vi "TL_XY_PFS_sCMOS_v8.vi"() -> ()   [LabVIEW 2013]
uses:
  <vilib>/Analysis/Matrix/Datatypes/RealMatrix.ctl
  <vilib>/Platform/TimedLoop/XDataNode/timing_clust.ctl
  <vilib>/Platform/TimedLoop/XDataNode/nitl_modes.ctl
  <vilib>/Platform/TimedLoop/XDataNode/wakeup.ctl
  <vilib>/DAQmx/read.llb/DAQmx Read (Analog DBL 1Chan 1Samp).vi
  <vilib>/DAQmx/write.llb/DAQmx Write (Analog DBL 1Chan 1Samp).vi
  <vilib>/DAQmx/write.llb/DAQmx Write (Digital 1D Bool 1Chan 1Samp).vi
  <vilib>/DAQmx/create/channels.llb/DAQmx Create Channel (AO-Voltage-Basic).vi
  <vilib>/DAQmx/create/channels.llb/DAQmx Create Channel (DO-Digital Output).vi
  <vilib>/Platform/TimedLoop/scheduler/LVUserAPI/_suppVIs/Create_1kHz_TSource.vi
  <vilib>/DAQmx/create/channels.llb/DAQmx Create Channel (AI-Voltage-Basic).vi
  <vilib>/DAQmx/miscellaneous.llb/DAQmx Fill In Error Info.vi
  <vilib>/Analysis/Matrix/Numeric/Conversions/Array To Matrix - RA.vi
  <vilib>/Platform/TimedLoop/XDataNode/XDataNode.xnode
  <vilib>/Platform/TimedLoop/XDataNode/XDNodeRunTimeDep.lvlib
  <vilib>/Analysis/Matrix/NI_Matrix.lvlib
panel:
  out "lastgoodz_list":T1
  in  "Delay after Fluo. cube change":u32=500
  in  "Delay PFS":u32=500
  out "lastgoodz":i32
  out "PFS status":i32
  in  "Delay after Move":u32=500
  out "TL_NPOS":u32 caption="Number of\nPositions"
  out "Laser Power (a.u.)":dbl=50.0 format="%05_2f"
  out "FlowRate (mL/min)":dbl=50.0 format="%05_2f"
  in  "Min. Scan duration":dbl
  out "TL Fluidic SYNC":bool caption="Fluidic SYNC"
  out "softversion":string
  in  "config Name":string="your_config"
  in  "Load Config":bool
  in  "Save Config":bool
  in  "Config Directory":path=path "D:/CONFIG_TIME_LAPSE"
  out "TL Laser shutter":bool caption="L. shutter"
  out "Next Pattern":u8(slide) scale=0.0..100.0
  out "Recorded\nPatterns":u32
  out "Ready":bool
  in  "stop the program":bool
  out "Current Position":u32
  out "Y position (µm)":dbl
  out "X position (µm)":dbl
  in  "storeXY Position":bool
  in  "stage speed (mm/s)":sgl=5.0 min=0.1 max=5 step=0.1
  in  "Stage COM PORT":refnum<visa-resource-name>="COM1"
  out "Next Scan":u8(slide) scale=0.0..100.0
  in  "Frames between Scan":u32
  out "Recorded Scans":u32
  in  "Total Number of Scan":u32=150 step=1
  out "TLON":bool
  in  "pause TL":bool
  in  "startTL":bool
  in  "Lower Filter":u8=1 min=1 max=6 step=1
  out "Buffer Info":T2
  out "Version":string
  out "Camera Serial":string
  out "Camera Model":string
  in  "Binning":u16=1 max=4 step=1
  out "zinit":i32
  in  "file name motif":string="image"
  out "SavedImages":i32
  out "Next Image Name":string
  out "Z position":dbl
  in  "error in (no error)":errorcluster
  out "Read Out Time":dbl=50.0
  in  "RO Mode":u32 max=2 step=1
  out "Imtemp":u16[][](array[numeric])
  in  "savelast":bool
  in  "Current Directory":path=path "D:/DATA_Par_Dates"
  in  "Exposure Time":dbl=0.1 min=0.0 max=10.0 step=9.999999747378752e-06
  in  "Time between Images (Free Run)":u32 caption="delay"
  in  "LASER shutter":bool
  in  "Free Run":bool
  in  "Commande onglets":T3(tab)
  out "Intensity Graph":u16[][](graph)
  in  "RESET ALL\nChanels":bool
  in  "ADD\nChanel":bool
  out "used Filters":u8[](array[numeric])
  out "used LEDs":bool[][](array[boolean])
  in  "LED-0":bool
  in  "LED-1":bool
  in  "LED-2":bool
  in  "LED-3":bool
  in  "LED-4":bool
  in  "LED-5":bool
  in  "Filter selection":u8(ring)=1 items=["1"=1, "2"=2, "3"=3, "4"=4, "5"=5, "6"=6]
  in  "LED-6":bool
  in  "LED-7":bool
  in  "LED-8":bool
  in  "LED-9":bool
  in  "LED-10":bool
  in  "LED-11":bool
  out "TL_NCAN":u8
  in  "Generate\nPositions":bool
  out "Field\nHeigth (µm)":dbl
  out "Field\nWidth (µm)":dbl
  out "stored XY":T1
  in  "re-SET ALL\nPositions":bool
  in  "XY positions path":path
  in  "Loadpositions":bool
  out "Scanning Motif":T4(graph)
  in  "Microscope Objective\nMagnification":dbl=60.0 min=1.0 max=1000.0 step=1.0
  in  "Method":u8(ring) items=["Spiral Scan", "Column Scan", "Line Scan"]
  in  "Spacing X (µm)":dbl=100.0 step=0.001
  in  "Spacing Y (µm)":dbl=100.0 step=0.001
  in  "Number\nof\nPositions":u32=40
  in  "Position to add":u32=30 step=1
  in  "Noff":u32 step=1
  in  "Non":u32=150 step=1
  in  "Nstart":u32=30 step=1
  in  "Frames between Patterns":u32
  in  "Total Number of Patterns":u32=1 step=1
  in  "is_single_shoot":bool caption="SingleShoot/TemporalPattern"
  in  "Shoot duration":dbl=1.0 step=1.0
  out "shooted_ positions":bool[][](array[boolean])
  in  "ADD\nPosition":bool
  in  "ADD ALL\nPositions":bool
  in  "RESET POS":bool
  out "shoot_list":T1
  in  "Shoot at Scan#":i32=1 step=1
  in  "useLASER_TL":bool caption="use LASER"
  in  "Noff FLUIDICS":u32 caption="Noff" step=1
  in  "Non FLUIDICS":u32=150 caption="Non" step=1
  in  "Nstart FLUIDICS":u32=30 caption="Nstart" step=1
  in  "useFLUIDICS_TL":bool caption="use LASER"
  # "XY stage"
  # "(µm)"
  # "Camera Settings"
  # "(s)"
  # "(s)"
  # "Time Lapse"
  # "Timming Settings"
  # "(s)"
  # "(ms)"
  # "(ms)"
  # "(ms)"
  # "Set a Illumination Pattern"
  # "Number of Channels"
  # "Light Sources to use"
  # "340\nnm"
  # "365\nnm"
  # "405\nnm"
  # "455\nnm"
  # "490\nnm"
  # "505\nnm"
  # "565\nnm"
  # "590\nnm"
  # "625\nnm"
  # "680\nnm"
  # "730\nnm"
  # "Bright\nField"
  # "0"
  # "1"
  # "2"
  # "Channel   #"
  # "3"
  # "4"
  # "5"
  # "6"
  # "7"
  # "8"
  # "Stored Positions"
  # "SingleShoot Mode"
  # "TemporalPattern Mode"
  # "Timming"
  # "Timming"
  # "(s)"
  # "FLUIDIC Switch Timming (SCAN Mode)"
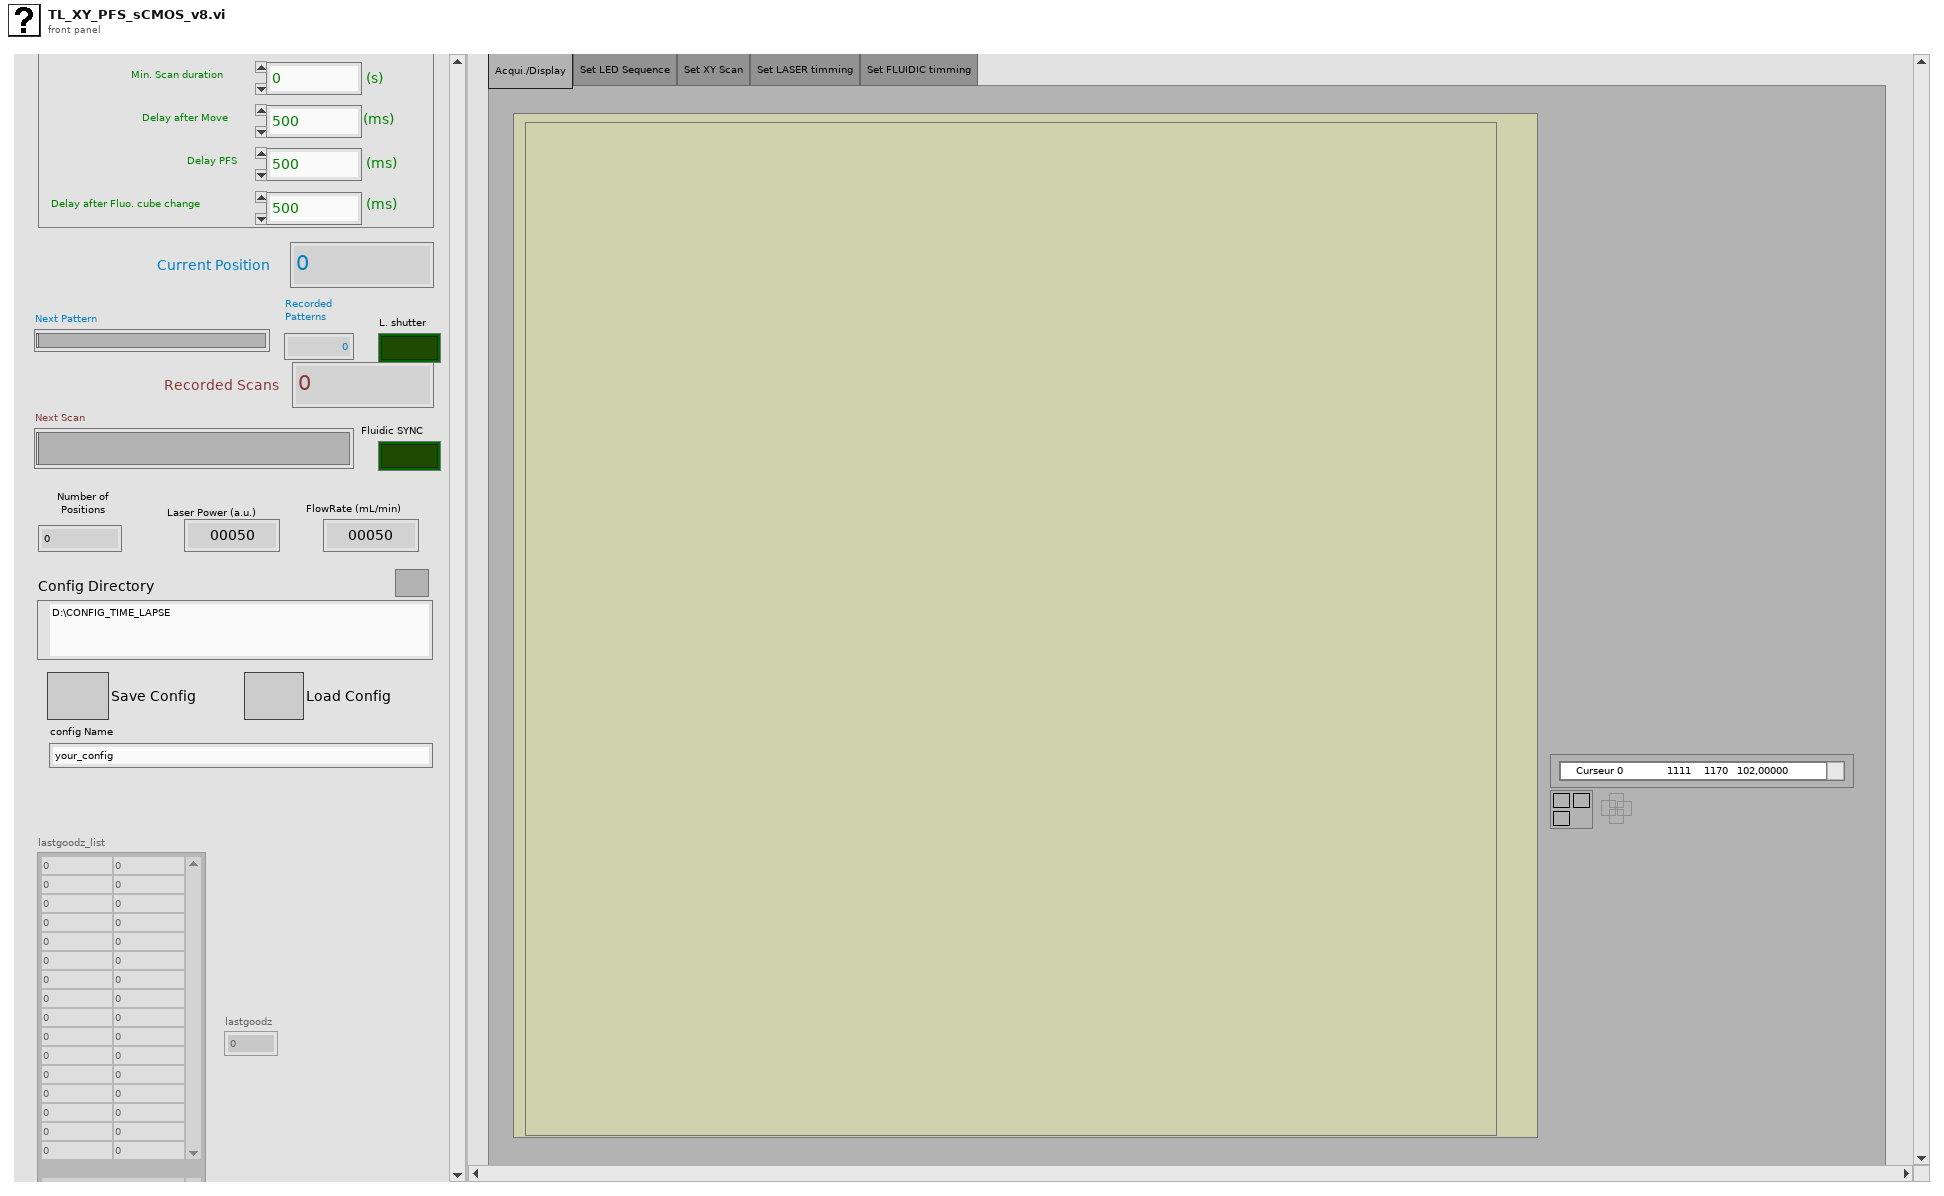
[diagram p1: front panel]
types:
  T1 = typedef "NI_Matrix.lvlib/RealMatrix.ctl" = dbl[][]
  T2 = cluster{"height":u32, "width":u32, "datatype":u32}
  T3 = enum32{"Acqui./Display", "Set LED Sequence", "Set XY Scan", "Set LASER timming", "Set FLUIDIC timming"}
  T4 = cluster{cluster{"Real Matrix Element":dbl, "Real Matrix Element":dbl}[]}[]
  T5 = cluster{"Model":string, "Camera ID":string, "Firmware":string}
  T6 = cluster{"Mode":u32, "Polarity":u32, "Times":u32, "Delay":dbl}
  T7 = typedef "XDNodeRunTimeDep.lvlib/timing_clust.ctl" = cluster{"Expected End [f-1]":u64, "Actual End [f-1]":u64, "Finished Late? [f-1]":bool, "Expected End [i-1]":u64, "Actual End [i-1]":u64, "Finished Late? [i-1]":bool, "Expected Start [i]":u64, "Actual Start [i]":u64, "Expected Start [f]":u64, "Actual Start [f]":u64, "Source Name":string, "Structure Name":string, "Period":i64, "Deadline":i64, "Offset":i64, "Start":i64, "Priority":i32, "Timeout":i32, "Mode":T8, "Wakeup Reason":T9, "Error":errorcluster, "Source Type":string, "Secondary Source Type":string, "Global End Time":u64, "Global Start Time":u64, "Frame Duration":u64, "Iteration Duration":u64, "Assigned CPU":i32, "I/O Scan Engine Mode":u32}
  T8 = typedef "XDNodeRunTimeDep.lvlib/nitl_modes.ctl" = enum32{"No Change", "Process missed periods, maintain original phase", "Discard missed periods, maintain original phase", "Process missed periods, ignore original phase", "Discard missed periods, ignore original phase"}
  T9 = typedef "XDNodeRunTimeDep.lvlib/wakeup.ctl" = enum32{"Normal", "Aborted", "Asynchronous wakeup", "Timing source error", "Timed loop error", "Timeout"}
  T10 = typedef "Image Type" = u32
  T11 = typedef "IMAQ Image.ctl" = refnum<image>
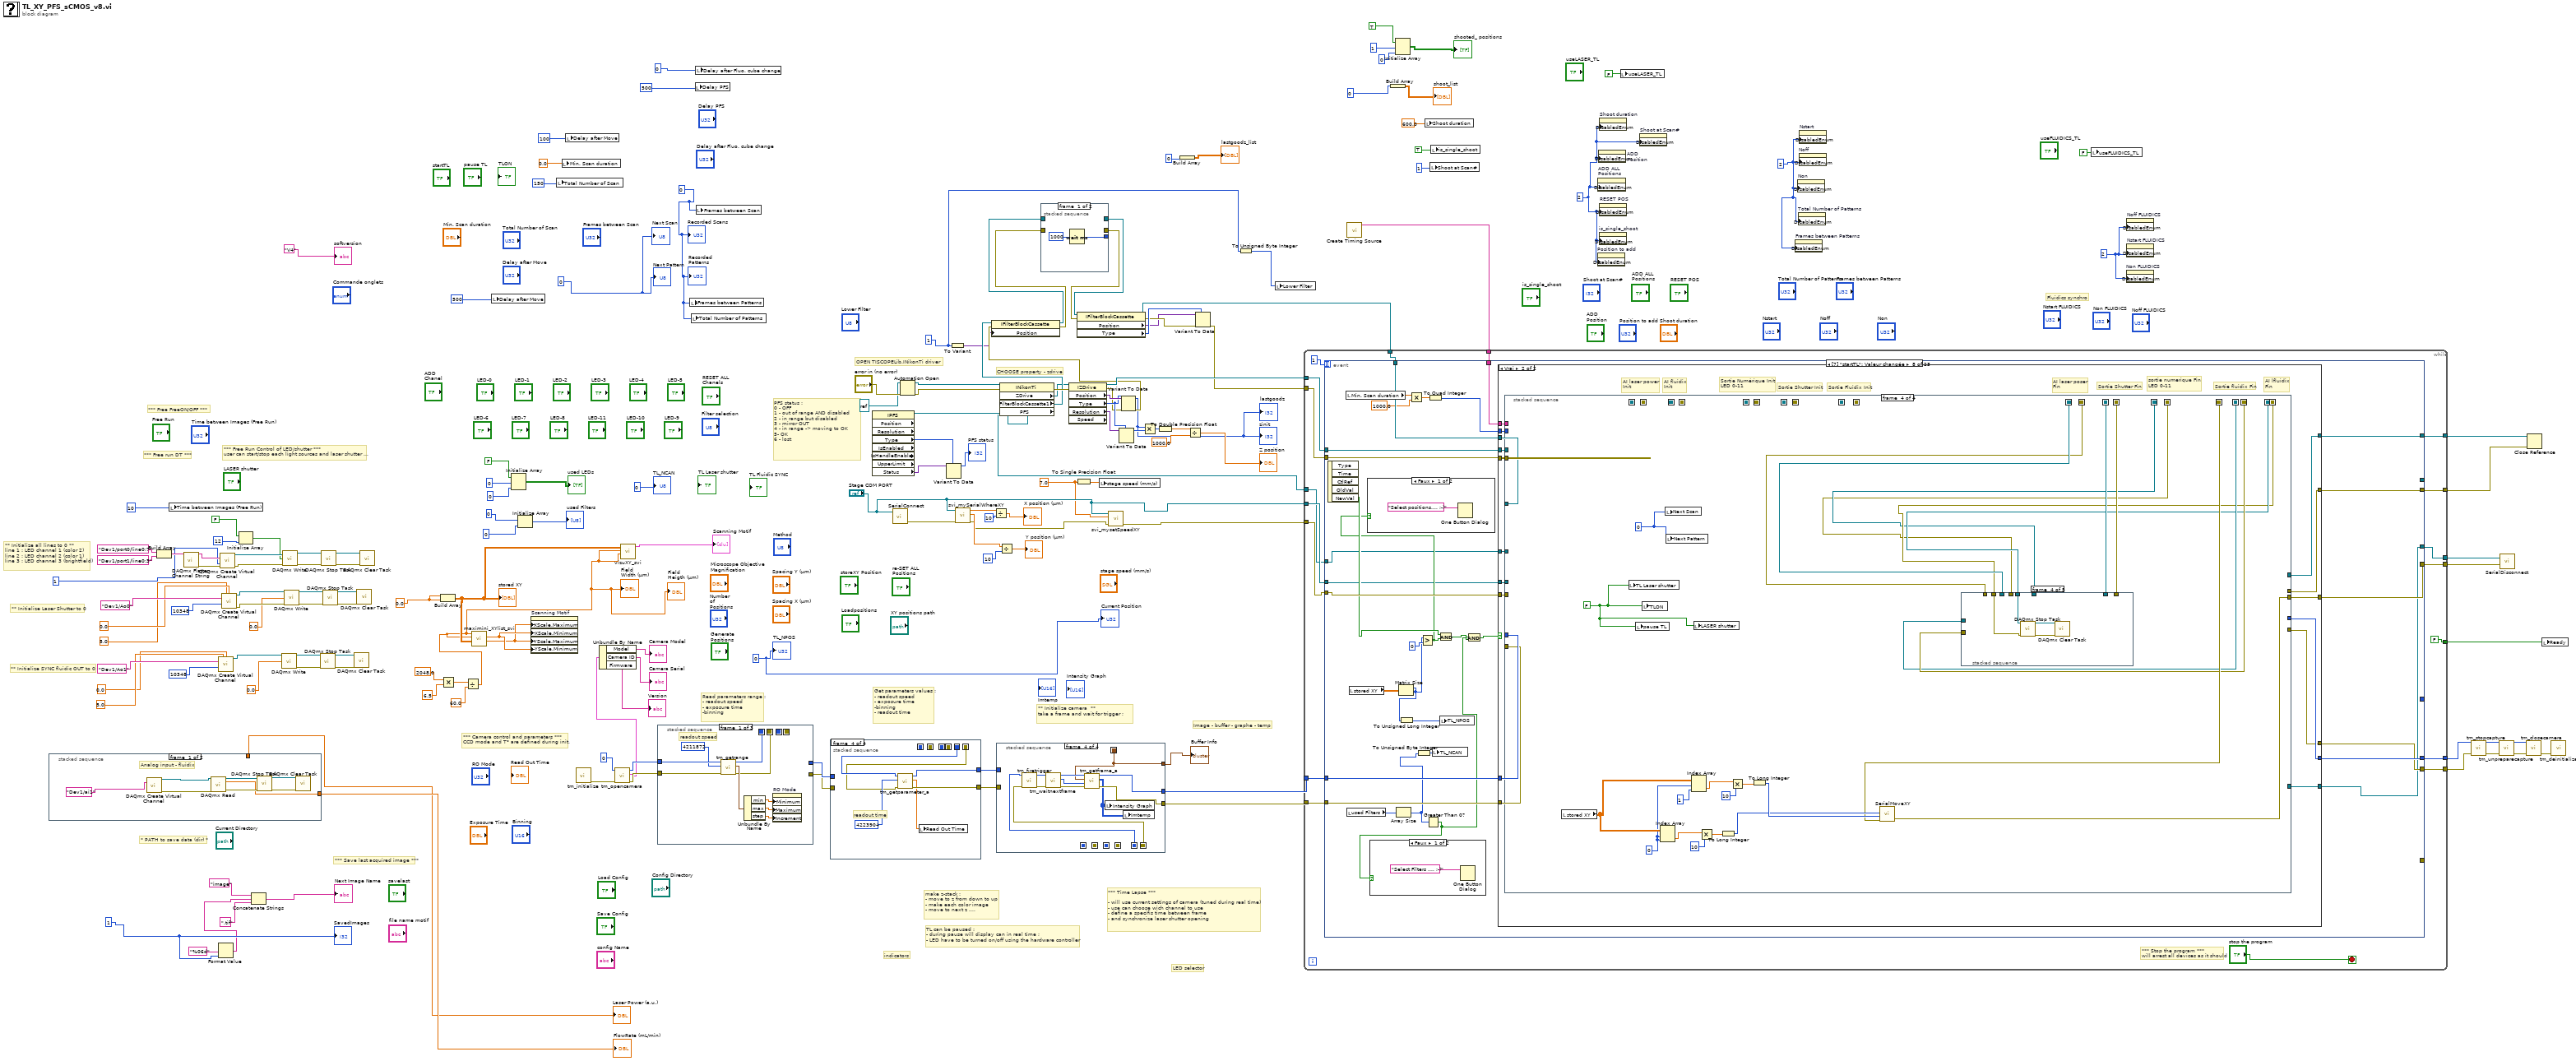
[diagram p0: block diagram]
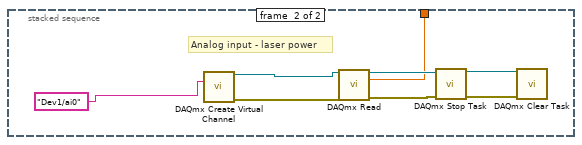
[diagram p2: hidden frame]
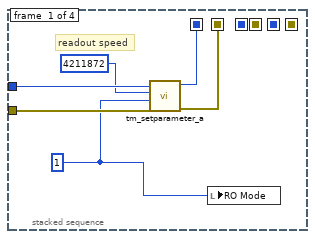
[diagram p4: hidden frame]
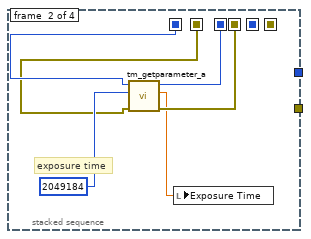
[diagram p5: hidden frame]
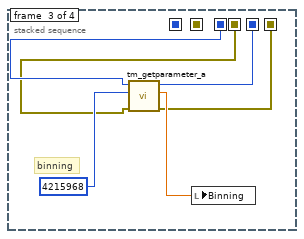
[diagram p6: hidden frame]
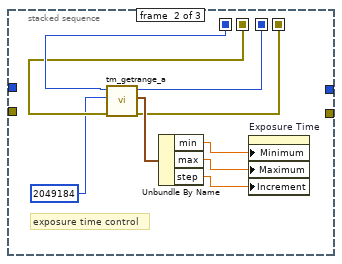
[diagram p7: hidden frame]
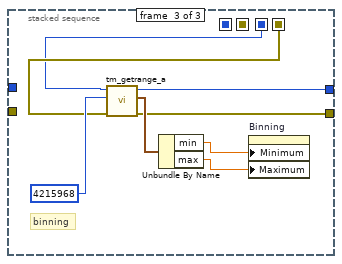
[diagram p8: hidden frame]
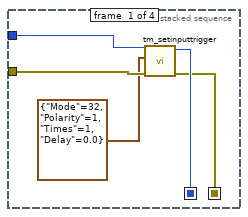
[diagram p9: hidden frame]
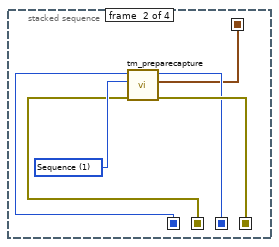
[diagram p10: hidden frame]
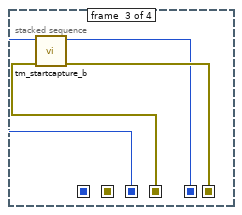
[diagram p11: hidden frame]
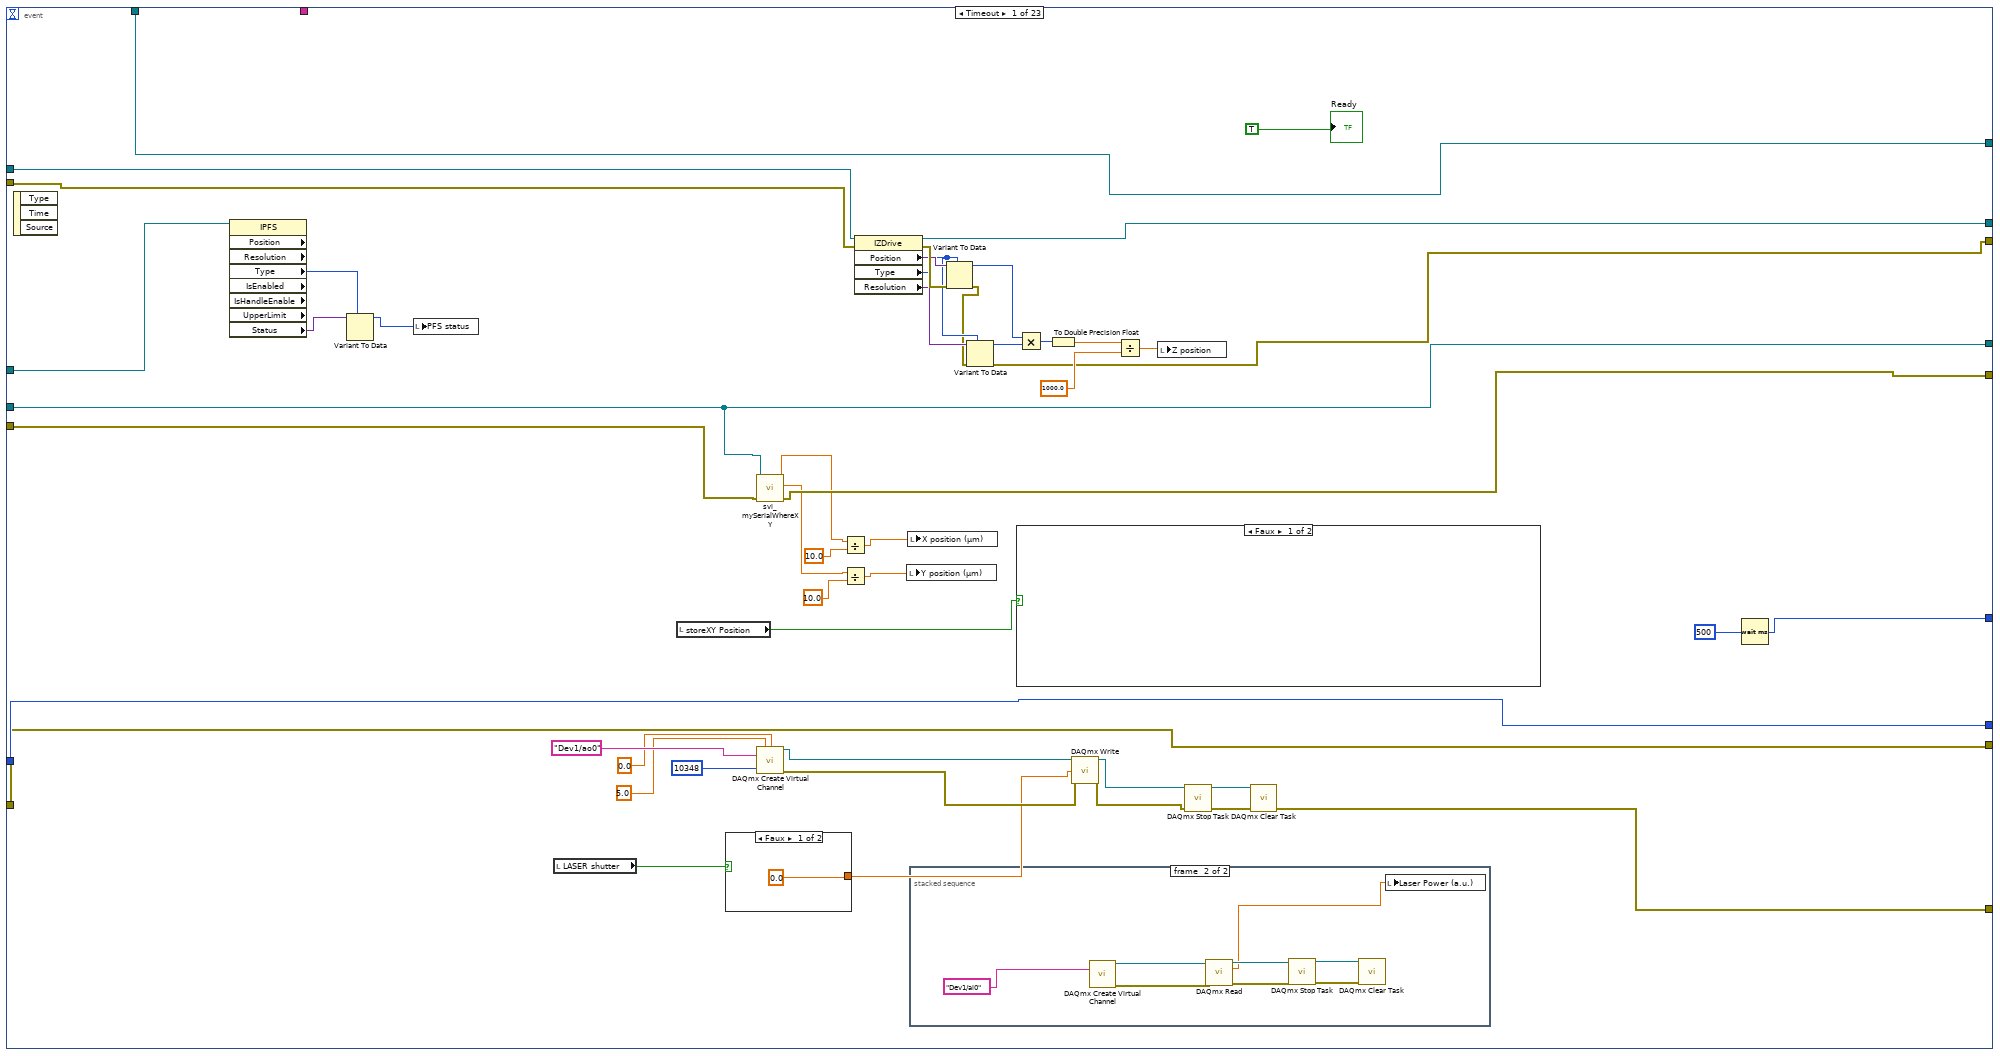
[diagram p12: hidden frame]
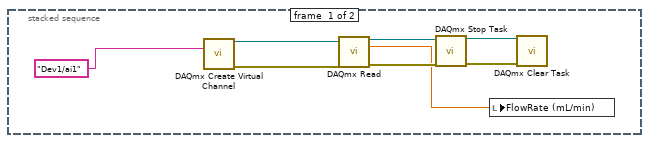
[diagram p13: hidden frame]
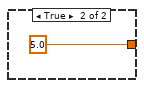
[diagram p14: hidden frame]
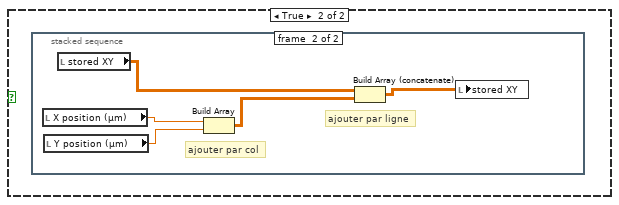
[diagram p15: hidden frame]
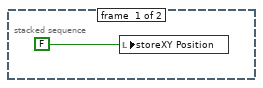
[diagram p16: hidden frame]
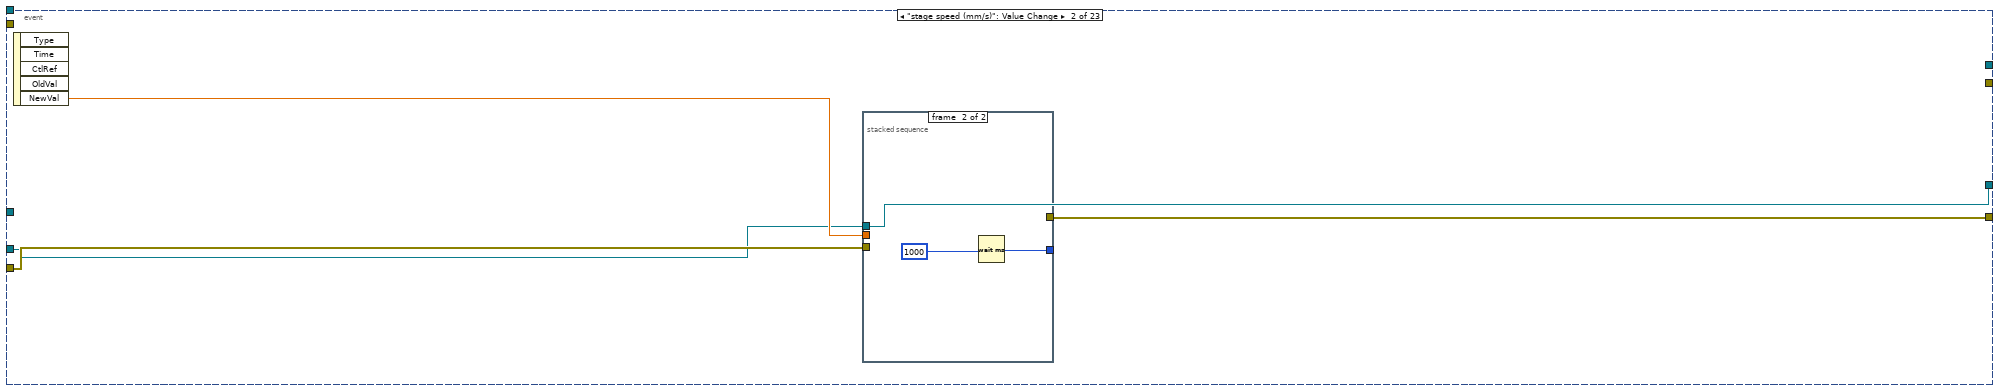
[diagram p17: hidden frame]
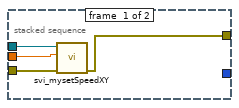
[diagram p18: hidden frame]
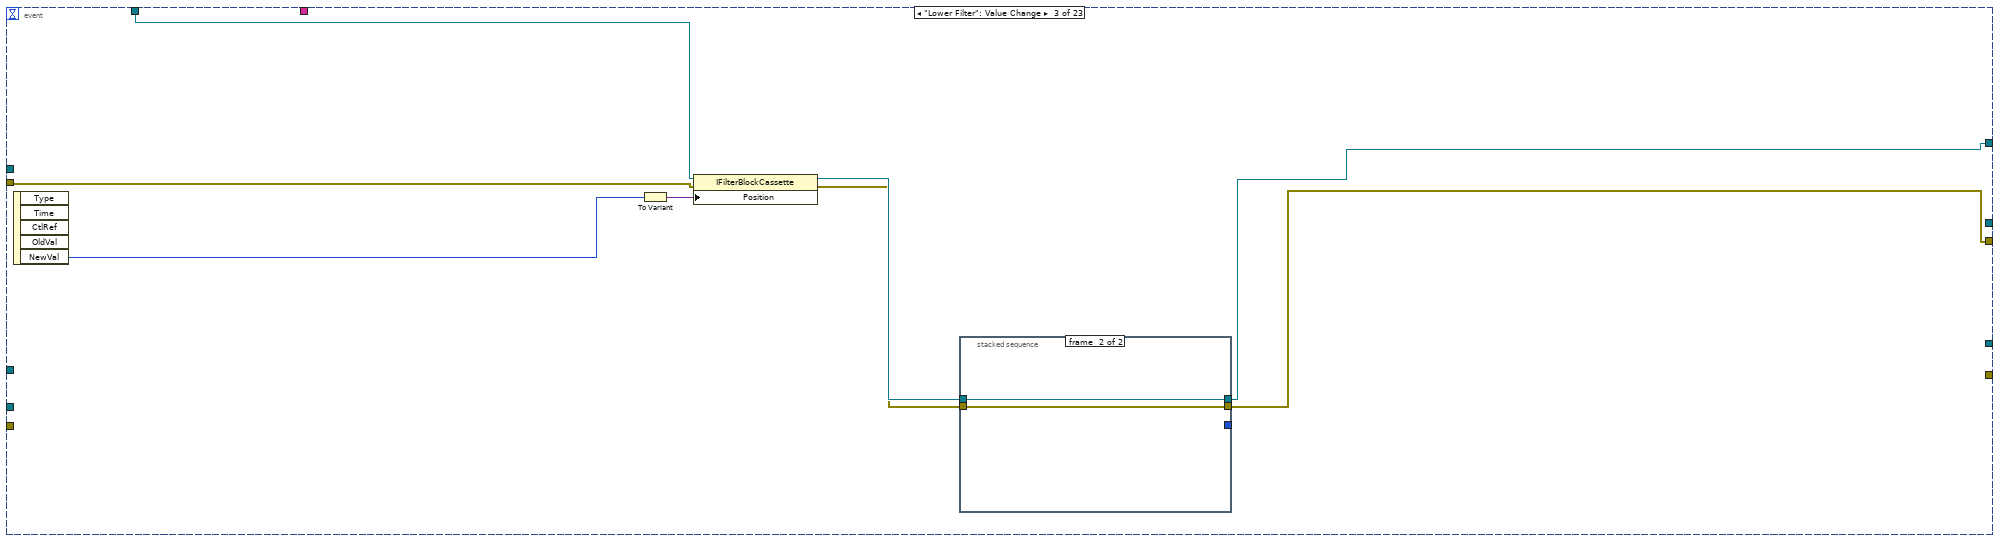
[diagram p19: hidden frame]
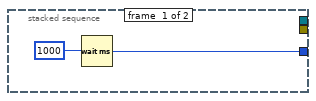
[diagram p20: hidden frame]
diagram:
  w16 = u8 2
  w15 = u8 2
  w24 = u8 2
  w56 = 0
  w58 = u32 0
  w59 = u8 0
  w60 = 0.0
  w92 = 7.0
  w41 = 1
  w132 = 1
  # "PFS status :\n0 - OFF\n1 - out of range AND disabled\n2 - in range but disabled\n3 - mirror OUT\n4 - in range -> moving to OK\n5- OK\n6 - lost"
  # "Fluidics synchro"
  # "** Initialize SYNC fluidic OUT to 0"
  # "** Initialize Laser Shutter to 0"
  # "* PATH to save data (dir) *"
  # "Image - buffer - graphe - temp"
  # "Get parameters values :\n- readout speed\n- exposure time\n-binning\n- readout time"
  # "Read parameters range :\n- readout speed\n- exposure time\n-binning"
  # "CHOOSE property - zdrive"
  # "OPEN TISCOPELib.INikonTi driver"
  # "indicators"
  # "LED selector"
  # "TL can be paused :\n- during pause will display can in real time ;\n- LED have to be turned on/off using the hardware controller"
  # "make z-stack :\n- move to z from down to up\n- make each color image\n- move to next z ...."
  # "*** Time Lapse ***\n\n- will use current settings of camera (tuned during real time)\n- use can choose wich channel to use\n- define a specifis time between frame\n- and synchronize laser shutter opening"
  # "*** Camera control and parameters ***\nCCD mode and T° are defined during init."
  # "*** Save last acquired image ***"
  # "** Initialize camera  **\ntake a frame and wait for trigger ;"
  # "** Initialize all lines to 0 **\nline 1 : LED channel 1 (color 2)\nline 2 : LED channel 2 (color 1)\nline 3 : LED channel 3 (brightfield)"
  # "*** Free FreeON/OFF ***"
  # "*** Free run DT ***"
  # "*** Free Run Control of LED/shutter ***\nuser can start/stop each light sources and laser shutter ..."
  n1 = stacked-sequence {
    tunnel: [w166 _] -> w20
    tunnel: [_ w174] -> w13
    frame #0 {
      # "Analog input - fluidix"
      n2 = call-poly <vilib>:"DAQmx Create Virtual Channel.vi"("physical channels"="Dev1/ai1") -> ("task out"=w173:refnum<k21>, "error out"=w172:errorcluster)  [unwired: 13 in]
      n3 = call-poly <vilib>:"DAQmx Read.vi"("task/channels in"=w173, "error in"=w172) -> ("task out"=w170:refnum<k21>, "data"=w166:dbl, "error out"=w171:errorcluster)  [unwired: 11 in]
      n4 = call <vilib>:"DAQmx Stop Task.vi"("task/channels in"=w170, "error in"=w171) -> ("task out"=w168:refnum<k21>, "error out"=w169:errorcluster)  [unwired: 12 in]
      n5 = call <vilib>:"DAQmx Clear Task.vi"("task in"=w168, "error in"=w169) -> ()  [unwired: 13 in, 1 out]
    }
    frame #1 {
      # "Analog input - laser power"
      n6 = call-poly <vilib>:"DAQmx Create Virtual Channel.vi"("physical channels"="Dev1/ai0") -> ("task out"=w175:refnum<k21>, "error out"=w176:errorcluster)  [unwired: 13 in]
      n7 = call-poly <vilib>:"DAQmx Read.vi"("task/channels in"=w175, "error in"=w176) -> ("task out"=w178:refnum<k21>, "data"=w174:dbl, "error out"=w177:errorcluster)  [unwired: 11 in]
      n8 = call <vilib>:"DAQmx Stop Task.vi"("task/channels in"=w178, "error in"=w177) -> ("task out"=w180:refnum<k21>, "error out"=w179:errorcluster)  [unwired: 12 in]
      n9 = call <vilib>:"DAQmx Clear Task.vi"("task in"=w180, "error in"=w179) -> ()  [unwired: 13 in, 1 out]
    }
  }
  "Laser Power (a.u.)" <- w13
  "FlowRate (mL/min)" <- w20
  n10 = Build Array("Dev1/port0/line0:7", "Dev1/port1/line0:3") -> (w83:string[])
  n11 = local write "Time between Images (Free Run)"(10) -> ()
  n12 = call <vilib>:"DAQmx Flatten Channel String.vi"("names in"=w83) -> ("names out"=w82:string, "error out"=w84:errorcluster)  [unwired: 13 in]
  n13 = Format Value(format string="%06d", value (0)=w132) -> (output string=w131:string)  [unwired: 1 in]
  n14 = call-poly <vilib>:"DAQmx Create Virtual Channel.vi"("maximum value"=5.0, "minimum value"=0.0, "physical channels"="Dev1/Ao1", "units"=10348) -> ("task out"=w38:refnum<k21>)  [unwired: 10 in, 1 out]
  n15 = call-poly <vilib>:"DAQmx Create Virtual Channel.vi"("lines"=w82, "line grouping"=1, "error in"=w84) -> ("task out"=w164:refnum<k21>, "error out"=w163:errorcluster)  [unwired: 11 in]
  n16 = call-poly <vilib>:"DAQmx Create Virtual Channel.vi"("maximum value"=5.0, "minimum value"=0.0, "physical channels"="Dev1/Ao0", "units"=10348) -> ("task out"=w80:refnum<k21>, "error out"=w79:errorcluster)  [unwired: 10 in]
  n17 = Initialize Array(FALSE, 12) -> (w109:bool[])
  n18 = Concatenate Strings("image", w131, ".tif") -> (→"Next Image Name":string)
  n19 = call-poly <vilib>:"DAQmx Write.vi"("task/channels in"=w38, "data"=0.0) -> ("task out"=w37:refnum<k21>, "error out"=w36:errorcluster)  [unwired: 11 in, 1 out]
  n20 = call-poly <vilib>:"DAQmx Write.vi"("task/channels in"=w164, "data"=w109, "error in"=w163) -> ("task out"=w162:refnum<k21>, "error out"=w160:errorcluster)  [unwired: 10 in, 1 out]
  n21 = call-poly <vilib>:"DAQmx Write.vi"("task/channels in"=w80, "data"=0.0, "error in"=w79) -> ("task out"=w76:refnum<k21>, "error out"=w77:errorcluster)  [unwired: 10 in, 1 out]
  n22 = call <vilib>:"DAQmx Stop Task.vi"("task/channels in"=w37, "error in"=w36) -> ("task out"=w34:refnum<k21>, "error out"=w35:errorcluster)  [unwired: 12 in]
  n23 = call <vilib>:"DAQmx Stop Task.vi"("task/channels in"=w162, "error in"=w160) -> ("task out"=w161:refnum<k21>, "error out"=w159:errorcluster)  [unwired: 12 in]
  n24 = call <vilib>:"DAQmx Stop Task.vi"("task/channels in"=w76, "error in"=w77) -> ("task out"=w75:refnum<k21>, "error out"=w74:errorcluster)  [unwired: 12 in]
  n25 = call <vilib>:"DAQmx Clear Task.vi"("task in"=w34, "error in"=w35) -> ()  [unwired: 13 in, 1 out]
  n26 = call <vilib>:"DAQmx Clear Task.vi"("task in"=w75, "error in"=w74) -> ()  [unwired: 13 in, 1 out]
  n27 = call <vilib>:"DAQmx Clear Task.vi"("task in"=w161, "error in"=w159) -> ()  [unwired: 13 in, 1 out]
  n28 = Build Array(w60, w60) -> (w52:T1)
  "stored XY" <- w52
  n29 = Multiply(x=2048.0, y=6.5) -> (x*y=w48:dbl)
  n30 = Divide(x=w48, y=60.0) -> (x/y=w47:dbl)
  "Field\nWidth (µm)" <- w47
  "Field\nHeigth (µm)" <- w47
  n31 = call "maximini_XYlist_svi.vi"("stored XY"=w52, "LY"=w47, "LX"=w47) -> ("mini (µm)"=w54:dbl, "maxi (µm)"=w53:dbl)  [unwired: 7 in]
  n32 = local write "Delay after Move"(u32 500) -> ()
  n33 = Initialize Array(FALSE, 0, 0) -> (→"used LEDs":bool[][])
  n34 = Initialize Array(u8 0, 0) -> (→"used Filters":u8[])
  n35 = property on="Scanning Motif" class="GraphXY (strict)"("XScale.Maximum"=w53, "XScale.Minimum"=w54, "YScale.Maximum"=w53, "YScale.Minimum"=w54) -> ()  [unwired: 2 in, 2 out]
  n36 = local write "Total Number of Scan"(u32 150) -> ()
  n37 = local write "Min. Scan duration"(0.0) -> ()
  n38 = local write "Delay after Move"(u32 100) -> ()
  n39 = call <userlib>:"tm_initialize.vi"() -> ("error out"=w158:errorcluster)  [unwired: 1 in, 10 out]
  n40 = call <userlib>:"tm_opencamera.vi"("error in (no error)"=w158, "Camera Index"=u32 0) -> ("error out"=w129:errorcluster, "Camera Details"=w119:T5, "Handle out"=w130:u32)  [unwired: 1 in, 6 out]
  n41 = Unbundle By Name(w119) -> ("Model"=→"Camera Model":string, "Camera ID"=→"Camera Serial":string, "Firmware"=→"Version":string)
  n42 = call "vizuXY_svi.vi"("LY (mm)"=w47, "LX (mm)"=w47, "stored XY (µm)"=w52) -> ("Tableau"=→"Scanning Motif":T4)  [unwired: 8 in]
  n43 = stacked-sequence {
    seq-local: [w183 _ _] -> [_ w199 _]
    seq-local: [w182 _ _] -> [_ w198 _]
    seq-local: [_ w192 _] -> [_ _ w203]
    seq-local: [_ w191 _] -> [_ _ w204]
    tunnel: w130 -> [w190 _ _]
    tunnel: w129 -> [w189 _ _]
    tunnel: [_ _ w202] -> w128
    tunnel: [_ _ w201] -> w127
    frame #0 {
      # "readout speed"
      n44 = call <userlib>:"tm_getrange.vi"("error in (no error)"=w189, "Parameter"=4211872, "Handle in"=w190) -> ("error out"=w182:errorcluster, "Range"=w187:cluster{"min":dbl, "max":dbl, "step":dbl}, "Handle out"=w183:u32)  [unwired: 6 out]
      n45 = Unbundle By Name(w187) -> ("min"=w186:dbl, "max"=w185:dbl, "step"=w184:dbl)
      n46 = property on="RO Mode" class="NumNb (strict)"("Minimum"=w186, "Maximum"=w185, "Increment"=w184) -> ()  [unwired: 2 in, 2 out]
    }
    frame #1 {
      # "exposure time control"
      n47 = call <userlib>:"tm_getrange_a.vi"("error in (no error)"=w198, "Parameter"=2049184, "Handle in"=w199) -> ("error out"=w191:errorcluster, "Range"=w197:cluster{"min":dbl, "max":dbl, "step":dbl}, "Handle out"=w192:u32)  [unwired: 2 in, 4 out]
      n48 = Unbundle By Name(w197) -> ("min"=w196:dbl, "max"=w195:dbl, "step"=w194:dbl)
      n49 = property on="Exposure Time" class="NumNb (strict)"("Minimum"=w196, "Maximum"=w195, "Increment"=w194) -> ()  [unwired: 2 in, 2 out]
    }
    frame #2 {
      # "binning"
      n50 = call <userlib>:"tm_getrange_a.vi"("error in (no error)"=w204, "Parameter"=4215968, "Handle in"=w203) -> ("error out"=w201:errorcluster, "Range"=w207:cluster{"min":dbl, "max":dbl, "step":dbl}, "Handle out"=w202:u32)  [unwired: 2 in, 4 out]
      n51 = Unbundle By Name(w207) -> ("min"=w200:dbl, "max"=w206:dbl)
      n52 = property on="Binning" class="NumNb (strict)"("Minimum"=w200, "Maximum"=w206) -> ()  [unwired: 2 in, 2 out]
    }
  }
  n53 = local write "Frames between Patterns"(w58) -> ()
  n54 = local write "Total Number of Patterns"(w58) -> ()
  n55 = local write "Delay PFS"(u32 500) -> ()
  n56 = local write "Delay after Fluo. cube change"(u32 0) -> ()
  n57 = local write "Frames between Scan"(w58) -> ()
  n58 = stacked-sequence {
    seq-local: [w210 _ _ _] -> [_ w218 _ _]
    seq-local: [w209 _ _ _] -> [_ w217 _ _]
    seq-local: [_ w216 _ _] -> [_ _ w223 _]
    seq-local: [_ w215 _ _] -> [_ _ w222 _]
    seq-local: [_ _ w221 _] -> [_ _ _ w230]
    seq-local: [_ _ w220 _] -> [_ _ _ w229]
    tunnel: w128 -> [w213 _ _ _]
    tunnel: w127 -> [w212 _ _ _]
    tunnel: [_ _ _ w228] -> w126
    tunnel: [_ _ _ w227] -> w125
    frame #0 {
      w208 = 1
      # "readout speed"
      n59 = call <userlib>:"tm_setparameter_a.vi"("error in (no error)"=w212, "Value in"=w208, "Parameter"=4211872, "Handle in"=w213) -> ("error out"=w209:errorcluster, "Handle out"=w210:u32)  [unwired: 6 in]
      n60 = local write "RO Mode"(w208) -> ()
    }
    frame #1 {
      # "exposure time"
      n61 = call <userlib>:"tm_getparameter_a.vi"("error in (no error)"=w217, "Parameter"=2049184, "Handle in"=w218) -> ("error out"=w215:errorcluster, "Value out"=w214:dbl, "Handle out"=w216:u32)  [unwired: 6 in]
      n62 = local write "Exposure Time"(w214) -> ()
    }
    frame #2 {
      # "binning"
      n63 = call <userlib>:"tm_getparameter_a.vi"("error in (no error)"=w222, "Parameter"=4215968, "Handle in"=w223) -> ("error out"=w220:errorcluster, "Value out"=w224:dbl, "Handle out"=w221:u32)  [unwired: 6 in]
      n64 = local write "Binning"(w224) -> ()
    }
    frame #3 {
      # "readout time"
      n65 = call <userlib>:"tm_getparameter_a.vi"("error in (no error)"=w229, "Parameter"=4223904, "Handle in"=w230) -> ("error out"=w227:errorcluster, "Value out"=w226:dbl, "Handle out"=w228:u32)  [unwired: 6 in]
      n66 = local write "Read Out Time"(w226) -> ()
    }
  }
  n67 = call "SerialConnect.vi"("VISA resource name"="Stage COM PORT") -> ("error out"=w108:errorcluster)  [unwired: 4 in]
  n68 = Automation Open(error in (no error)="error in (no error)", Automation Refnum=refnum<k7> refnum ("TISCOPELib.INikonTi")) -> (Automation Refnum=w145:refnum<k7>, error out=w144:errorcluster)  [unwired: 2 out]
  n69 = To Variant(anything=w41) -> (Variant=w110:variant)
  n70 = call "svi_mySerialWhereXY.vi"("entrée d'erreur (pas d'erreur)"=w108, "Refnum VISA en entrée"="Stage COM PORT") -> ("sortie d'erreur"=w101:errorcluster, "Y"=w104:dbl, "X"=w107:dbl)  [unwired: 7 in]
  n71 = Divide(x=w107, y=10) -> (x/y=→"X position (µm)":dbl)
  n72 = stacked-sequence {
    seq-local: [w233 _ _ _] -> [_ w241 _ _]
    seq-local: [w232 _ _ _] -> [_ w240 _ _]
    seq-local: [_ w238 _ _] -> [_ _ w246 _]
    seq-local: [_ w239 _ _] -> [_ _ w245 _]
    seq-local: [_ _ w243 _] -> [_ _ _ w255]
    seq-local: [_ _ w244 _] -> [_ _ _ w254]
    seq-local: [_ w237 _ _] -> [_ _ _ w248]
    tunnel: w126 -> [w236 _ _ _]
    tunnel: w125 -> [w235 _ _ _]
    tunnel: [_ _ _ w250] -> w124
    tunnel: [_ _ _ w249] -> w123
    tunnel: [_ _ _ w248] -> w152
    frame #0 {
      n73 = call <userlib>:"tm_setinputtrigger.vi"("error in (no error)"=w235, "Parameters"=T6 {"Mode"=32, "Polarity"=1, "Times"=1, "Delay"=0.0}, "Handle in"=w236) -> ("error out"=w232:errorcluster, "Handle out"=w233:u32)  [unwired: 7 in]
    }
    frame #1 {
      w242 = 1 items=["Snap", "Sequence"] ("Capture mode")
      n74 = call <userlib>:"tm_preparecapture.vi"("error in (no error)"=w240, "Capture mode"=w242, "Handle in"=w241) -> ("error out"=w239:errorcluster, "Buffer Info"=w237:T2, "Handle out"=w238:u32)  [unwired: 5 in, 1 out]
    }
    frame #2 {
      n75 = call <userlib>:"tm_startcapture_b.vi"("error in (no error)"=w245, "Handle in"=w246) -> ("error out"=w244:errorcluster, "Handle out"=w243:u32)  [unwired: 8 in]
    }
    frame #3 {
      n76 = call <userlib>:"tm_firetrigger.vi"("error in (no error)"=w254, "Handle in"=w255) -> ("error out"=w257:errorcluster, "Handle out"=w256:u32)  [unwired: 8 in]
      n77 = call <userlib>:"tm_waitnextframe.vi"("error in (no error)"=w257, "Handle in"=w256) -> ("error out"=w252:errorcluster, "Frame Index"=w251:i32, "Handle out"=w253:u32)  [unwired: 6 in, 1 out]
      n78 = call <userlib>:"tm_getframe_a.vi"("error in (no error)"=w252, "Frame Index"=w251, "Buffer Info"=w248, "Handle in"=w253) -> ("error out"=w249:errorcluster, "Data 16"=w247:u16[][], "Handle out"=w250:u32)  [unwired: 3 in, 2 out]
      n79 = local write "Intensity Graph"(w247) -> ()
      n80 = local write "Imtemp"(w247) -> ()
    }
  }
  "Buffer Info" <- w152
  n81 = Divide(x=w104, y=10) -> (x/y=→"Y position (µm)":dbl)
  n82 = property class="INikonTi"(reference=w145, error in=w144) -> (error out=w116:errorcluster, "ZDrive"=w89:refnum<k7>, "FilterBlockCassette1"=w112:refnum<k7>, "PFS"=w10:refnum<k7>)  [unwired: 1 out]
  n83 = property class="IPFS" props=["Position", "Resolution", "Type", "IsEnabled", "IsHandleEnable", "UpperLimit", "Status"](reference=w10) -> (reference out=w6:refnum<k7>, "Type"=w9:i32, "Status"=w7:variant)  [unwired: 1 in, 6 out]
  n84 = Variant To Data(type=w9, Variant=w7) -> (data=→"PFS status":i32)  [unwired: 1 in, 1 out]
  n85 = property class="IZDrive" props=["Position", "Type", "Resolution", "Speed"](reference=w89, error in=w116) -> (reference out=w143:refnum<k7>, error out=w139:errorcluster, "Position"=w142:variant, "Type"=w140:i32, "Resolution"=w141:variant)  [unwired: 1 out]
  n86 = To Single Precision Float(number=w92) -> (single precision float=w93:sgl)
  n87 = local write "stage speed (mm/s)"(w93) -> ()
  n88 = call "svi_mysetSpeedXY.vi"("entrée d'erreur (pas d'erreur)"=w101, "speed (mm/s)"=w92, "Refnum VISA en entrée"="Stage COM PORT") -> ("sortie d'erreur"=w99:errorcluster)  [unwired: 8 in]
  n89 = Variant To Data(type=w140, Variant=w141) -> (data=w138:i32)  [unwired: 1 in, 1 out]
  n90 = Variant To Data(error in=w139, type=w140, Variant=w142) -> (data=w5:i32, error out=w111:errorcluster)
  "zinit" <- w5
  "lastgoodz" <- w5
  n91 = property class="IFilterBlockCassette"(reference=w112, error in=w111, "Position"=w110) -> (reference out=w46:refnum<k7>, error out=w45:errorcluster)
  n92 = stacked-sequence {
    tunnel: [w258 _] -> _
    tunnel: w46 -> [_ w261]
    tunnel: w45 -> [_ w260]
    tunnel: [_ w261] -> w44
    tunnel: [_ w260] -> w43
    frame #0 {
      n93 = Wait (ms)(milliseconds to wait=1000) -> (millisecond timer value=w258:u32)
    }
    frame #1 {
    }
  }
  n94 = property class="IFilterBlockCassette"(reference=w44, error in=w43) -> (reference out=w115:refnum<k7>, error out=w117:errorcluster, "Position"=w113:variant, "Type"=w118:i32)
  n95 = Multiply(x=w5, y=w138) -> (x*y=w95:i32)
  n96 = To Double Precision Float(number=w95) -> (double precision float=w94:dbl)
  n97 = Build Array(0) -> (→"lastgoodz_list":T1)
  n98 = Divide(x=w94, y=1000.0) -> (x/y=→"Z position":dbl)
  n99 = Variant To Data(error in=w117, type=w118, Variant=w113) -> (error out=w64:errorcluster)  [unwired: 1 out]
  n100 = To Unsigned Byte Integer(number=w41) -> (unsigned 8bit integer=w90:u8)
  n101 = local write "Lower Filter"(w90) -> ()
  n102 = call-poly <vilib>:"Create Timing Source.vi"() -> ("name (out)"=w18:string)  [unwired: 10 in, 1 out]
  n103 = while {
    tunnel: [w277] -> w154
    tunnel: w124 -> [w276]
    tunnel: w123 -> [w275]
    tunnel: [w274] -> w153
    tunnel: w143 -> [w272]
    tunnel: w64 -> [w273]
    tunnel: [w271] -> w87
    tunnel: [FALSE] -> w134
    tunnel: w115 -> [w269]
    tunnel: [w268] -> w114
    tunnel: w99 -> [w267]
    tunnel: "Stage COM PORT" -> [w266]
    tunnel: [w265] -> w98
    tunnel: [w264] -> w97
    tunnel: w18 -> [w263]
    tunnel: w6 -> [w262]
    stop <- "stop the program" stop-if-true
    # "*** Stop the program ***\nwill arrest all devices as it should ..."
    n104 = event shown="[7] \"startTL\": Valeur changée" {
      selector: _ -> [_ _ _ _ _ _ _ _ _ _ _ _ _ _ _ _ _ _ _ _ _ _ _]
      dyn-events: _ -> [_ _ _ _ _ _ _ _ _ _ _ _ _ _ _ _ _ _ _ _ _ _ _]
      timeout: 1 -> [_ _ _ _ _ _ _ _ _ _ _ _ _ _ _ _ _ _ _ _ _ _ _]
      tunnel: [w326 _ _ w378 _ _ _ w540 _ _ _ w1701 w1741 w1779 _ _ _ _ _ _ _ w1907 _] -> w277
      tunnel: w276 -> [w326 _ _ w379 _ _ _ w539 _ _ _ w1737 w1776 w1815 _ _ _ _ _ _ _ w1912 _]
      tunnel: w275 -> [w325 _ _ w380 _ _ _ w538 _ _ _ w1736 w1775 w1814 _ _ _ _ _ _ _ w1911 _]
      tunnel: [w325 _ _ w377 _ _ _ w534 _ _ _ w1702 w1740 w1778 _ _ _ _ _ _ _ w1906 _] -> w274
      tunnel: w273 -> [w324 _ w368 _ _ _ _ w537 _ _ _ _ _ _ _ _ _ _ _ _ _ _ _]
      tunnel: w272 -> [w284 _ _ _ _ _ _ w536 _ _ _ _ _ _ _ _ _ _ _ _ _ _ _]
      tunnel: [w323 _ _ _ _ _ _ _ _ _ _ _ _ _ _ _ _ _ _ _ _ _ _] -> _
      tunnel: [w285 _ w362 _ _ _ _ w525 _ _ _ _ _ _ _ _ _ _ _ _ _ _ _] -> w271
      tunnel: w269 -> [w286 _ w367 _ _ _ _ w527 _ _ _ _ _ _ _ _ _ _ _ _ _ _ _]
      tunnel: [w286 _ w363 _ _ _ _ w526 _ _ _ _ _ _ _ _ _ _ _ _ _ _ _] -> w268
      tunnel: [w314 _ _ _ _ _ _ _ _ _ _ _ _ _ _ _ _ _ _ _ _ _ _] -> _
      tunnel: [w306 _ _ _ _ _ _ _ _ _ _ _ _ _ _ _ _ _ _ _ _ _ _] -> _
      tunnel: w267 -> [w305 w354 _ w376 _ _ _ w535 _ _ _ _ _ _ _ _ _ _ _ _ _ w1910 _]
      tunnel: w266 -> [w303 w353 _ w375 _ _ _ w517 _ _ _ _ _ _ _ _ _ _ _ _ _ w1904 _]
      tunnel: [w304 w352 _ w374 _ _ _ w533 _ _ _ _ _ _ _ _ _ _ _ _ _ w1908 _] -> w264
      tunnel: [w303 w353 _ _ _ _ _ w516 _ _ _ _ _ _ _ _ _ _ _ _ _ w1909 _] -> w265
      tunnel: w263 -> [_ _ _ _ _ _ _ w515 _ _ _ _ _ _ _ _ _ _ _ _ _ _ _]
      tunnel: w262 -> [w283 _ _ _ _ _ _ w510 _ _ _ _ _ _ _ _ _ _ _ _ _ _ _]
      event Timeout {
        n105 = event-data() -> ()  [unwired: 1 in, 3 out]
        n106 = property class="IPFS" props=["Position", "Resolution", "Type", "IsEnabled", "IsHandleEnable", "UpperLimit", "Status"](reference=w283) -> ("Type"=w281:i32, "Status"=w282:variant)  [unwired: 1 in, 7 out]
        n107 = Variant To Data(type=w281, Variant=w282) -> (data=w280:i32)  [unwired: 1 in, 1 out]
        n108 = local write "PFS status"(w280) -> ()
        n109 = local read "LASER shutter"() -> (w290:bool)
        n110 = local read "storeXY Position"() -> (w292:bool)
        n111 = case shown="Faux" w290 {
          tunnel: [0.0 5.0] -> w291
          frame False {
          }
          frame True {
          }
        }
        n112 = call "svi_mySerialWhereXY.vi"("entrée d'erreur (pas d'erreur)"=w305, "Refnum VISA en entrée"=w303) -> ("sortie d'erreur"=w304:errorcluster, "Y"=w300:dbl, "X"=w298:dbl)  [unwired: 7 in]
        n113 = call-poly <vilib>:"DAQmx Create Virtual Channel.vi"("maximum value"=5.0, "minimum value"=0.0, "physical channels"="Dev1/ao0", "units"=10348) -> ("task out"=w312:refnum<k21>, "error out"=w311:errorcluster)  [unwired: 10 in]
        n114 = Divide(x=w298, y=10.0) -> (x/y=w297:dbl)
        n115 = Divide(x=w300, y=10.0) -> (x/y=w299:dbl)
        n116 = property class="IZDrive"(reference=w284, error in=w324) -> (reference out=w323:refnum<k7>, error out=w322:errorcluster, "Position"=w321:variant, "Type"=w319:i32, "Resolution"=w320:variant)
        n117 = local write "Y position (µm)"(w299) -> ()
        n118 = local write "X position (µm)"(w297) -> ()
        n119 = stacked-sequence {
          frame #0 {
            n120 = call-poly <vilib>:"DAQmx Create Virtual Channel.vi"("physical channels"="Dev1/ai1") -> ("task out"=w328:refnum<k21>, "error out"=w335:errorcluster)  [unwired: 13 in]
            n121 = call-poly <vilib>:"DAQmx Read.vi"("task/channels in"=w328, "error in"=w335) -> ("task out"=w329:refnum<k21>, "data"=w331:dbl, "error out"=w334:errorcluster)  [unwired: 11 in]
            n122 = call <vilib>:"DAQmx Stop Task.vi"("task/channels in"=w329, "error in"=w334) -> ("task out"=w330:refnum<k21>, "error out"=w333:errorcluster)  [unwired: 12 in]
            n123 = local write "FlowRate (mL/min)"(w331) -> ()
            n124 = call <vilib>:"DAQmx Clear Task.vi"("task in"=w330, "error in"=w333) -> ()  [unwired: 13 in, 1 out]
          }
          frame #1 {
            n125 = call-poly <vilib>:"DAQmx Create Virtual Channel.vi"("physical channels"="Dev1/ai0") -> ("task out"=w337:refnum<k21>, "error out"=w338:errorcluster)  [unwired: 13 in]
            n126 = call-poly <vilib>:"DAQmx Read.vi"("task/channels in"=w337, "error in"=w338) -> ("task out"=w340:refnum<k21>, "data"=w336:dbl, "error out"=w339:errorcluster)  [unwired: 11 in]
            n127 = call <vilib>:"DAQmx Stop Task.vi"("task/channels in"=w340, "error in"=w339) -> ("task out"=w342:refnum<k21>, "error out"=w341:errorcluster)  [unwired: 12 in]
            n128 = call <vilib>:"DAQmx Clear Task.vi"("task in"=w342, "error in"=w341) -> ()  [unwired: 13 in, 1 out]
            n129 = local write "Laser Power (a.u.)"(w336) -> ()
          }
        }
        n130 = Variant To Data(error in=w322, type=w319, Variant=w321) -> (data=w317:i32, error out=w316:errorcluster)
        n131 = Variant To Data(error in=w316, type=w319, Variant=w320) -> (data=w318:i32, error out=w285:errorcluster)
        n132 = case shown="Faux" w292 {
          frame False {
          }
          frame True {
            n133 = stacked-sequence {
              frame #0 {
                n134 = local write "storeXY Position"(FALSE) -> ()
              }
              frame #1 {
                # "ajouter par ligne"
                # "ajouter par col"
                n135 = local read "X position (µm)"() -> (w351:dbl)
                n136 = local read "Y position (µm)"() -> (w350:dbl)
                n137 = local read "stored XY"() -> (w349:T1)
                n138 = Build Array(w351, w350) -> (w348:T1)
                n139 = Build Array (concatenate)(w349, w348) -> (w347:T1)
                n140 = local write "stored XY"(w347) -> ()
              }
            }
          }
        }
        n141 = Multiply(x=w317, y=w318) -> (x*y=w295:i32)
        n142 = To Double Precision Float(number=w295) -> (double precision float=w294:dbl)
        n143 = call-poly <vilib>:"DAQmx Write.vi"("task/channels in"=w312, "data"=w291, "error in"=w311) -> ("task out"=w309:refnum<k21>, "error out"=w310:errorcluster)  [unwired: 10 in, 1 out]
        n144 = Divide(x=w294, y=1000.0) -> (x/y=w296:dbl)
        n145 = local write "Z position"(w296) -> ()
        n146 = call <vilib>:"DAQmx Stop Task.vi"("task/channels in"=w309, "error in"=w310) -> ("task out"=w307:refnum<k21>, "error out"=w308:errorcluster)  [unwired: 12 in]
        n147 = call <vilib>:"DAQmx Clear Task.vi"("task in"=w307, "error in"=w308) -> ("error out"=w306:errorcluster)  [unwired: 13 in]
        n148 = Wait (ms)(milliseconds to wait=u32 500) -> (millisecond timer value=w314:u32)
        "Ready" <- TRUE
      }
      event "stage speed (mm/s)": Value Change {
        n149 = event-data() -> ("NewVal"=w355:sgl)  [unwired: 1 in, 4 out]
        n150 = stacked-sequence {
          tunnel: w355 -> [w359 _]
          tunnel: w354 -> [w358 _]
          tunnel: w353 -> [w357 _]
          tunnel: [w356 _] -> w352
          tunnel: [_ w360] -> _
          frame #0 {
            n151 = call "svi_mysetSpeedXY.vi"("entrée d'erreur (pas d'erreur)"=w358, "speed (mm/s)"=w359, "Refnum VISA en entrée"=w357) -> ("sortie d'erreur"=w356:errorcluster)  [unwired: 8 in]
          }
          frame #1 {
            n152 = Wait (ms)(milliseconds to wait=1000) -> (millisecond timer value=w360:u32)
          }
        }
      }
      event "Lower Filter": Value Change {
        n153 = event-data() -> ("NewVal"=w369:u8)  [unwired: 1 in, 4 out]
        n154 = To Variant(anything=w369) -> (Variant=w366:variant)
        n155 = property class="IFilterBlockCassette"(reference=w367, error in=w368, "Position"=w366) -> (reference out=w365:refnum<k7>, error out=w364:errorcluster)
        n156 = stacked-sequence {
          tunnel: w365 -> [_ w373]
          tunnel: w364 -> [_ w372]
          tunnel: [w370 _] -> _
          tunnel: [_ w373] -> w363
          tunnel: [_ w372] -> w362
          frame #0 {
            n157 = Wait (ms)(milliseconds to wait=u32 1000) -> (millisecond timer value=w370:u32)
          }
          frame #1 {
          }
        }
      }
      event "Free Run": Value Change {
        n158 = event-data() -> ("NewVal"=w381:bool)  [unwired: 1 in, 4 out]
        n159 = case shown="Vrai" w381 {
          tunnel: w380 -> [w384 w401]
          tunnel: [w384 w405] -> w377
          tunnel: w379 -> [w383 w402]
          tunnel: [w383 w400] -> w378
          tunnel: w376 -> [w382 w395]
          tunnel: w375 -> [_ w394]
          tunnel: [w382 w393] -> w374
          frame False {
          }
          frame True {
            # "*** Stop E/S device ***"
            # "*** Start E/S device ***"
            n160 = stacked-sequence {
              tunnel: w401 -> [w410]
              tunnel: [w413] -> w404
              tunnel: [w412] -> w403
              tunnel: w402 -> [w411]
              frame #0 {
                w415 = 7 items=["BINNING"=1, "BITS PER CHANNEL"=2, "ACTIVE VIEW INDEX"=3, "CCD MODE"=4, "SENSOR MODE"=5, "READOUT MODE"=6, "EXPOSURE TIME"=7, "CONTRAST GAIN"=8, "CONTRAST OFFSET"=9, "LIGHT MODE"=10, "SENSITIVITY"=11, "WHITE BALANCE"=12, "PHOTON IMAGING MODE"=13, "HIGH DYNAMIC RANGE MODE"=14, "TRIGGER SOURCE"=15, "TRIGGER ACTIVE"=16, "TRIGGER MODE"=17, "TRIGGER POLARITY"=18, "TRIGGER GLOBAL EXPOSURE"=19, "FIRST TRIGGER BEHAVIOR"=20, "TRIGGER TIMES"=21, "OUTPUT TRIGGER POLARITY"=22, "OUTPUT TRIGGER DELAY"=23, "OUTPUT TRIGGER PERIOD"=24, "TEMPERATURE"=25, "TEMPERATURE TARGET"=26, "SENSOR COOLER FAN"=27, "MECHANICAL SHUTTER"=28, "BACK FOCUS POSITION"=29, "FRAMEBUNDLE MODE"=30, "FRAMEBUNDLE NUMBER"=31] ("Parameter")
                n161 = local read "Exposure Time"() -> (w414:dbl)
                n162 = call <userlib>:"tm_setparameter.vi"("error in (no error)"=w410, "Value in"=w414, "Parameter"=w415, "Handle in"=w411) -> ("error out"=w412:errorcluster, "Handle out"=w413:u32)  [unwired: 6 in]
              }
            }
            n163 = call-poly <vilib>:"DAQmx Create Virtual Channel.vi"("maximum value"=5.0, "minimum value"=0.0, "physical channels"="Dev1/Ao0", "units"=10348) -> ("task out"=w391:refnum<k21>, "error out"=w390:errorcluster)  [unwired: 10 in]
            n164 = while {
              shift-right: [w424] -> w400
              shift-left: w404 -> [w426]
              shift-right: [w423] -> w405
              shift-left: w403 -> [w425]
              shift-right: [w427] -> w397
              shift-left: w390 -> [w416]
              shift-right: [w428] -> w396
              shift-left: w391 -> [w417]
              tunnel: w395 -> [w421]
              tunnel: w394 -> [w419]
              tunnel: [w418] -> w393
              stop <- w422 continue-if-true
              n165 = local read "storeXY Position"() -> (w420:bool)
              n166 = stacked-sequence {
                tunnel: w417 -> [w434 _ _ _]
                tunnel: w416 -> [w433 _ _ _]
                tunnel: [w430 _ _ _] -> w428
                tunnel: [w429 _ _ _] -> w427
                tunnel: w426 -> [_ w440 _ _]
                tunnel: w425 -> [_ w439 _ _]
                tunnel: [_ w442 _ _] -> w424
                tunnel: [_ w441 _ _] -> w423
                tunnel: [_ _ _ w466] -> _
                tunnel: w421 -> [_ _ w449 _]
                tunnel: w420 -> [_ _ w450 _]
                tunnel: w419 -> [_ _ w448 _]
                tunnel: [_ _ w447 _] -> w418
                frame #0 {
                  n167 = local read "LASER shutter"() -> (w432:bool)
                  n168 = case shown="Faux" w432 {
                    tunnel: [0.0 5.0] -> w431
                    frame False {
                    }
                    frame True {
                    }
                  }
                  n169 = call-poly <vilib>:"DAQmx Write.vi"("task/channels in"=w434, "data"=w431, "error in"=w433) -> ("task out"=w430:refnum<k21>, "error out"=w429:errorcluster)  [unwired: 10 in, 1 out]
                }
                frame #1 {
                  n170 = call <userlib>:"tm_firetrigger.vi"("error in (no error)"=w439, "Handle in"=w440) -> ("error out"=w446:errorcluster, "Handle out"=w445:u32)  [unwired: 8 in]
                  n171 = local read "Buffer Info"() -> (w438:T2)
                  n172 = call <userlib>:"tm_waitnextframe.vi"("error in (no error)"=w446, "Handle in"=w445) -> ("error out"=w443:errorcluster, "Handle out"=w444:u32)  [unwired: 6 in, 2 out]
                  n173 = call <userlib>:"tm_getframe_a.vi"("error in (no error)"=w443, "Buffer Info"=w438, "Handle in"=w444) -> ("error out"=w441:errorcluster, "Data 16"=w437:u16[][], "Handle out"=w442:u32)  [unwired: 4 in, 2 out]
                  n174 = local write "Imtemp"(w437) -> ()
                  n175 = local write "Intensity Graph"(w437) -> ()
                }
                frame #2 {
                  n176 = stacked-sequence {
                    tunnel: w450 -> [_ w459]
                    tunnel: w449 -> [w458 _]
                    tunnel: w448 -> [w457 _]
                    tunnel: [w451 _] -> w447
                    frame #0 {
                      w456 = 10.0
                      n177 = call "svi_mySerialWhereXY.vi"("entrée d'erreur (pas d'erreur)"=w458, "Refnum VISA en entrée"=w457) -> ("sortie d'erreur"=w451:errorcluster, "Y"=w455:dbl, "X"=w454:dbl)  [unwired: 7 in]
                      n178 = Divide(x=w454, y=w456) -> (x/y=w453:dbl)
                      n179 = Divide(x=w455, y=w456) -> (x/y=w452:dbl)
                      n180 = local write "X position (µm)"(w453) -> ()
                      n181 = local write "Y position (µm)"(w452) -> ()
                    }
                    frame #1 {
                      n182 = case shown="Vrai" w459 {
                        frame False {
                        }
                        frame True {
                          n183 = stacked-sequence {
                            frame #0 {
                              n184 = local write "storeXY Position"(FALSE) -> ()
                            }
                            frame #1 {
                              # "ajouter par ligne"
                              # "ajouter par col"
                              n185 = local read "X position (µm)"() -> (w465:dbl)
                              n186 = local read "Y position (µm)"() -> (w464:dbl)
                              n187 = local read "stored XY"() -> (w463:T1)
                              n188 = Build Array(w465, w464) -> (w462:T1)
                              n189 = Build Array (concatenate)(w463, w462) -> (w461:T1)
                              n190 = local write "stored XY"(w461) -> ()
                            }
                          }
                        }
                      }
                    }
                  }
                }
                frame #3 {
                  n191 = local read "Time between Images (Free Run)"() -> (w467:u32)
                  n192 = Wait (ms)(milliseconds to wait=w467) -> (millisecond timer value=w466:u32)
                }
              }
              n193 = local read "Free Run"() -> (w422:bool)
            }
            n194 = local read "LASER shutter"() -> (w386:bool)
            n195 = case shown="Faux" w386 {
              tunnel: [0.0 5.0] -> w385
              frame False {
              }
              frame True {
              }
            }
            n196 = call-poly <vilib>:"DAQmx Write.vi"("task/channels in"=w396, "data"=w385, "error in"=w397) -> ("task out"=w399:refnum<k21>, "error out"=w398:errorcluster)  [unwired: 10 in, 1 out]
            n197 = call <vilib>:"DAQmx Stop Task.vi"("task/channels in"=w399, "error in"=w398) -> ("task out"=w406:refnum<k21>, "error out"=w407:errorcluster)  [unwired: 12 in]
            n198 = call <vilib>:"DAQmx Clear Task.vi"("task in"=w406, "error in"=w407) -> ()  [unwired: 13 in, 1 out]
          }
        }
      }
      event "re-SET ALL\nPositions": Value Change {
        n199 = event-data() -> ("NewVal"=w468:bool)  [unwired: 1 in, 4 out]
        n200 = case shown="Vrai" w468 {
          frame False {
          }
          frame True {
            n201 = stacked-sequence {
              frame #0 {
                n202 = local read "Microscope Objective\nMagnification"() -> (w473:dbl)
                n203 = Build Array(0.0, 0.0) -> (w477:T1)
                n204 = Multiply(x=2048.0, y=6.5) -> (x*y=w470:dbl)
                n205 = Divide(x=w470, y=w473) -> (x/y=w469:dbl)
                n206 = call "vizuXY_svi.vi"("LY (mm)"=w469, "LX (mm)"=w469, "stored XY (µm)"=w477) -> ("Tableau"=w476:T4)  [unwired: 8 in]
                n207 = call "maximini_XYlist_svi.vi"("stored XY"=w477, "LY"=w469, "LX"=w469) -> ("mini (µm)"=w475:dbl, "maxi (µm)"=w474:dbl)  [unwired: 7 in]
                n208 = local write "stored XY"(w477) -> ()
                n209 = local write "Scanning Motif"(w476) -> ()
                n210 = property on="Scanning Motif" class="GraphXY (strict)"("XScale.Maximum"=w474, "XScale.Minimum"=w475, "YScale.Maximum"=w474, "YScale.Minimum"=w475) -> ()  [unwired: 2 in, 2 out]
              }
              frame #1 {
                n211 = local write "re-SET ALL\nPositions"(FALSE) -> ()
              }
            }
          }
        }
      }
      event "savelast": Value Change {
        n212 = event-data() -> ("NewVal"=w481:bool)  [unwired: 1 in, 4 out]
        n213 = case shown="Vrai" w481 {
          frame False {
          }
          frame True {
            n214 = stacked-sequence {
              frame #0 {
                w491 = T10 7 items=["Grayscale (U8)", "Grayscale (I16)", "Grayscale (SGL)", "Complex (CSG)", "RGB (U32)", "HSL (U32)", "RGB (U64)", "Grayscale (U16)"] ("Image Type")
                n215 = local read "Next Image Name"() -> (w485:string)
                n216 = local read "Current Directory"() -> (w488:path)
                n217 = local read "Imtemp"() -> (w489:u16[][])
                n218 = call "IMAQ Create"("Image Name"="nextimage", "Image Type"=w491) -> ("New Image"=w496:T11, "error out"=w492:errorcluster)  [unwired: 2 in, 1 out]
                n219 = Path To String(path=w488) -> (string=w487:string)
                n220 = call "IMAQ ArrayToImage"("Image Pixels (U16)"=w489, "error in (no error)"=w492, "Image"=w496) -> ("error out"=w493:errorcluster, "Image Out"=w494:T11)  [unwired: 7 in]
                n221 = Concatenate Strings(w487, "/", w485) -> (w484:string)
                n222 = String To Path(string=w484) -> (path=w483:path)
                n223 = call-poly "IMAQ Write File 2"("error in (no error)"=w493, "File Path"=w483, "Image"=w494) -> ("error out"=w490:errorcluster, "Image Out (duplicate)"=w495:T11)  [unwired: 2 in, 5 out]
                n224 = call "IMAQ Dispose"("Image"=w495, "error in (no error)"=w490) -> ()  [unwired: 1 in, 4 out]
              }
              frame #1 {
                n225 = local read "SavedImages"() -> (w501:i32)
                n226 = local read "file name motif"() -> (w497:string)
                n227 = Increment(x=w501) -> (x+1=w500:i32)
                n228 = Format Value(format string="%06d", value (0)=w500) -> (output string=w498:string)  [unwired: 1 in]
                n229 = local write "SavedImages"(w500) -> ()
                n230 = Concatenate Strings(w497, w498, ".tif") -> (w503:string)
                n231 = local write "Next Image Name"(w503) -> ()
              }
            }
          }
        }
      }
      event "file name motif": Value Change {
        w506 = 1
        n232 = event-data() -> ("NewVal"=w504:string)  [unwired: 1 in, 4 out]
        n233 = local write "SavedImages"(w506) -> ()
        n234 = Format Value(format string="%06d", value (0)=w506) -> (output string=w507:string)  [unwired: 1 in]
        n235 = Concatenate Strings(w504, w507, ".tif") -> (w505:string)
        n236 = local write "Next Image Name"(w505) -> ()
      }
      event "startTL": Value Change {
        n237 = event-data() -> ("NewVal"=w528:bool)  [unwired: 1 in, 4 out]
        n238 = local read "Min. Scan duration"() -> (w514:dbl)
        n239 = local read "used Filters"() -> (w520:u8[])
        n240 = local read "stored XY"() -> (w532:T1)
        n241 = Array Size(array=w520) -> (size(s)=w518:i32)
        n242 = Matrix Size(0:w532) -> (1:w529:i32)  [unwired: 1 out]
        n243 = To Unsigned Long Integer(number=w529) -> (unsigned 32bit integer=w531:u32)
        n244 = Multiply(x=w514, y=1000.0) -> (x*y=w512:dbl)
        n245 = To Unsigned Byte Integer(number=w518) -> (unsigned 8bit integer=w519:u8)
        n246 = Greater?(x=w529, y=0) -> (0:w524:bool)
        n247 = case shown="Faux" w524 {
          frame False {
            n248 = One Button Dialog(message="Select positions.... ;-)") -> ()  [unwired: 1 in, 1 out]
          }
          frame True {
          }
        }
        n249 = Greater Than 0?(x=w518) -> (x > 0?=w522:bool)
        n250 = case shown="Faux" w522 {
          frame False {
            n251 = One Button Dialog(message="Select Filters .... ;-)") -> ()  [unwired: 1 in, 1 out]
          }
          frame True {
          }
        }
        n252 = To Quad Integer(1:w512) -> (0:w511:i64)
        n253 = local write "TL_NCAN"(w519) -> ()
        n254 = And(x=w528, y=w524) -> (x .and. y?=w521:bool)
        n255 = local write "TL_NPOS"(w531) -> ()
        n256 = And(x=w521, y=w522) -> (x .and. y?=w523:bool)
        n257 = case shown="Vrai" w523 {
          tunnel: [w548 w556] -> w540
          tunnel: [w547 w555] -> w534
          tunnel: w539 -> [w548 w558]
          tunnel: w538 -> [w547 w557]
          tunnel: w537 -> [w545 w562]
          tunnel: w536 -> [_ w561]
          tunnel: [w545 w554] -> w525
          tunnel: w535 -> [w546 w564]
          tunnel: [w546 w563] -> w533
          tunnel: w527 -> [w544 w560]
          tunnel: [w544 w559] -> w526
          tunnel: w517 -> [w543 w553]
          tunnel: [w543 w552] -> w516
          tunnel: w515 -> [_ w551]
          tunnel: w511 -> [_ w550]
          tunnel: w510 -> [_ w549]
          frame False {
          }
          frame True {
            # "AI lfluidix\nFin"
            # "Sortie fluidix Fin"
            # "Sortie Fluidix Init"
            # "AI fluidix\nInit"
            # "Sortie Shutter Fin"
            # "Sortie Shutter Init"
            # "sortie numerique Fin\nLED 0-11"
            # "AI laser poser\nFin"
            # "Sortie Numérique Init\nLED 0-11"
            # "AI laser power\nInit"
            n258 = stacked-sequence {
              seq-local: [w595 _ _ _] -> [_ _ w804 _]
              seq-local: [w594 _ _ _] -> [_ _ w805 _]
              seq-local: [w581 _ _ _] -> [_ _ w811 _]
              seq-local: [w580 _ _ _] -> [_ _ w810 _]
              seq-local: [_ _ w803 _] -> [_ _ _ w1611]
              seq-local: [_ _ w802 _] -> [_ _ _ w1610]
              seq-local: [_ _ w799 _] -> [_ _ _ w1607]
              seq-local: [_ _ w798 _] -> [_ _ _ w1606]
              seq-local: [_ _ w797 _] -> [_ _ _ w1619]
              seq-local: [w579 _ _ _] -> [_ _ w794 _]
              seq-local: [w578 _ _ _] -> [_ _ w793 _]
              seq-local: [_ _ w792 _] -> [_ _ _ w1616]
              seq-local: [_ _ w791 _] -> [_ _ _ w1615]
              seq-local: [w569 _ _ _] -> [_ _ w789 _]
              seq-local: [w570 _ _ _] -> [_ _ w788 _]
              seq-local: [w571 _ _ _] -> [_ _ _ _]
              seq-local: [w572 _ _ _] -> [_ _ _ _]
              seq-local: [_ _ w787 _] -> [_ _ _ w1612]
              seq-local: [_ _ w786 _] -> [_ _ _ w1613]
              seq-local: [_ _ w785 _] -> [_ _ _ w1609]
              seq-local: [_ _ w784 _] -> [_ _ _ w1608]
              tunnel: w564 -> [w575 _ w812 _]
              tunnel: [_ _ _ w1618] -> w563
              tunnel: w562 -> [_ _ w795 _]
              tunnel: w561 -> [w568 _ w796 _]
              tunnel: w560 -> [_ _ w809 _]
              tunnel: [_ _ w808 _] -> w559
              tunnel: w558 -> [_ _ w807 _]
              tunnel: w557 -> [_ _ w806 _]
              tunnel: [_ _ w801 _] -> w556
              tunnel: [_ _ w800 _] -> w555
              tunnel: [_ _ w790 _] -> w554
              tunnel: w553 -> [w576 _ _ _]
              tunnel: [w573 _ _ _] -> w552
              tunnel: w551 -> [_ _ w781 _]
              tunnel: w550 -> [_ _ w780 _]
              tunnel: w549 -> [_ _ w779 _]
              frame #0 {
                n259 = stacked-sequence {
                  tunnel: [w611 _] -> w595
                  tunnel: [w610 _] -> w594
                  tunnel: [_ w614] -> w570
                  tunnel: [_ w613] -> w569
                  frame #0 {
                    n260 = call-poly <vilib>:"DAQmx Create Virtual Channel.vi"("physical channels"="Dev1/ai0") -> ("task out"=w611:refnum<k21>, "error out"=w610:errorcluster)  [unwired: 13 in]
                  }
                  frame #1 {
                    n261 = call-poly <vilib>:"DAQmx Create Virtual Channel.vi"("physical channels"="Dev1/ai1") -> ("task out"=w613:refnum<k21>, "error out"=w614:errorcluster)  [unwired: 13 in]
                  }
                }
                n262 = stacked-sequence {
                  tunnel: [w620 _] -> w579
                  tunnel: [w619 _] -> w578
                  tunnel: [_ w626] -> w572
                  tunnel: [_ w625] -> w571
                  frame #0 {
                    n263 = call-poly <vilib>:"DAQmx Create Virtual Channel.vi"("maximum value"=5.0, "minimum value"=0.0, "physical channels"="Dev1/Ao0", "units"=10348) -> ("task out"=w623:refnum<k21>, "error out"=w622:errorcluster)  [unwired: 10 in]
                    n264 = call-poly <vilib>:"DAQmx Write.vi"("task/channels in"=w623, "data"=0.0, "error in"=w622) -> ("task out"=w620:refnum<k21>, "error out"=w619:errorcluster)  [unwired: 10 in, 1 out]
                  }
                  frame #1 {
                    n265 = call-poly <vilib>:"DAQmx Create Virtual Channel.vi"("maximum value"=5.0, "minimum value"=0.0, "physical channels"="Dev1/Ao1", "units"=10348) -> ("task out"=w628:refnum<k21>, "error out"=w629:errorcluster)  [unwired: 10 in]
                    n266 = call-poly <vilib>:"DAQmx Write.vi"("task/channels in"=w628, "data"=0.0, "error in"=w629) -> ("task out"=w625:refnum<k21>, "error out"=w626:errorcluster)  [unwired: 10 in, 1 out]
                  }
                }
                n267 = local write "TLON"(TRUE) -> ()
                n268 = local write "Recorded Scans"(0) -> ()
                n269 = Build Array("Dev1/port0/line0:7", "Dev1/port1/line0:3") -> (w589:string[])
                n270 = property class="IZDrive"(reference=w568) -> ("Type"=w566:i32, "Position"=w567:variant)  [unwired: 1 in, 2 out]
                n271 = call <vilib>:"DAQmx Flatten Channel String.vi"("names in"=w589) -> ("names out"=w588:string, "error out"=w587:errorcluster)  [unwired: 13 in]
                n272 = call-poly <vilib>:"DAQmx Create Virtual Channel.vi"("lines"=w588, "line grouping"=1, "error in"=w587) -> ("task out"=w586:refnum<k21>, "error out"=w585:errorcluster)  [unwired: 11 in]
                n273 = Variant To Data(type=w566, Variant=w567) -> (data=w565:i32)  [unwired: 1 in, 1 out]
                n274 = Initialize Array(FALSE, 12) -> (w582:bool[])
                n275 = local write "lastgoodz"(w565) -> ()
                n276 = call-poly <vilib>:"DAQmx Write.vi"("task/channels in"=w586, "data"=w582, "error in"=w585) -> ("task out"=w581:refnum<k21>, "error out"=w580:errorcluster)  [unwired: 10 in, 1 out]
                n277 = stacked-sequence {
                  seq-local: [w596 _] -> [_ w609]
                  tunnel: w565 -> [_ w607]
                  frame #0 {
                    n278 = Initialize Array(nan, 0) -> (w601:dbl[])
                    n279 = local read "TL_NPOS"() -> (w599:u32)
                    n280 = call-poly <vilib>:"Array To Matrix.vi"("Real 1D Array"=w601) -> ("Real Matrix (Column Vector)"=w597:T1)
                    n281 = for {
                      N: w599 -> [_]
                      border: w597 -> [_]
                      tunnel: [w602] -> w596
                      n282 = Build Array(nan) -> (w604:T1)
                      n283 = feedback #1() -> (w603:T1)
                      n284 = Build Array (concatenate)(w603, w604) -> (w602:T1)
                      n285 = feedback-in #1(w602) -> ()
                    }
                  }
                  frame #1 {
                    w606 = 0
                    n286 = Replace Array Subset(array=w609, new element=w607, index (row)=w606, index (col)=w606) -> (w608:T1)
                    n287 = local write "lastgoodz_list"(w608) -> ()
                  }
                }
                n288 = local read "stage speed (mm/s)"() -> (w574:sgl)
                n289 = stacked-sequence {
                  tunnel: w576 -> [w634 _]
                  tunnel: w575 -> [w636 _]
                  tunnel: w574 -> [w635 _]
                  tunnel: [_ w638] -> _
                  tunnel: [w634 _] -> w573
                  frame #0 {
                    n290 = call "svi_mysetSpeedXY.vi"("entrée d'erreur (pas d'erreur)"=w636, "speed (mm/s)"=w635, "Refnum VISA en entrée"=w634) -> ()  [unwired: 8 in, 1 out]
                  }
                  frame #1 {
                    n291 = Wait (ms)(milliseconds to wait=1000) -> (millisecond timer value=w638:u32)
                  }
                }
              }
              frame #1 {
                n292 = local read "Camera Model"() -> (w647:string)
                n293 = local read "Camera Serial"() -> (w641:string)
                n294 = local read "Version"() -> (w644:string)
                n295 = local read "useLASER_TL"() -> (w652:bool)
                n296 = local read "useFLUIDICS_TL"() -> (w651:bool)
                n297 = local read "softversion"() -> (w674:string)
                n298 = local read "Current Directory"() -> (w675:path)
                n299 = local read "TL_NPOS"() -> (w650:u32)
                n300 = local read "TL_NCAN"() -> (w649:u8)
                n301 = local read "Total Number of Patterns"() -> (w662:u32)
                n302 = local read "Frames between Patterns"() -> (w663:u32)
                n303 = local read "Total Number of Scan"() -> (w660:u32)
                n304 = local read "Frames between Scan"() -> (w661:u32)
                n305 = local read "stage speed (mm/s)"() -> (w670:sgl)
                n306 = local read "Min. Scan duration"() -> (w656:dbl)
                n307 = local read "Stage COM PORT"() -> (w669:refnum<visa-resource-name>)
                n308 = local read "is_single_shoot"() -> (w655:bool)
                n309 = local read "Shoot at Scan#"() -> (w654:i32)
                n310 = local read "Shoot duration"() -> (w653:dbl)
                n311 = local read "used Filters"() -> (w667:u8[])
                n312 = local read "used LEDs"() -> (w668:bool[][])
                n313 = local read "Nstart FLUIDICS"() -> (w659:u32)
                n314 = local read "Exposure Time"() -> (w673:dbl)
                n315 = local read "Noff FLUIDICS"() -> (w657:u32)
                n316 = local read "Non FLUIDICS"() -> (w658:u32)
                n317 = local read "Nstart"() -> (w664:u32)
                n318 = local read "RO Mode"() -> (w671:u32)
                n319 = local read "Noff"() -> (w666:u32)
                n320 = local read "Non"() -> (w665:u32)
                n321 = Concatenate Strings("camera model :", w647, "\r", "camera version :", w644, "\r", "camera serial :", w641, "\r") -> (w639:string)
                n322 = local read "Binning"() -> (w672:u16)
                n323 = stacked-sequence {
                  tunnel: w650 -> [w678 w724 w735 w758]
                  tunnel: w649 -> [w677 w725 _ w757]
                  tunnel: w675 -> [w676 w721 w728 w756]
                  tunnel: w674 -> [_ w720 _ _]
                  tunnel: w673 -> [_ w718 _ _]
                  tunnel: w672 -> [_ w717 _ _]
                  tunnel: w671 -> [_ w716 _ _]
                  tunnel: w670 -> [_ w722 _ _]
                  tunnel: w669 -> [_ w723 _ _]
                  tunnel: w668 -> [_ w727 _ _]
                  tunnel: w667 -> [_ w726 _ _]
                  tunnel: w666 -> [_ w704 _ _]
                  tunnel: w665 -> [_ w705 _ _]
                  tunnel: w664 -> [_ w706 _ _]
                  tunnel: w663 -> [_ w707 _ _]
                  tunnel: w662 -> [_ w708 _ _]
                  tunnel: w661 -> [_ w714 _ _]
                  tunnel: w660 -> [_ w715 _ _]
                  tunnel: w659 -> [_ w702 _ _]
                  tunnel: w658 -> [_ w701 _ _]
                  tunnel: w657 -> [_ w700 _ _]
                  tunnel: w656 -> [_ w713 _ _]
                  tunnel: w655 -> [_ w711 _ _]
                  tunnel: w654 -> [_ w710 _ _]
                  tunnel: w653 -> [_ w709 _ _]
                  tunnel: w652 -> [_ w712 _ _]
                  tunnel: w651 -> [_ w703 _ _]
                  tunnel: w639 -> [_ w719 _ _]
                  frame #0 {
                    n324 = for {
                      N: w678 -> [_]
                      tunnel: w677 -> [w680]
                      tunnel: w676 -> [w679]
                      i -> [w685]
                      n325 = Path To String(path=w679) -> (string=w687:string)
                      n326 = Format Value(string ("")="\\Pos_", format string="%05d" ("chaîne"), value (0)=w685) -> (output string=w683:string)
                      n327 = Concatenate Strings(w687, w683, "\\") -> (w681:string)
                      n328 = stacked-sequence {
                        tunnel: w681 -> [w689 w691]
                        tunnel: w680 -> [_ w690]
                        frame #0 {
                          n329 = String To Path(string=w689) -> (path=w688:path)
                          n330 = Create Folder ("Créer un dossier")(path (use dialog)=w688) -> ()  [unwired: 2 in, 3 out]
                        }
                        frame #1 {
                          n331 = for {
                            N: w690 -> [_]
                            tunnel: w691 -> [w693]
                            i -> [w692]
                            n332 = Format Value(string ("")="\\chanel", format string="%d" ("chaîne"), value (0)=w692) -> (output string=w697:string)
                            n333 = Concatenate Strings(w693, w697, "\\") -> (w695:string)
                            n334 = String To Path(string=w695) -> (path=w694:path)
                            n335 = Create Folder ("Créer un dossier")(path (use dialog)=w694) -> ()  [unwired: 2 in, 3 out]
                          }
                        }
                      }
                    }
                  }
                  frame #1 {
                    n336 = call "save_infos_v4_svi.vi"("Refnum VISA en entrée"=w723, "STAGE_SPEED"=w722, "info Directory"=w721, "USED_FILTERS"=w726, "NUM_POS"=w724, "NB_CHANELS"=w725, "NSCAN"=w715, "Noff_fluidix"=w700, "Camera infos"=w719, "BETWEEN_SCAN"=w714, "ROMODE"=w716, "Non_fluidix"=w701, "BIN"=w717, "useLASER"=w712, "SOFT_VERSION"=w720, "Nstart_fluidics"=w702, "EXPT"=w718, "MIN SCAN DURATION"=w713, "USED_LEDS"=w727, "useFLUIDCS"=w703, "Noff_laser"=w704, "Non_laser"=w705, "Nstart_laser"=w706, "BETWEEN_PATTERN"=w707, "NPATTERN"=w708, "SHOOT_AT_SCAN"=w710, "SHOOT_DUR"=w709, "is_singleshoot"=w711) -> ()
                  }
                  frame #2 {
                    n337 = Path To String(path=w728) -> (string=w737:string)
                    n338 = Concatenate Strings(w737, "\\XY_positions.txt") -> (w736:string)
                    n339 = String To Path(string=w736) -> (path=w729:path)
                    n340 = Open/Create/Replace File(file path (use dialog)=w729, operation (0:open)=4) -> (refnum out=w733:refnum<file>, error out=w732:errorcluster)  [unwired: 4 in, 1 out]
                    n341 = for {
                      N: w735 -> [_]
                      tunnel: w733 -> [w743]
                      tunnel: w732 -> [w742]
                      tunnel: [w741] -> w731
                      tunnel: [w740] -> w730
                      i -> [w752]
                      n342 = local read "stored XY"() -> (w750:T1)
                      n343 = Index Array(array=w750, index (row)=w752, index (col)=0) -> (element=w754:dbl)
                      n344 = Format Value(format string="%f" ("chaîne"), value (0)=w754) -> (output string=w746:string)  [unwired: 1 in]
                      n345 = Index Array(array=w750, index (row)=w752, index (col)=1) -> (element=w748:dbl)
                      n346 = Format Value(string ("")=" ; ", format string="%f" ("chaîne"), value (0)=w748) -> (output string=w745:string)
                      n347 = Concatenate Strings(w746, w745, "\r") -> (w744:string)
                      n348 = Write to Text File(file (use dialog)=w743, text=w744, error in=w742) -> (refnum out=w741:refnum<file>, error out=w740:errorcluster)  [unwired: 1 in, 1 out]
                    }
                    n349 = Close File(refnum=w731, error in=w730) -> ()  [unwired: 2 out]
                  }
                  frame #3 {
                    n350 = for {
                      N: w758 -> [_]
                      tunnel: w757 -> [w760]
                      tunnel: w756 -> [w759]
                      i -> [w764]
                      n351 = Path To String(path=w759) -> (string=w763:string)
                      n352 = Format Value(string ("")="\\Pos_", format string="%05d" ("chaîne"), value (0)=w764) -> (output string=w762:string)
                      n353 = Concatenate Strings(w763, w762) -> (w761:string)
                      n354 = for {
                        N: w760 -> [_]
                        tunnel: w761 -> [w776]
                        i -> [w767]
                        n355 = Format Value(string ("")="\\ext_in_chanel", format string="%d" ("chaîne"), value (0)=w767) -> (output string=w775:string)
                        n356 = Concatenate Strings(w776, w775, ".txt") -> (w773:string)
                        n357 = String To Path(string=w773) -> (path=w772:path)
                        n358 = Open/Create/Replace File(file path (use dialog)=w772, prompt="", operation (0:open)=4) -> (refnum out=w768:refnum<file>, error out=w769:errorcluster)  [unwired: 3 in, 1 out]
                        n359 = Close File(refnum=w768, error in=w769) -> ()  [unwired: 2 out]
                      }
                    }
                  }
                }
              }
              frame #2 {
                n360 = node-c288(w781, w780) -> (w783:T7)  [unwired: 2 in]
                n361 = timed-loop {
                  tunnel: w812 -> [w845]
                  tunnel: w811 -> [w844]
                  tunnel: w810 -> [w843]
                  tunnel: w809 -> [w842]
                  tunnel: [w841] -> w808
                  tunnel: w807 -> [w840]
                  tunnel: w806 -> [w839]
                  tunnel: w805 -> [w838]
                  tunnel: w804 -> [w837]
                  tunnel: [w836] -> w803
                  tunnel: [w835] -> w802
                  tunnel: [w834] -> w801
                  tunnel: [w833] -> w800
                  tunnel: [w832] -> w799
                  tunnel: [w831] -> w798
                  tunnel: [w830] -> w797
                  tunnel: w796 -> [w827]
                  tunnel: w795 -> [w826]
                  tunnel: w794 -> [w825]
                  tunnel: w793 -> [w824]
                  tunnel: [w823] -> w792
                  tunnel: [w822] -> w791
                  tunnel: [w821] -> w790
                  tunnel: w789 -> [w820]
                  tunnel: w788 -> [w819]
                  tunnel: [w818] -> w787
                  tunnel: [w817] -> w786
                  tunnel: [w815] -> w785
                  tunnel: [w814] -> w784
                  timing: w783 -> [_]
                  timing-out: [_] -> w782
                  tunnel: w779 -> [w813]
                  i -> [w816]
                  stop <- w848 stop-if-true
                  n362 = node-c288() -> ()  [unwired: 1 in, 1 out]
                  n363 = stacked-sequence {
                    seq-local: [_ w901 _ _ _] -> [_ _ _ w1568 _]
                    seq-local: [_ w900 _ _ _] -> [_ _ _ w1567 _]
                    seq-local: [_ w899 _ _ _] -> [_ _ w1562 _ _]
                    tunnel: w845 -> [_ w912 _ _ _]
                    tunnel: w844 -> [_ w911 _ _ _]
                    tunnel: w843 -> [_ w910 _ _ _]
                    tunnel: w842 -> [_ w909 _ _ _]
                    tunnel: [_ w908 _ _ _] -> w841
                    tunnel: w840 -> [_ w907 _ _ _]
                    tunnel: w839 -> [_ w906 _ _ _]
                    tunnel: w838 -> [_ w905 _ _ _]
                    tunnel: w837 -> [_ w904 _ _ _]
                    tunnel: [_ w903 _ _ _] -> w836
                    tunnel: [_ w902 _ _ _] -> w835
                    tunnel: [_ _ _ w1566 _] -> w834
                    tunnel: [_ _ _ w1565 _] -> w833
                    tunnel: [_ w898 _ _ _] -> w832
                    tunnel: [_ w897 _ _ _] -> w831
                    tunnel: [_ _ w1550 _ _] -> w830
                    tunnel: w816 -> [_ _ _ _ w1599]
                    tunnel: w827 -> [_ w890 _ _ _]
                    tunnel: w826 -> [_ w889 _ _ _]
                    tunnel: w825 -> [_ w894 _ _ _]
                    tunnel: w824 -> [_ w893 _ _ _]
                    tunnel: [_ w892 _ _ _] -> w823
                    tunnel: [_ w891 _ _ _] -> w822
                    tunnel: [_ w888 _ _ _] -> w821
                    tunnel: w820 -> [w857 w887 _ _ _]
                    tunnel: w819 -> [w856 w886 _ _ _]
                    tunnel: [w855 _ _ _ _] -> w818
                    tunnel: [w854 _ _ _ _] -> w817
                    tunnel: w816 -> [w853 w883 _ _ _]
                    tunnel: [_ w885 _ _ _] -> w815
                    tunnel: [_ w884 _ _ _] -> w814
                    tunnel: w813 -> [_ w882 _ _ _]
                    frame #0 {
                      w858 = 0
                      n364 = local read "useFLUIDICS_TL"() -> (w852:bool)
                      n365 = local write "Recorded\nPatterns"(w858) -> ()
                      n366 = local write "Next Scan"(w858) -> ()
                      n367 = case shown="Vrai" w852 {
                        tunnel: w857 -> [w859 w865]
                        tunnel: w856 -> [w860 w864]
                        tunnel: [w859 w863] -> w855
                        tunnel: [w860 w862] -> w854
                        tunnel: w853 -> [_ w861]
                        frame False {
                        }
                        frame True {
                          # "motif index"
                          # "number of motif done"
                          n368 = local read "Noff FLUIDICS"() -> (w879:u32)
                          n369 = local read "Non FLUIDICS"() -> (w878:u32)
                          n370 = local read "Nstart FLUIDICS"() -> (w877:u32)
                          n371 = Add(x=w878, y=w879) -> (x+y=w876:u32)
                          n372 = Subtract(x=w861, y=w877) -> (x-y=w872:u32)
                          n373 = Greater Or Equal To 0?(x=w872) -> (x >= 0?=w870:bool)
                          n374 = Divide(x=w872, y=w876) -> (x/y=w875:dbl)
                          n375 = Round Toward -Infinity(1:w875) -> (0:w874:dbl)
                          n376 = Multiply(x=w874, y=w876) -> (x*y=w873:dbl)
                          n377 = Subtract(x=w872, y=w873) -> (x-y=w871:dbl)
                          n378 = Greater Or Equal?(x=w871, y=w878) -> (x >= y?=w869:bool)
                          n379 = Or(x=w869, y=w870) -> (x .or. y?=w868:bool)
                          n380 = Not(x=w868) -> (.not. x?=w867:bool)
                          n381 = case shown="Faux" w867 {
                            tunnel: [0.0 5.0] -> w866
                            frame False {
                            }
                            frame True {
                            }
                          }
                          n382 = local write "TL Fluidic SYNC"(w867) -> ()
                          n383 = call-poly <vilib>:"DAQmx Write.vi"("task/channels in"=w865, "data"=w866, "error in"=w864) -> ("task out"=w863:refnum<k21>, "error out"=w862:errorcluster)  [unwired: 10 in, 1 out]
                        }
                      }
                    }
                    frame #1 {
                      n384 = local read "TL_NPOS"() -> (w896:u32)
                      n385 = To Long Integer(number=w896) -> (32bit integer=w895:i32)
                      n386 = for {
                        N: w895 -> [_]
                        tunnel: w912 -> [w942]
                        tunnel: w911 -> [w940]
                        tunnel: w910 -> [w939]
                        tunnel: w909 -> [w938]
                        tunnel: [w937] -> w908
                        tunnel: w907 -> [w936]
                        tunnel: w906 -> [w935]
                        tunnel: w905 -> [w934]
                        tunnel: w904 -> [w933]
                        tunnel: [w932] -> w903
                        tunnel: [w931] -> w902
                        tunnel: [w930] -> w901
                        tunnel: [w929] -> w900
                        tunnel: [w928] -> w899
                        tunnel: [w927] -> w898
                        tunnel: [w926] -> w897
                        tunnel: w894 -> [w925]
                        tunnel: w893 -> [w924]
                        tunnel: [w923] -> w892
                        tunnel: [w922] -> w891
                        tunnel: w890 -> [w921]
                        tunnel: w889 -> [w920]
                        tunnel: [w919] -> w888
                        tunnel: w887 -> [w918]
                        tunnel: w886 -> [w917]
                        tunnel: [w916] -> w885
                        tunnel: [w915] -> w884
                        tunnel: w883 -> [w914]
                        tunnel: w882 -> [w913]
                        i -> [w941]
                        n387 = stacked-sequence {
                          seq-local: [_ _ _ w1238 _ _] -> [_ _ _ _ w1260 _]
                          seq-local: [_ _ _ w1237 _ _] -> [_ _ _ _ w1259 _]
                          seq-local: [_ _ _ _ w1257 _] -> [_ _ _ _ _ w1548]
                          seq-local: [_ _ _ _ w1258 _] -> [_ _ _ _ _ w1549]
                          seq-local: [_ _ _ w1233 _ _] -> [_ _ _ _ w1256 _]
                          seq-local: [_ _ _ w1232 _ _] -> [_ _ _ _ w1255 _]
                          seq-local: [_ _ _ _ w1253 _] -> [_ _ _ _ _ w1540]
                          seq-local: [_ _ _ _ w1254 _] -> [_ _ _ _ _ w1541]
                          tunnel: w942 -> [w958 _ _ _ _ _]
                          tunnel: w941 -> [w945 _ w962 _ w1244 _]
                          tunnel: [_ w960 _ _ _ _] -> _
                          tunnel: w940 -> [_ _ _ w1240 w1272 _]
                          tunnel: w939 -> [_ _ _ w1239 w1271 _]
                          tunnel: w938 -> [_ _ _ _ w1270 _]
                          tunnel: [_ _ _ _ w1269 _] -> w937
                          tunnel: w936 -> [_ _ _ _ w1268 _]
                          tunnel: w935 -> [_ _ _ _ w1267 _]
                          tunnel: w934 -> [_ _ _ _ w1266 _]
                          tunnel: w933 -> [_ _ _ _ w1265 _]
                          tunnel: [_ _ _ _ w1264 _] -> w932
                          tunnel: [_ _ _ _ w1263 _] -> w931
                          tunnel: [_ _ _ _ w1262 _] -> w930
                          tunnel: [_ _ _ _ w1261 _] -> w929
                          tunnel: [w946 _ _ _ _ _] -> w928
                          tunnel: [_ _ _ _ _ w1544] -> w927
                          tunnel: [_ _ _ _ _ w1543] -> w926
                          tunnel: w925 -> [_ _ _ w1235 _ _]
                          tunnel: w924 -> [_ _ _ w1234 _ _]
                          tunnel: [_ _ _ _ _ w1539] -> w923
                          tunnel: [_ _ _ _ _ w1538] -> w922
                          tunnel: w921 -> [_ _ w972 _ w1252 _]
                          tunnel: w920 -> [_ _ _ _ w1251 _]
                          tunnel: [_ _ _ _ w1250 _] -> w919
                          tunnel: w918 -> [_ _ _ _ w1249 _]
                          tunnel: w917 -> [_ _ _ _ w1248 _]
                          tunnel: [_ _ _ _ w1247 _] -> w916
                          tunnel: [_ _ _ _ w1246 _] -> w915
                          tunnel: w914 -> [_ _ _ _ w1245 _]
                          tunnel: w913 -> [_ _ w975 _ _ _]
                          frame #0 {
                            n388 = local read "stored XY"() -> (w952:T1)
                            n389 = Index Array(array=w952, index (row)=w945, index (col)=0) -> (element=w948:dbl)
                            n390 = Index Array(array=w952, index (row)=w945, index (col)=1) -> (element=w947:dbl)
                            n391 = Multiply(x=w948, y=10) -> (x*y=w955:dbl)
                            n392 = To Long Integer(number=w955) -> (32bit integer=w954:i32)
                            n393 = Multiply(x=w947, y=10) -> (x*y=w950:dbl)
                            n394 = To Long Integer(number=w950) -> (32bit integer=w949:i32)
                            n395 = local write "Next Pattern"(0) -> ()
                            n396 = call "SerialMoveXY.vi"("error in (no error)"=w958, "Y"=w949, "X"=w954) -> ("error out"=w946:errorcluster)  [unwired: 2 in]
                            n397 = To Unsigned Long Integer(number=w945) -> (unsigned 32bit integer=w944:u32)
                            n398 = local write "X position (µm)"(w948) -> ()
                            n399 = local write "Y position (µm)"(w947) -> ()
                            n400 = local write "Current Position"(w944) -> ()
                          }
                          frame #1 {
                            n401 = local read "Delay after Move"() -> (w959:u32)
                            n402 = Wait (ms)(milliseconds to wait=w959) -> (millisecond timer value=w960:u32)
                          }
                          frame #2 {
                            n403 = local read "lastgoodz_list"() -> (w963:T1)
                            n404 = local read "lastgoodz"() -> (w966:i32)
                            n405 = property class="IPFS"(reference=w975) -> (reference out=w971:refnum<k7>, "Type"=w974:i32, "Status"=w973:variant)  [unwired: 1 in, 1 out]
                            n406 = Index Array(array=w963, index (row)=w962, index (col)=0) -> (element=w967:dbl)
                            n407 = Variant To Data(type=w974, Variant=w973) -> (data=w970:i32, error out=w969:errorcluster)  [unwired: 1 in]
                            n408 = local write "PFS status"(w970) -> ()
                            n409 = case shown="5" w970 {
                              tunnel: w972 -> [w979 w1014 w1065 w1117 w1171 w1229]
                              tunnel: w971 -> [w981 w1016 w1067 w1119 w1170 _]
                              tunnel: [w980 w1015 w1066 w1118 w1173 w1227] -> _
                              tunnel: w969 -> [_ _ _ _ w1172 _]
                              tunnel: w967 -> [w978 w1013 w1063 w1116 w1169 _]
                              tunnel: w962 -> [_ _ _ w1115 _ _]
                              tunnel: w966 -> [w977 w1012 w1064 w1114 w1168 _]
                              tunnel: [w976 w1011 w1062 w1113 w1167 w1226] -> w961
                              frame 2 {
                                n410 = stacked-sequence {
                                tunnel: w981 -> [w985 _ w995]
                                tunnel: [w984 _ _] -> w980
                                tunnel: w979 -> [_ _ w994]
                                tunnel: [_ w986 _] -> _
                                tunnel: w978 -> [_ _ w990]
                                tunnel: w977 -> [_ _ w989]
                                tunnel: [_ _ w988] -> w976
                                frame #0 {
                                n411 = To Variant(anything=1) -> (Variant=w982:variant)
                                n412 = property class="IPFS"(reference=w985, "IsEnabled"=w982) -> (error out=w984:errorcluster)  [unwired: 1 in, 1 out]
                                }
                                frame #1 {
                                n413 = local read "Delay PFS"() -> (w987:u32)
                                n414 = Wait (ms)(milliseconds to wait=w987) -> (millisecond timer value=w986:u32)
                                }
                                frame #2 {
                                n415 = property class="IPFS"(reference=w995) -> ("Type"=w996:i32, "Status"=w997:variant)  [unwired: 1 in, 2 out]
                                n416 = Variant To Data(type=w996, Variant=w997) -> (data=w992:i32)  [unwired: 1 in, 1 out]
                                n417 = local write "PFS status"(w992) -> ()
                                n418 = Equal?(x=w992, y=5) -> (x = y?=w991:bool)
                                n419 = case shown="Vrai" w991 {
                                tunnel: w994 -> [w1004 w1010]
                                tunnel: w990 -> [w999 _]
                                tunnel: w989 -> [w1001 _]
                                tunnel: [nan w1007] -> w988
                                frame False {
                                n420 = Not A Number/Path/Refnum?(number/path/refnum=w999) -> (NaN/Path/Refnum?=w1002:bool)
                                n421 = case shown="Faux" w1002 {
                                tunnel: [w1005 w1006] -> w1000
                                tunnel: w1001 -> [_ w1006]
                                tunnel: w999 -> [w1005 _]
                                frame False {
                                }
                                frame True {
                                }
                                }
                                n422 = To Variant(anything=w1000) -> (Variant=w1003:variant)
                                n423 = property class="IZDrive"(reference=w1004, "Position"=w1003) -> ()  [unwired: 1 in, 2 out]
                                }
                                frame True {
                                n424 = property class="IZDrive"(reference=w1010) -> ("Type"=w1009:i32, "Position"=w1008:variant)  [unwired: 1 in, 2 out]
                                n425 = Variant To Data(type=w1009, Variant=w1008) -> (data=w1007:i32)  [unwired: 1 in, 1 out]
                                n426 = local write "lastgoodz"(w1007) -> ()
                                }
                                }
                                }
                                }
                              }
                              frame 6 {
                                n427 = stacked-sequence {
                                tunnel: w1016 -> [_ w1028 _ w1037]
                                tunnel: [_ w1027 _ _] -> w1015
                                tunnel: w1014 -> [w1022 _ _ w1036]
                                tunnel: [_ _ w1029 _] -> _
                                tunnel: w1013 -> [w1017 _ _ w1032]
                                tunnel: w1012 -> [w1018 _ _ w1031]
                                tunnel: [_ _ _ w1033] -> w1011
                                frame #0 {
                                n428 = Not A Number/Path/Refnum?(number/path/refnum=w1017) -> (NaN/Path/Refnum?=w1020:bool)
                                n429 = case shown="Faux" w1020 {
                                tunnel: [w1023 w1024] -> w1019
                                tunnel: w1018 -> [_ w1024]
                                tunnel: w1017 -> [w1023 _]
                                frame False {
                                }
                                frame True {
                                }
                                }
                                n430 = To Variant(anything=w1019) -> (Variant=w1021:variant)
                                n431 = property class="IZDrive"(reference=w1022, "Position"=w1021) -> ()  [unwired: 1 in, 2 out]
                                }
                                frame #1 {
                                n432 = To Variant(anything=1) -> (Variant=w1025:variant)
                                n433 = property class="IPFS"(reference=w1028, "IsEnabled"=w1025) -> (error out=w1027:errorcluster)  [unwired: 1 in, 1 out]
                                }
                                frame #2 {
                                n434 = local read "Delay PFS"() -> (w1030:u32)
                                n435 = Wait (ms)(milliseconds to wait=w1030) -> (millisecond timer value=w1029:u32)
                                }
                                frame #3 {
                                n436 = property class="IPFS"(reference=w1037) -> (reference out=w1035:refnum<k7>, "Type"=w1038:i32, "Status"=w1039:variant)  [unwired: 1 in, 1 out]
                                n437 = Variant To Data(type=w1038, Variant=w1039) -> (data=w1034:i32)  [unwired: 1 in, 1 out]
                                n438 = local write "PFS status"(w1034) -> ()
                                n439 = case shown="4" w1034 {
                                tunnel: w1036 -> [w1044 _ w1061]
                                tunnel: w1035 -> [w1043 _ _]
                                tunnel: [w1040 nan w1058] -> w1033
                                tunnel: w1032 -> [w1042 _ _]
                                tunnel: w1031 -> [w1041 _ _]
                                frame 0, 1, 6, Default {
                                n440 = stacked-sequence {
                                tunnel: w1044 -> [_ w1053]
                                tunnel: w1043 -> [w1047 _]
                                tunnel: w1042 -> [_ w1049]
                                tunnel: w1041 -> [_ w1051]
                                tunnel: [_ nan] -> w1040
                                frame #0 {
                                n441 = To Variant(anything=0) -> (Variant=w1046:variant)
                                n442 = property class="IPFS"(reference=w1047, "IsEnabled"=w1046) -> ()  [unwired: 1 in, 2 out]
                                }
                                frame #1 {
                                n443 = Not A Number/Path/Refnum?(number/path/refnum=w1049) -> (NaN/Path/Refnum?=w1052:bool)
                                n444 = case shown="Faux" w1052 {
                                tunnel: [w1055 w1056] -> w1050
                                tunnel: w1051 -> [_ w1056]
                                tunnel: w1049 -> [w1055 _]
                                frame False {
                                }
                                frame True {
                                }
                                }
                                n445 = To Variant(anything=w1050) -> (Variant=w1054:variant)
                                n446 = property class="IZDrive"(reference=w1053, "Position"=w1054) -> ()  [unwired: 1 in, 2 out]
                                }
                                }
                                }
                                frame 4 {
                                }
                                frame 5 {
                                n447 = property class="IZDrive"(reference=w1061) -> ("Type"=w1060:i32, "Position"=w1059:variant)  [unwired: 1 in, 2 out]
                                n448 = Variant To Data(type=w1060, Variant=w1059) -> (data=w1058:i32)  [unwired: 1 in, 1 out]
                                n449 = local write "lastgoodz"(w1058) -> ()
                                }
                                }
                                }
                                }
                              }
                              frame 1 {
                                n450 = stacked-sequence {
                                tunnel: w1067 -> [_ w1079 _ w1088]
                                tunnel: [_ w1078 _ _] -> w1066
                                tunnel: w1065 -> [w1073 _ _ w1087]
                                tunnel: [_ _ w1080 _] -> _
                                tunnel: w1064 -> [w1070 _ _ w1082]
                                tunnel: w1063 -> [w1068 _ _ w1083]
                                tunnel: [_ _ _ w1084] -> w1062
                                frame #0 {
                                n451 = Not A Number/Path/Refnum?(number/path/refnum=w1068) -> (NaN/Path/Refnum?=w1071:bool)
                                n452 = case shown="Faux" w1071 {
                                tunnel: w1070 -> [_ w1075]
                                tunnel: [w1074 w1075] -> w1069
                                tunnel: w1068 -> [w1074 _]
                                frame False {
                                }
                                frame True {
                                }
                                }
                                n453 = To Variant(anything=w1069) -> (Variant=w1072:variant)
                                n454 = property class="IZDrive"(reference=w1073, "Position"=w1072) -> ()  [unwired: 1 in, 2 out]
                                }
                                frame #1 {
                                n455 = To Variant(anything=1) -> (Variant=w1076:variant)
                                n456 = property class="IPFS"(reference=w1079, "IsEnabled"=w1076) -> (error out=w1078:errorcluster)  [unwired: 1 in, 1 out]
                                }
                                frame #2 {
                                n457 = local read "Delay PFS"() -> (w1081:u32)
                                n458 = Wait (ms)(milliseconds to wait=w1081) -> (millisecond timer value=w1080:u32)
                                }
                                frame #3 {
                                n459 = property class="IPFS"(reference=w1088) -> (reference out=w1086:refnum<k7>, "Type"=w1089:i32, "Status"=w1090:variant)  [unwired: 1 in, 1 out]
                                n460 = Variant To Data(type=w1089, Variant=w1090) -> (data=w1085:i32)  [unwired: 1 in, 1 out]
                                n461 = local write "PFS status"(w1085) -> ()
                                n462 = case shown="5" w1085 {
                                tunnel: w1087 -> [w1095 _ w1112]
                                tunnel: w1086 -> [w1094 _ _]
                                tunnel: [w1091 nan w1109] -> w1084
                                tunnel: w1083 -> [w1093 _ _]
                                tunnel: w1082 -> [w1092 _ _]
                                frame 0, 1, 6, Default {
                                n463 = stacked-sequence {
                                tunnel: w1095 -> [_ w1104]
                                tunnel: w1094 -> [w1098 _]
                                tunnel: w1093 -> [_ w1100]
                                tunnel: w1092 -> [_ w1101]
                                tunnel: [_ nan] -> w1091
                                frame #0 {
                                n464 = To Variant(anything=0) -> (Variant=w1097:variant)
                                n465 = property class="IPFS"(reference=w1098, "IsEnabled"=w1097) -> ()  [unwired: 1 in, 2 out]
                                }
                                frame #1 {
                                n466 = Not A Number/Path/Refnum?(number/path/refnum=w1100) -> (NaN/Path/Refnum?=w1103:bool)
                                n467 = case shown="Faux" w1103 {
                                tunnel: [w1106 w1107] -> w1102
                                tunnel: w1101 -> [_ w1107]
                                tunnel: w1100 -> [w1106 _]
                                frame False {
                                }
                                frame True {
                                }
                                }
                                n468 = To Variant(anything=w1102) -> (Variant=w1105:variant)
                                n469 = property class="IZDrive"(reference=w1104, "Position"=w1105) -> ()  [unwired: 1 in, 2 out]
                                }
                                }
                                }
                                frame 4 {
                                }
                                frame 5 {
                                n470 = property class="IZDrive"(reference=w1112) -> ("Type"=w1111:i32, "Position"=w1110:variant)  [unwired: 1 in, 2 out]
                                n471 = Variant To Data(type=w1111, Variant=w1110) -> (data=w1109:i32)  [unwired: 1 in, 1 out]
                                n472 = local write "lastgoodz"(w1109) -> ()
                                }
                                }
                                }
                                }
                              }
                              frame 0, Default {
                                n473 = stacked-sequence {
                                tunnel: w1119 -> [_ w1133 _ w1142]
                                tunnel: [_ w1132 _ _] -> w1118
                                tunnel: w1117 -> [w1122 _ _ w1141]
                                tunnel: [_ _ w1134 _] -> _
                                tunnel: w1116 -> [w1121 _ _ w1138]
                                tunnel: w1115 -> [_ _ _ _]
                                tunnel: w1114 -> [w1120 _ _ w1137]
                                tunnel: [_ _ _ w1136] -> w1113
                                frame #0 {
                                n474 = Not A Number/Path/Refnum?(number/path/refnum=w1121) -> (NaN/Path/Refnum?=w1123:bool)
                                n475 = case shown="Vrai" w1123 {
                                tunnel: w1122 -> [w1124 w1128]
                                tunnel: w1121 -> [w1125 _]
                                tunnel: w1120 -> [_ w1127]
                                frame False {
                                n476 = To Variant(anything=w1125) -> (Variant=w1126:variant)
                                n477 = property class="IZDrive"(reference=w1124, "Position"=w1126) -> ()  [unwired: 1 in, 2 out]
                                }
                                frame True {
                                n478 = To Variant(anything=w1127) -> (Variant=w1129:variant)
                                n479 = property class="IZDrive"(reference=w1128, "Position"=w1129) -> ()  [unwired: 1 in, 2 out]
                                }
                                }
                                }
                                frame #1 {
                                n480 = To Variant(anything=1) -> (Variant=w1130:variant)
                                n481 = property class="IPFS"(reference=w1133, "IsEnabled"=w1130) -> (error out=w1132:errorcluster)  [unwired: 1 in, 1 out]
                                }
                                frame #2 {
                                n482 = local read "Delay PFS"() -> (w1135:u32)
                                n483 = Wait (ms)(milliseconds to wait=w1135) -> (millisecond timer value=w1134:u32)
                                }
                                frame #3 {
                                n484 = property class="IPFS"(reference=w1142) -> (reference out=w1140:refnum<k7>, "Type"=w1143:i32, "Status"=w1144:variant)  [unwired: 1 in, 1 out]
                                n485 = Variant To Data(type=w1143, Variant=w1144) -> (data=w1139:i32)  [unwired: 1 in, 1 out]
                                n486 = local write "PFS status"(w1139) -> ()
                                n487 = case shown="0, 1, 6, Par défaut" w1139 {
                                tunnel: w1141 -> [w1149 _ w1166]
                                tunnel: w1140 -> [w1148 _ _]
                                tunnel: w1138 -> [w1147 _ _]
                                tunnel: w1137 -> [w1146 _ _]
                                tunnel: [w1145 nan w1163] -> w1136
                                frame 0, 1, 6, Default {
                                n488 = stacked-sequence {
                                tunnel: w1149 -> [_ w1158]
                                tunnel: w1148 -> [w1152 _]
                                tunnel: w1147 -> [_ w1154]
                                tunnel: w1146 -> [_ w1156]
                                tunnel: [_ nan] -> w1145
                                frame #0 {
                                n489 = To Variant(anything=0) -> (Variant=w1151:variant)
                                n490 = property class="IPFS"(reference=w1152, "IsEnabled"=w1151) -> ()  [unwired: 1 in, 2 out]
                                }
                                frame #1 {
                                n491 = Not A Number/Path/Refnum?(number/path/refnum=w1154) -> (NaN/Path/Refnum?=w1157:bool)
                                n492 = case shown="Vrai" w1157 {
                                tunnel: w1156 -> [_ w1161]
                                tunnel: [w1160 w1161] -> w1155
                                tunnel: w1154 -> [w1160 _]
                                frame False {
                                }
                                frame True {
                                }
                                }
                                n493 = To Variant(anything=w1155) -> (Variant=w1159:variant)
                                n494 = property class="IZDrive"(reference=w1158, "Position"=w1159) -> ()  [unwired: 1 in, 2 out]
                                }
                                }
                                }
                                frame 4 {
                                }
                                frame 5 {
                                n495 = property class="IZDrive"(reference=w1166) -> ("Type"=w1165:i32, "Position"=w1164:variant)  [unwired: 1 in, 2 out]
                                n496 = Variant To Data(type=w1165, Variant=w1164) -> (data=w1163:i32)  [unwired: 1 in, 1 out]
                                n497 = local write "lastgoodz"(w1163) -> ()
                                }
                                }
                                }
                                }
                              }
                              frame 4 {
                                n498 = stacked-sequence {
                                tunnel: [w1175 _] -> _
                                tunnel: [w1174 _] -> w1173
                                tunnel: w1172 -> [w1174 _]
                                tunnel: w1171 -> [_ w1182]
                                tunnel: w1170 -> [_ w1181]
                                tunnel: w1169 -> [_ w1179]
                                tunnel: w1168 -> [_ w1178]
                                tunnel: [_ w1177] -> w1167
                                frame #0 {
                                n499 = local read "Delay PFS"() -> (w1176:u32)
                                n500 = Wait (ms)(milliseconds to wait=w1176) -> (millisecond timer value=w1175:u32)
                                }
                                frame #1 {
                                n501 = property class="IPFS"(reference=w1181) -> (reference out=w1180:refnum<k7>, "Type"=w1185:i32, "Status"=w1184:variant)  [unwired: 1 in, 1 out]
                                n502 = Variant To Data(type=w1185, Variant=w1184) -> (data=w1183:i32)  [unwired: 1 in, 1 out]
                                n503 = local write "PFS status"(w1183) -> ()
                                n504 = case shown="5" w1183 {
                                tunnel: w1182 -> [w1192 w1201 w1210 _ _ w1225]
                                tunnel: w1180 -> [_ _ _ w1214 _ _]
                                tunnel: w1179 -> [w1187 w1196 w1205 w1213 w1217 _]
                                tunnel: w1178 -> [w1188 w1197 w1206 _ _ _]
                                tunnel: [nan nan nan w1213 w1218 w1222] -> w1177
                                frame 0, Default {
                                n505 = Not A Number/Path/Refnum?(number/path/refnum=w1187) -> (NaN/Path/Refnum?=w1190:bool)
                                n506 = case shown="Faux" w1190 {
                                tunnel: [w1193 w1194] -> w1189
                                tunnel: w1188 -> [_ w1194]
                                tunnel: w1187 -> [w1193 _]
                                frame False {
                                }
                                frame True {
                                }
                                }
                                n507 = To Variant(anything=w1189) -> (Variant=w1191:variant)
                                n508 = property class="IZDrive"(reference=w1192, "Position"=w1191) -> ()  [unwired: 1 in, 2 out]
                                }
                                frame 1 {
                                n509 = Not A Number/Path/Refnum?(number/path/refnum=w1196) -> (NaN/Path/Refnum?=w1199:bool)
                                n510 = case shown="Faux" w1199 {
                                tunnel: [w1202 w1203] -> w1198
                                tunnel: w1197 -> [_ w1203]
                                tunnel: w1196 -> [w1202 _]
                                frame False {
                                }
                                frame True {
                                }
                                }
                                n511 = To Variant(anything=w1198) -> (Variant=w1200:variant)
                                n512 = property class="IZDrive"(reference=w1201, "Position"=w1200) -> ()  [unwired: 1 in, 2 out]
                                }
                                frame 6 {
                                n513 = Not A Number/Path/Refnum?(number/path/refnum=w1205) -> (NaN/Path/Refnum?=w1208:bool)
                                n514 = case shown="Faux" w1208 {
                                tunnel: [w1211 w1212] -> w1207
                                tunnel: w1206 -> [_ w1212]
                                tunnel: w1205 -> [w1211 _]
                                frame False {
                                }
                                frame True {
                                }
                                }
                                n515 = To Variant(anything=w1207) -> (Variant=w1209:variant)
                                n516 = property class="IZDrive"(reference=w1210, "Position"=w1209) -> ()  [unwired: 1 in, 2 out]
                                }
                                frame 2 {
                                n517 = To Variant(anything=1) -> (Variant=w1216:variant)
                                n518 = property class="IPFS"(reference=w1214, "IsEnabled"=w1216) -> ()  [unwired: 1 in, 2 out]
                                }
                                frame 4 {
                                n519 = stacked-sequence {
                                tunnel: [w1220] -> _
                                tunnel: [w1219] -> w1218
                                tunnel: w1217 -> [w1219]
                                frame #0 {
                                n520 = local read "Delay PFS"() -> (w1221:u32)
                                n521 = Wait (ms)(milliseconds to wait=w1221) -> (millisecond timer value=w1220:u32)
                                }
                                }
                                }
                                frame 5 {
                                n522 = property class="IZDrive"(reference=w1225) -> ("Type"=w1224:i32, "Position"=w1223:variant)  [unwired: 1 in, 2 out]
                                n523 = Variant To Data(type=w1224, Variant=w1223) -> (data=w1222:i32)  [unwired: 1 in, 1 out]
                                n524 = local write "lastgoodz"(w1222) -> ()
                                }
                                }
                                }
                                }
                              }
                              frame 5 {
                                n525 = property class="IZDrive"(reference=w1229) -> (error out=w1228:errorcluster, "Type"=w1231:i32, "Position"=w1230:variant)  [unwired: 1 in, 1 out]
                                n526 = Variant To Data(error in=w1228, type=w1231, Variant=w1230) -> (data=w1226:i32, error out=w1227:errorcluster)
                                n527 = local write "lastgoodz"(w1226) -> ()
                              }
                            }
                            n528 = Replace Array Subset(array=w963, new element=w961, index (row)=w962, index (col)=0) -> (w964:T1)
                            n529 = local write "lastgoodz_list"(w964) -> ()
                          }
                          frame #3 {
                            n530 = Initialize Array(FALSE, 12) -> (w1241:bool[])
                            n531 = call-poly <vilib>:"DAQmx Write.vi"("task/channels in"=w1235, "data"=0.0, "error in"=w1234) -> ("task out"=w1233:refnum<k21>, "error out"=w1232:errorcluster)  [unwired: 10 in, 1 out]
                            n532 = call-poly <vilib>:"DAQmx Write.vi"("task/channels in"=w1240, "data"=w1241, "error in"=w1239) -> ("task out"=w1238:refnum<k21>, "error out"=w1237:errorcluster)  [unwired: 10 in, 1 out]
                          }
                          frame #4 {
                            n533 = while {
                              tunnel: w1272 -> [w1305]
                              tunnel: w1271 -> [w1304]
                              tunnel: w1270 -> [w1303]
                              tunnel: [w1302] -> w1269
                              tunnel: w1268 -> [w1301]
                              tunnel: w1267 -> [w1300]
                              tunnel: w1244 -> [w1299]
                              tunnel: w1266 -> [w1298]
                              tunnel: w1265 -> [w1297]
                              tunnel: [w1296] -> w1264
                              tunnel: [w1295] -> w1263
                              tunnel: [w1294] -> w1262
                              tunnel: [w1293] -> w1261
                              tunnel: w1260 -> [w1289]
                              tunnel: w1259 -> [w1288]
                              tunnel: [w1287] -> w1258
                              tunnel: [w1286] -> w1257
                              tunnel: w1256 -> [w1285]
                              tunnel: w1255 -> [w1284]
                              tunnel: [w1283] -> w1254
                              tunnel: [w1282] -> w1253
                              tunnel: w1252 -> [w1281]
                              tunnel: w1251 -> [w1280]
                              tunnel: [w1279] -> w1250
                              tunnel: w1249 -> [w1278]
                              tunnel: w1248 -> [w1277]
                              tunnel: [w1276] -> w1247
                              tunnel: [w1275] -> w1246
                              tunnel: w1245 -> [w1274]
                              tunnel: w1244 -> [w1273]
                              i -> [w1290]
                              stop <- w1307 stop-if-true
                              n534 = local read "Total Number of Patterns"() -> (w1291:u32)
                              n535 = stacked-sequence {
                                seq-local: [_ w1388 _ _ _] -> [_ _ _ w1505 _]
                                seq-local: [_ w1387 _ _ _] -> [_ _ _ w1504 _]
                                seq-local: [_ w1383 _ _ _] -> [_ _ w1496 _ _]
                                seq-local: [_ w1382 _ _ _] -> [_ _ w1495 _ _]
                                tunnel: w1290 -> [w1317 _ _ _ w1535]
                                tunnel: w1305 -> [_ _ _ _ _]
                                tunnel: w1304 -> [_ _ _ _ _]
                                tunnel: w1303 -> [_ w1397 _ _ _]
                                tunnel: [_ w1396 _ _ _] -> w1302
                                tunnel: w1301 -> [_ w1395 _ _ _]
                                tunnel: w1300 -> [_ w1394 _ _ _]
                                tunnel: w1299 -> [_ w1393 _ _ _]
                                tunnel: w1298 -> [_ w1392 _ _ _]
                                tunnel: w1297 -> [_ w1391 _ _ _]
                                tunnel: [_ w1390 _ _ _] -> w1296
                                tunnel: [_ w1389 _ _ _] -> w1295
                                tunnel: [_ _ _ w1503 _] -> w1294
                                tunnel: [_ _ _ w1502 _] -> w1293
                                tunnel: w1289 -> [_ w1385 _ _ _]
                                tunnel: w1288 -> [_ w1384 _ _ _]
                                tunnel: [_ _ w1493 _ _] -> w1287
                                tunnel: [_ _ w1494 _ _] -> w1286
                                tunnel: w1285 -> [w1316 _ _ _ _]
                                tunnel: w1284 -> [w1315 _ _ _ _]
                                tunnel: [w1314 _ _ _ _] -> w1283
                                tunnel: [w1313 _ _ _ _] -> w1282
                                tunnel: w1281 -> [_ w1381 _ _ _]
                                tunnel: w1280 -> [_ w1380 _ _ _]
                                tunnel: [_ w1379 _ _ _] -> w1279
                                tunnel: w1278 -> [_ w1378 _ _ _]
                                tunnel: w1277 -> [_ w1377 _ _ _]
                                tunnel: [_ w1376 _ _ _] -> w1276
                                tunnel: [_ w1375 _ _ _] -> w1275
                                tunnel: w1274 -> [w1312 _ _ _ _]
                                tunnel: w1273 -> [w1311 _ _ _ _]
                                frame #0 {
                                n536 = local read "useLASER_TL"() -> (w1310:bool)
                                n537 = case shown="Vrai" w1310 {
                                tunnel: w1317 -> [_ w1327]
                                tunnel: w1316 -> [w1319 w1326]
                                tunnel: w1315 -> [w1318 w1325]
                                tunnel: [w1319 w1324] -> w1314
                                tunnel: [w1318 w1323] -> w1313
                                tunnel: w1312 -> [_ w1321]
                                tunnel: w1311 -> [_ w1320]
                                frame False {
                                }
                                frame True {
                                n538 = local read "is_single_shoot"() -> (w1322:bool)
                                n539 = case shown="Vrai" w1322 {
                                tunnel: w1327 -> [w1345 _]
                                tunnel: w1326 -> [w1331 w1354]
                                tunnel: w1325 -> [w1330 w1353]
                                tunnel: [w1329 w1350] -> w1324
                                tunnel: [w1328 w1349] -> w1323
                                tunnel: w1321 -> [_ w1352]
                                tunnel: w1320 -> [_ w1351]
                                frame False {
                                # "motif index"
                                # "number of motif done"
                                n540 = local read "Non"() -> (w1338:u32)
                                n541 = local read "Noff"() -> (w1344:u32)
                                n542 = local read "Nstart"() -> (w1346:u32)
                                n543 = Add(x=w1338, y=w1344) -> (x+y=w1341:u32)
                                n544 = Subtract(x=w1345, y=w1346) -> (x-y=w1337:u32)
                                n545 = Divide(x=w1337, y=w1341) -> (x/y=w1343:dbl)
                                n546 = Greater Or Equal To 0?(x=w1337) -> (x >= 0?=w1335:bool)
                                n547 = Round Toward -Infinity(1:w1343) -> (0:w1342:dbl)
                                n548 = Multiply(x=w1342, y=w1341) -> (x*y=w1340:dbl)
                                n549 = Subtract(x=w1337, y=w1340) -> (x-y=w1339:dbl)
                                n550 = Greater Or Equal?(x=w1339, y=w1338) -> (x >= y?=w1336:bool)
                                n551 = Or(x=w1336, y=w1335) -> (x .or. y?=w1334:bool)
                                n552 = Not(x=w1334) -> (.not. x?=w1333:bool)
                                n553 = case shown="Faux" w1333 {
                                tunnel: [0.0 5.0] -> w1332
                                frame False {
                                }
                                frame True {
                                }
                                }
                                n554 = local write "TL Laser shutter"(w1333) -> ()
                                n555 = call-poly <vilib>:"DAQmx Write.vi"("task/channels in"=w1331, "data"=w1332, "error in"=w1330) -> ("task out"=w1329:refnum<k21>, "error out"=w1328:errorcluster)  [unwired: 10 in, 1 out]
                                }
                                frame True {
                                n556 = stacked-sequence {
                                tunnel: w1354 -> [w1367 _]
                                tunnel: w1353 -> [w1366 _]
                                tunnel: w1352 -> [w1364 _]
                                tunnel: w1351 -> [w1362 _]
                                tunnel: [w1356 _] -> w1350
                                tunnel: [w1355 _] -> w1349
                                tunnel: [_ w1370] -> _
                                frame #0 {
                                n557 = local read "Shoot at Scan#"() -> (w1365:i32)
                                n558 = local read "shooted_ positions"() -> (w1363:bool[][])
                                n559 = Equal?(x=w1365, y=w1364) -> (x = y?=w1360:bool)
                                n560 = Index Array(array=w1363, index (row)=w1362, index (col)=0) -> (element=w1361:bool)
                                n561 = And(x=w1361, y=w1360) -> (x .and. y?=w1357:bool)
                                n562 = case shown="Vrai" w1357 {
                                tunnel: [0.0 5.0] -> w1358
                                frame False {
                                }
                                frame True {
                                }
                                }
                                n563 = local write "TL Laser shutter"(w1357) -> ()
                                n564 = call-poly <vilib>:"DAQmx Write.vi"("task/channels in"=w1367, "data"=w1358, "error in"=w1366) -> ("task out"=w1356:refnum<k21>, "error out"=w1355:errorcluster)  [unwired: 10 in, 1 out]
                                }
                                frame #1 {
                                n565 = local read "Shoot duration"() -> (w1374:dbl)
                                n566 = Multiply(x=w1374, y=1000.0) -> (x*y=w1372:dbl)
                                n567 = To Unsigned Long Integer(number=w1372) -> (unsigned 32bit integer=w1371:u32)
                                n568 = Wait Until Next ms Multiple(millisecond multiple=w1371) -> (millisecond timer value=w1370:u32)
                                }
                                }
                                }
                                }
                                }
                                }
                                }
                                frame #1 {
                                n569 = local read "TL_NCAN"() -> (w1386:u8)
                                n570 = for {
                                N: w1386 -> [_]
                                tunnel: w1397 -> [w1419]
                                tunnel: [w1418] -> w1396
                                tunnel: w1395 -> [w1417]
                                tunnel: w1394 -> [w1416]
                                tunnel: w1393 -> [w1415]
                                tunnel: w1392 -> [w1414]
                                tunnel: w1391 -> [w1413]
                                tunnel: [w1412] -> w1390
                                tunnel: [w1411] -> w1389
                                tunnel: [w1410] -> w1388
                                tunnel: [w1409] -> w1387
                                tunnel: w1385 -> [w1408]
                                tunnel: w1384 -> [w1407]
                                tunnel: [w1406] -> w1383
                                tunnel: [w1405] -> w1382
                                tunnel: w1381 -> [w1404]
                                tunnel: w1380 -> [w1403]
                                tunnel: [w1402] -> w1379
                                tunnel: w1378 -> [w1401]
                                tunnel: w1377 -> [w1400]
                                tunnel: [w1399] -> w1376
                                tunnel: [w1398] -> w1375
                                i -> [w1420]
                                n571 = stacked-sequence {
                                seq-local: [_ _ w1452 _ _] -> [_ _ _ _ w1489]
                                seq-local: [_ _ w1451 _ _] -> [_ _ _ _ w1488]
                                tunnel: w1420 -> [w1426 _ w1450 w1465 _]
                                tunnel: w1419 -> [w1425 _ _ _ _]
                                tunnel: [w1424 _ _ _ _] -> w1418
                                tunnel: w1417 -> [_ _ _ w1485 _]
                                tunnel: w1416 -> [_ _ _ w1484 _]
                                tunnel: w1415 -> [_ _ _ w1467 _]
                                tunnel: w1414 -> [_ _ _ w1473 _]
                                tunnel: w1413 -> [_ _ _ w1472 _]
                                tunnel: [_ _ _ w1471 _] -> w1412
                                tunnel: [_ _ _ w1470 _] -> w1411
                                tunnel: [_ _ _ w1469 _] -> w1410
                                tunnel: [_ _ _ w1468 _] -> w1409
                                tunnel: w1408 -> [_ _ w1454 _ _]
                                tunnel: w1407 -> [_ _ w1453 _ _]
                                tunnel: [_ _ _ _ w1487] -> w1406
                                tunnel: [_ _ _ _ w1486] -> w1405
                                tunnel: w1404 -> [_ w1449 _ _ _]
                                tunnel: w1403 -> [_ w1439 _ _ _]
                                tunnel: [_ w1438 _ _ _] -> w1402
                                tunnel: w1401 -> [_ _ _ w1462 _]
                                tunnel: w1400 -> [_ _ _ w1461 _]
                                tunnel: [_ _ _ w1460 _] -> w1399
                                tunnel: [_ _ _ w1459 _] -> w1398
                                frame #0 {
                                n572 = local read "used Filters"() -> (w1423:u8[])
                                n573 = Index Array(array=w1423, index=w1426) -> (element=w1422:u8)
                                n574 = stacked-sequence {
                                tunnel: w1425 -> [w1429 w1435 _]
                                tunnel: [w1428 _ _] -> w1424
                                tunnel: w1422 -> [w1427 _ _]
                                tunnel: [_ w1431 _] -> w1421
                                tunnel: [_ _ w1437] -> _
                                frame #0 {
                                n575 = To Variant(anything=w1427) -> (Variant=w1430:variant)
                                n576 = property class="IFilterBlockCassette"(reference=w1429, "Position"=w1430) -> (reference out=w1428:refnum<k7>)  [unwired: 1 in, 1 out]
                                }
                                frame #1 {
                                n577 = property class="IFilterBlockCassette"(reference=w1435) -> ("Position"=w1433:variant, "Type"=w1434:i32)  [unwired: 1 in, 2 out]
                                n578 = Variant To Data(type=w1434, Variant=w1433) -> (data=w1432:i32)  [unwired: 1 in, 1 out]
                                n579 = To Unsigned Byte Integer(number=w1432) -> (unsigned 8bit integer=w1431:u8)
                                }
                                frame #2 {
                                n580 = local read "Delay after Fluo. cube change"() -> (w1436:u32)
                                n581 = Wait (ms)(milliseconds to wait=w1436) -> (millisecond timer value=w1437:u32)
                                }
                                }
                                n582 = local write "Lower Filter"(w1421) -> ()
                                }
                                frame #1 {
                                n583 = property class="IZDrive"(reference=w1449, error in=w1439) -> ("Position"=w1448:variant, "Type"=w1445:i32, "Resolution"=w1446:variant)  [unwired: 2 out]
                                n584 = Variant To Data(type=w1445, Variant=w1446) -> (data=w1444:i32)  [unwired: 1 in, 1 out]
                                n585 = Variant To Data(type=w1445, Variant=w1448) -> (data=w1447:i32, error out=w1438:errorcluster)  [unwired: 1 in]
                                n586 = Multiply(x=w1447, y=w1444) -> (x*y=w1443:i32)
                                n587 = To Double Precision Float(number=w1443) -> (double precision float=w1442:dbl)
                                n588 = Divide(x=w1442, y=1000.0) -> (x/y=w1440:dbl)
                                n589 = local write "Z position"(w1440) -> ()
                                }
                                frame #2 {
                                n590 = local read "used LEDs"() -> (w1456:bool[][])
                                n591 = Index Array(array=w1456, index (row)=w1450) -> (element=w1455:bool[])  [unwired: 1 in]
                                n592 = call-poly <vilib>:"DAQmx Write.vi"("task/channels in"=w1454, "data"=w1455, "error in"=w1453) -> ("task out"=w1452:refnum<k21>, "error out"=w1451:errorcluster)  [unwired: 10 in, 1 out]
                                }
                                frame #3 {
                                n593 = local read "Current Directory"() -> (w1475:path)
                                n594 = local read "Buffer Info"() -> (w1481:T2)
                                n595 = call <userlib>:"tm_firetrigger.vi"("error in (no error)"=w1484, "Handle in"=w1485) -> ("error out"=w1483:errorcluster, "Handle out"=w1482:u32)  [unwired: 8 in]
                                n596 = call <userlib>:"tm_waitnextframe.vi"("error in (no error)"=w1483, "Handle in"=w1482) -> ("error out"=w1478:errorcluster, "Frame Index"=w1479:i32, "Handle out"=w1480:u32)  [unwired: 6 in, 1 out]
                                n597 = To Unsigned Byte Integer(number=w1465) -> (unsigned 8bit integer=w1464:u8)
                                n598 = call <userlib>:"tm_getframe_a.vi"("error in (no error)"=w1478, "Frame Index"=w1479, "Buffer Info"=w1481, "Handle in"=w1480) -> ("error out"=w1468:errorcluster, "Data 16"=w1477:u16[][], "Handle out"=w1469:u32)  [unwired: 3 in, 2 out]
                                n599 = local write "Intensity Graph"(w1477) -> ()
                                n600 = To Unsigned Long Integer(number=w1467) -> (unsigned 32bit integer=w1466:u32)
                                n601 = call "svi_write_image_XYscan.vi"("Position num"=w1466, "chanel num"=w1464, "image in"=w1477, "Chemin"=w1475) -> ()  [unwired: 8 in]
                                n602 = local read "TL Fluidic SYNC"() -> (w1463:bool)
                                n603 = local read "TL Laser shutter"() -> (w1474:bool)
                                n604 = local read "Z position"() -> (w1476:dbl)
                                n605 = call-poly <vilib>:"DAQmx Read.vi"("task/channels in"=w1462, "error in"=w1461) -> ("task out"=w1460:refnum<k21>, "data"=w1457:dbl, "error out"=w1459:errorcluster)  [unwired: 11 in]
                                n606 = call-poly <vilib>:"DAQmx Read.vi"("task/channels in"=w1472, "error in"=w1473) -> ("task out"=w1471:refnum<k21>, "data"=w1458:dbl, "error out"=w1470:errorcluster)  [unwired: 11 in]
                                n607 = call "svi_write_ext_in.vi"("shutter en entrée"=w1463, "position num"=w1466, "power value"=w1458, "pdir_path"=w1475, "shutter 1"=w1474, "z value"=w1476, "power value 2"=w1457, "chanel num"=w1464) -> ()  [unwired: 3 in, 1 out]
                                n608 = local write "FlowRate (mL/min)"(w1457) -> ()
                                n609 = local write "Laser Power (a.u.)"(w1458) -> ()
                                }
                                frame #4 {
                                n610 = Initialize Array(FALSE, 12) -> (w1490:bool[])
                                n611 = call-poly <vilib>:"DAQmx Write.vi"("task/channels in"=w1489, "data"=w1490, "error in"=w1488) -> ("task out"=w1487:refnum<k21>, "error out"=w1486:errorcluster)  [unwired: 10 in, 1 out]
                                }
                                }
                                }
                                }
                                frame #2 {
                                n612 = Initialize Array(FALSE, 12) -> (w1497:bool[])
                                n613 = call-poly <vilib>:"DAQmx Write.vi"("task/channels in"=w1496, "data"=w1497, "error in"=w1495) -> ("task out"=w1493:refnum<k21>, "error out"=w1494:errorcluster)  [unwired: 10 in, 1 out]
                                }
                                frame #3 {
                                n614 = local read "Frames between Patterns"() -> (w1500:u32)
                                n615 = Greater Than 0?(x=w1500) -> (x > 0?=w1501:bool)
                                n616 = case shown="Vrai" w1501 {
                                tunnel: w1505 -> [w1507 w1512]
                                tunnel: w1504 -> [w1506 w1511]
                                tunnel: [w1507 w1510] -> w1503
                                tunnel: [w1506 w1509] -> w1502
                                tunnel: w1500 -> [_ w1508]
                                frame False {
                                }
                                frame True {
                                n617 = while {
                                tunnel: w1512 -> [w1531]
                                tunnel: w1511 -> [w1530]
                                tunnel: [w1523] -> w1510
                                tunnel: [w1522] -> w1509
                                tunnel: w1508 -> [w1519]
                                i -> [w1513]
                                stop <- w1532 stop-if-true
                                n618 = To Long Integer(number=w1519) -> (32bit integer=w1514:i32)
                                n619 = local read "Buffer Info"() -> (w1520:T2)
                                n620 = Decrement(x=w1514) -> (x-1=w1521:i32)
                                n621 = Greater Or Equal?(x=w1513, y=w1521) -> (x >= y?=w1534:bool)
                                n622 = call <userlib>:"tm_firetrigger.vi"("error in (no error)"=w1530, "Handle in"=w1531) -> ("error out"=w1528:errorcluster, "Handle out"=w1529:u32)  [unwired: 8 in]
                                n623 = call <userlib>:"tm_waitnextframe.vi"("error in (no error)"=w1528, "Handle in"=w1529) -> ("error out"=w1526:errorcluster, "Frame Index"=w1525:i32, "Handle out"=w1527:u32)  [unwired: 6 in, 1 out]
                                n624 = local read "pause TL"() -> (w1533:bool)
                                n625 = call <userlib>:"tm_getframe_a.vi"("error in (no error)"=w1526, "Frame Index"=w1525, "Buffer Info"=w1520, "Handle in"=w1527) -> ("error out"=w1522:errorcluster, "Data 16"=w1524:u16[][], "Handle out"=w1523:u32)  [unwired: 3 in, 2 out]
                                n626 = local write "Intensity Graph"(w1524) -> ()
                                n627 = Increment(x=w1513) -> (x+1=w1515:i32)
                                n628 = Divide(x=w1515, y=w1514) -> (x/y=w1517:dbl)
                                n629 = Or(x=w1533, y=w1534) -> (x .or. y?=w1532:bool)
                                n630 = Multiply(x=w1517, y=100) -> (x*y=w1516:dbl)
                                n631 = local write "Next Pattern"(w1516) -> ()
                                }
                                }
                                }
                                }
                                frame #4 {
                                n632 = Increment(x=w1535) -> (x+1=w1537:i32)
                                n633 = To Unsigned Long Integer(number=w1537) -> (unsigned 32bit integer=w1536:u32)
                                n634 = local write "Recorded\nPatterns"(w1536) -> ()
                                }
                              }
                              n635 = To Long Integer(number=w1291) -> (32bit integer=w1292:i32)
                              n636 = Decrement(x=w1292) -> (x-1=w1309:i32)
                              n637 = Greater Or Equal?(x=w1290, y=w1309) -> (x >= y?=w1308:bool)
                              n638 = local read "pause TL"() -> (w1306:bool)
                              n639 = Or(x=w1308, y=w1306) -> (x .or. y?=w1307:bool)
                            }
                          }
                          frame #5 {
                            n640 = Initialize Array(FALSE, 12) -> (w1545:bool[])
                            n641 = call-poly <vilib>:"DAQmx Write.vi"("task/channels in"=w1541, "data"=0.0, "error in"=w1540) -> ("task out"=w1539:refnum<k21>, "error out"=w1538:errorcluster)  [unwired: 10 in, 1 out]
                            n642 = call-poly <vilib>:"DAQmx Write.vi"("task/channels in"=w1549, "data"=w1545, "error in"=w1548) -> ("task out"=w1544:refnum<k21>, "error out"=w1543:errorcluster)  [unwired: 10 in, 1 out]
                          }
                        }
                      }
                    }
                    frame #2 {
                      w1559 = 0
                      n643 = local read "stored XY"() -> (w1561:T1)
                      n644 = Index Array(array=w1561, index (row)=w1559, index (col)=w1559) -> (element=w1557:dbl)
                      n645 = Index Array(array=w1561, index (row)=w1559, index (col)=1) -> (element=w1558:dbl)
                      n646 = Multiply(x=w1557, y=10) -> (x*y=w1554:dbl)
                      n647 = To Long Integer(number=w1554) -> (32bit integer=w1552:i32)
                      n648 = Multiply(x=w1558, y=10) -> (x*y=w1553:dbl)
                      n649 = To Long Integer(number=w1553) -> (32bit integer=w1551:i32)
                      n650 = call "SerialMoveXY.vi"("error in (no error)"=w1562, "Y"=w1551, "X"=w1552) -> ("error out"=w1550:errorcluster)  [unwired: 2 in]
                    }
                    frame #3 {
                      n651 = local read "Frames between Scan"() -> (w1563:u32)
                      n652 = Greater Than 0?(x=w1563) -> (x > 0?=w1564:bool)
                      n653 = case shown="Vrai" w1564 {
                        tunnel: w1568 -> [w1570 w1575]
                        tunnel: w1567 -> [w1569 w1574]
                        tunnel: [w1570 w1573] -> w1566
                        tunnel: [w1569 w1572] -> w1565
                        tunnel: w1563 -> [_ w1571]
                        frame False {
                        }
                        frame True {
                          n654 = while {
                            tunnel: w1575 -> [w1593]
                            tunnel: w1574 -> [w1592]
                            tunnel: [w1584] -> w1573
                            tunnel: [w1583] -> w1572
                            tunnel: w1571 -> [w1581]
                            i -> [w1580]
                            stop <- w1594 stop-if-true
                            n655 = To Long Integer(number=w1581) -> (32bit integer=w1582:i32)
                            n656 = Decrement(x=w1582) -> (x-1=w1597:i32)
                            n657 = Greater Or Equal?(x=w1580, y=w1597) -> (x >= y?=w1595:bool)
                            n658 = Increment(x=w1580) -> (x+1=w1579:i32)
                            n659 = local read "Buffer Info"() -> (w1586:T2)
                            n660 = call <userlib>:"tm_firetrigger.vi"("error in (no error)"=w1592, "Handle in"=w1593) -> ("error out"=w1590:errorcluster, "Handle out"=w1591:u32)  [unwired: 8 in]
                            n661 = call <userlib>:"tm_waitnextframe.vi"("error in (no error)"=w1590, "Handle in"=w1591) -> ("error out"=w1588:errorcluster, "Frame Index"=w1589:i32, "Handle out"=w1587:u32)  [unwired: 6 in, 1 out]
                            n662 = local read "pause TL"() -> (w1596:bool)
                            n663 = call <userlib>:"tm_getframe_a.vi"("error in (no error)"=w1588, "Frame Index"=w1589, "Buffer Info"=w1586, "Handle in"=w1587) -> ("error out"=w1583:errorcluster, "Data 16"=w1585:u16[][], "Handle out"=w1584:u32)  [unwired: 3 in, 2 out]
                            n664 = Divide(x=w1579, y=w1581) -> (x/y=w1578:dbl)
                            n665 = local write "Intensity Graph"(w1585) -> ()
                            n666 = Multiply(x=w1578, y=100) -> (x*y=w1577:dbl)
                            n667 = Or(x=w1596, y=w1595) -> (x .or. y?=w1594:bool)
                            n668 = local write "Next Scan"(w1577) -> ()
                          }
                        }
                      }
                    }
                    frame #4 {
                      n669 = Increment(x=w1599) -> (x+1=w1600:i32)
                      n670 = To Unsigned Long Integer(number=w1600) -> (unsigned 32bit integer=w1598:u32)
                      n671 = local write "Recorded Scans"(w1598) -> ()
                    }
                  }
                  n672 = local read "Total Number of Scan"() -> (w829:u32)
                  n673 = To Long Integer(number=w829) -> (32bit integer=w828:i32)
                  n674 = Decrement(x=w828) -> (x-1=w849:i32)
                  n675 = Greater Or Equal?(x=w816, y=w849) -> (x >= y?=w847:bool)
                  n676 = local read "pause TL"() -> (w846:bool)
                  n677 = Or(x=w846, y=w847) -> (x .or. y?=w848:bool)
                  n678 = node-c288() -> ()  [unwired: 1 in, 1 out]
                }
                n679 = node-c288(w782) -> ()  [unwired: 1 out]
              }
              frame #3 {
                w1617 = 0
                w1628 = 0
                w1614 = FALSE
                n680 = local read "stored XY"() -> (w1630:T1)
                n681 = local write "TL Laser shutter"(w1614) -> ()
                n682 = local write "pause TL"(w1614) -> ()
                n683 = local write "TLON"(w1614) -> ()
                n684 = Index Array(array=w1630, index (row)=w1628, index (col)=w1628) -> (element=w1625:dbl)
                n685 = local write "Next Scan"(w1617) -> ()
                n686 = local write "Next Pattern"(w1617) -> ()
                n687 = Index Array(array=w1630, index (row)=w1628, index (col)=1) -> (element=w1627:dbl)
                n688 = local write "LASER shutter"(w1614) -> ()
                n689 = Multiply(x=w1625, y=10) -> (x*y=w1623:dbl)
                n690 = To Long Integer(number=w1623) -> (32bit integer=w1620:i32)
                n691 = Multiply(x=w1627, y=10) -> (x*y=w1622:dbl)
                n692 = To Long Integer(number=w1622) -> (32bit integer=w1621:i32)
                n693 = call "SerialMoveXY.vi"("error in (no error)"=w1619, "Y"=w1621, "X"=w1620) -> ("error out"=w1618:errorcluster)  [unwired: 2 in]
                n694 = stacked-sequence {
                  tunnel: w1616 -> [w1632 _ _ _ _]
                  tunnel: w1615 -> [w1631 _ _ _ _]
                  tunnel: w1613 -> [_ w1639 _ _ _]
                  tunnel: w1612 -> [_ w1638 _ _ _]
                  tunnel: w1611 -> [_ _ w1646 _ _]
                  tunnel: w1610 -> [_ _ w1645 _ _]
                  tunnel: w1609 -> [_ _ _ w1650 _]
                  tunnel: w1608 -> [_ _ _ w1649 _]
                  tunnel: w1607 -> [_ _ _ _ w1654]
                  tunnel: w1606 -> [_ _ _ _ w1653]
                  frame #0 {
                    n695 = call-poly <vilib>:"DAQmx Write.vi"("task/channels in"=w1632, "data"=0.0, "error in"=w1631) -> ("task out"=w1633:refnum<k21>, "error out"=w1634:errorcluster)  [unwired: 10 in, 1 out]
                    n696 = call <vilib>:"DAQmx Stop Task.vi"("task/channels in"=w1633, "error in"=w1634) -> ("task out"=w1637:refnum<k21>, "error out"=w1636:errorcluster)  [unwired: 12 in]
                    n697 = call <vilib>:"DAQmx Clear Task.vi"("task in"=w1637, "error in"=w1636) -> ()  [unwired: 13 in, 1 out]
                  }
                  frame #1 {
                    n698 = call-poly <vilib>:"DAQmx Write.vi"("task/channels in"=w1638, "data"=0.0, "error in"=w1639) -> ("task out"=w1644:refnum<k21>, "error out"=w1643:errorcluster)  [unwired: 10 in, 1 out]
                    n699 = call <vilib>:"DAQmx Stop Task.vi"("task/channels in"=w1644, "error in"=w1643) -> ("task out"=w1640:refnum<k21>, "error out"=w1641:errorcluster)  [unwired: 12 in]
                    n700 = call <vilib>:"DAQmx Clear Task.vi"("task in"=w1640, "error in"=w1641) -> ()  [unwired: 13 in, 1 out]
                  }
                  frame #2 {
                    n701 = call <vilib>:"DAQmx Stop Task.vi"("task/channels in"=w1646, "error in"=w1645) -> ("task out"=w1647:refnum<k21>, "error out"=w1648:errorcluster)  [unwired: 12 in]
                    n702 = call <vilib>:"DAQmx Clear Task.vi"("task in"=w1647, "error in"=w1648) -> ()  [unwired: 13 in, 1 out]
                  }
                  frame #3 {
                    n703 = call <vilib>:"DAQmx Stop Task.vi"("task/channels in"=w1650, "error in"=w1649) -> ("task out"=w1652:refnum<k21>, "error out"=w1651:errorcluster)  [unwired: 12 in]
                    n704 = call <vilib>:"DAQmx Clear Task.vi"("task in"=w1652, "error in"=w1651) -> ()  [unwired: 13 in, 1 out]
                  }
                  frame #4 {
                    n705 = call <vilib>:"DAQmx Stop Task.vi"("task/channels in"=w1654, "error in"=w1653) -> ("task out"=w1656:refnum<k21>, "error out"=w1655:errorcluster)  [unwired: 12 in]
                    n706 = call <vilib>:"DAQmx Clear Task.vi"("task in"=w1656, "error in"=w1655) -> ()  [unwired: 13 in, 1 out]
                  }
                }
              }
            }
          }
        }
      }
      event "is_single_shoot": Value Change {
        n707 = event-data() -> ("NewVal"=w1657:bool)  [unwired: 1 in, 5 out]
        n708 = case shown="Vrai" w1657 {
          frame True {
            w1660 = 2
            w1661 = 0
            w1669 = u32 0
            n709 = local write "Total Number of Patterns"(w1669) -> ()
            n710 = local write "Total Number of Scan"(u32 150) -> ()
            n711 = local write "Frames between Patterns"(w1669) -> ()
            n712 = local write "Shoot duration"(60.0) -> ()
            n713 = local write "Shoot at Scan#"(1) -> ()
            n714 = Build Array(0) -> (w1662:T1)
            n715 = Initialize Array(TRUE, 1, 0) -> (w1663:bool[][])
            n716 = local write "shooted_ positions"(w1663) -> ()
            n717 = property on="Position to add" class="NumNb (strict)"("DisabledEnum"=w1661) -> ()  [unwired: 2 in, 2 out]
            n718 = property on="Shoot at Scan#" class="NumNb (strict)"("DisabledEnum"=w1661) -> ()  [unwired: 2 in, 2 out]
            n719 = property on="Shoot duration" class="NumNb (strict)"("DisabledEnum"=w1661) -> ()  [unwired: 2 in, 2 out]
            n720 = property on="ADD ALL\nPositions" class="Bool (strict)"("DisabledEnum"=w1661) -> ()  [unwired: 2 in, 2 out]
            n721 = property on="RESET POS" class="Bool (strict)"("DisabledEnum"=w1661) -> ()  [unwired: 2 in, 2 out]
            n722 = property on="ADD\nPosition" class="Bool (strict)"("DisabledEnum"=w1661) -> ()  [unwired: 2 in, 2 out]
            n723 = local write "shoot_list"(w1662) -> ()
            n724 = property on="Frames between Patterns" class="NumNb (strict)"("DisabledEnum"=w1660) -> ()  [unwired: 2 in, 2 out]
            n725 = property on="Total Number of Patterns" class="NumNb (strict)"("DisabledEnum"=w1660) -> ()  [unwired: 2 in, 2 out]
            n726 = property on="Nstart" class="NumNb (strict)"("DisabledEnum"=w1660) -> ()  [unwired: 2 in, 2 out]
            n727 = property on="Noff" class="NumNb (strict)"("DisabledEnum"=w1660) -> ()  [unwired: 2 in, 2 out]
            n728 = property on="Non" class="NumNb (strict)"("DisabledEnum"=w1660) -> ()  [unwired: 2 in, 2 out]
          }
          frame False {
            w1672 = 2
            w1671 = 0
            n729 = local write "Total Number of Patterns"(u32 180) -> ()
            n730 = local write "Total Number of Scan"(0) -> ()
            n731 = local write "Frames between Patterns"(u32 0) -> ()
            n732 = property on="Noff FLUIDICS" class="NumNb (strict)"("DisabledEnum"=w1671) -> ()  [unwired: 2 in, 2 out]
            n733 = property on="Total Number of Patterns" class="NumNb (strict)"("DisabledEnum"=w1671) -> ()  [unwired: 2 in, 2 out]
            n734 = property on="Non FLUIDICS" class="NumNb (strict)"("DisabledEnum"=w1671) -> ()  [unwired: 2 in, 2 out]
            n735 = property on="Frames between Patterns" class="NumNb (strict)"("DisabledEnum"=w1671) -> ()  [unwired: 2 in, 2 out]
            n736 = property on="Nstart FLUIDICS" class="NumNb (strict)"("DisabledEnum"=w1671) -> ()  [unwired: 2 in, 2 out]
            n737 = property on="ADD ALL\nPositions" class="Bool (strict)"("DisabledEnum"=w1672) -> ()  [unwired: 2 in, 2 out]
            n738 = property on="RESET POS" class="Bool (strict)"("DisabledEnum"=w1672) -> ()  [unwired: 2 in, 2 out]
            n739 = property on="Shoot duration" class="NumNb (strict)"("DisabledEnum"=w1672) -> ()  [unwired: 2 in, 2 out]
            n740 = property on="Shoot at Scan#" class="NumNb (strict)"("DisabledEnum"=w1672) -> ()  [unwired: 2 in, 2 out]
            n741 = property on="ADD\nPosition" class="Bool (strict)"("DisabledEnum"=w1672) -> ()  [unwired: 2 in, 2 out]
            n742 = property on="Position to add" class="NumNb (strict)"("DisabledEnum"=w1672) -> ()  [unwired: 2 in, 2 out]
          }
        }
      }
      event "useLASER_TL": Value Change {
        n743 = event-data() -> ("NewVal"=w1675:bool)  [unwired: 1 in, 5 out]
        n744 = case shown="Faux" w1675 {
          frame True {
            w1680 = 2
            w1681 = 0
            w1689 = u32 0
            n745 = local write "Total Number of Patterns"(w1689) -> ()
            n746 = local write "Frames between Patterns"(w1689) -> ()
            n747 = local write "Total Number of Scan"(u32 150) -> ()
            n748 = local write "Shoot duration"(60.0) -> ()
            n749 = local write "is_single_shoot"(TRUE) -> ()
            n750 = local write "Shoot at Scan#"(1) -> ()
            n751 = Build Array(0) -> (w1682:T1)
            n752 = Initialize Array(TRUE, 1, 0) -> (w1683:bool[][])
            n753 = local write "shooted_ positions"(w1683) -> ()
            n754 = property on="Position to add" class="NumNb (strict)"("DisabledEnum"=w1681) -> ()  [unwired: 2 in, 2 out]
            n755 = property on="Shoot at Scan#" class="NumNb (strict)"("DisabledEnum"=w1681) -> ()  [unwired: 2 in, 2 out]
            n756 = property on="Shoot duration" class="NumNb (strict)"("DisabledEnum"=w1681) -> ()  [unwired: 2 in, 2 out]
            n757 = property on="ADD ALL\nPositions" class="Bool (strict)"("DisabledEnum"=w1681) -> ()  [unwired: 2 in, 2 out]
            n758 = property on="RESET POS" class="Bool (strict)"("DisabledEnum"=w1681) -> ()  [unwired: 2 in, 2 out]
            n759 = property on="ADD\nPosition" class="Bool (strict)"("DisabledEnum"=w1681) -> ()  [unwired: 2 in, 2 out]
            n760 = property on="is_single_shoot" class="Bool (strict)"("DisabledEnum"=0) -> ()  [unwired: 2 in, 2 out]
            n761 = local write "shoot_list"(w1682) -> ()
            n762 = property on="Frames between Patterns" class="NumNb (strict)"("DisabledEnum"=w1680) -> ()  [unwired: 2 in, 2 out]
            n763 = property on="Total Number of Patterns" class="NumNb (strict)"("DisabledEnum"=w1680) -> ()  [unwired: 2 in, 2 out]
            n764 = property on="Nstart" class="NumNb (strict)"("DisabledEnum"=w1680) -> ()  [unwired: 2 in, 2 out]
            n765 = property on="Noff" class="NumNb (strict)"("DisabledEnum"=w1680) -> ()  [unwired: 2 in, 2 out]
            n766 = property on="Non" class="NumNb (strict)"("DisabledEnum"=w1680) -> ()  [unwired: 2 in, 2 out]
          }
          frame False {
            w1692 = 2
            w1693 = 2
            w1695 = u32 0
            n767 = local write "Total Number of Patterns"(w1695) -> ()
            n768 = local write "Frames between Patterns"(w1695) -> ()
            n769 = local write "Shoot duration"(0.0) -> ()
            n770 = local write "Shoot at Scan#"(0) -> ()
            n771 = property on="is_single_shoot" class="Bool (strict)"("DisabledEnum"=2) -> ()  [unwired: 2 in, 2 out]
            n772 = property on="Position to add" class="NumNb (strict)"("DisabledEnum"=w1693) -> ()  [unwired: 2 in, 2 out]
            n773 = property on="Shoot at Scan#" class="NumNb (strict)"("DisabledEnum"=w1693) -> ()  [unwired: 2 in, 2 out]
            n774 = property on="Shoot duration" class="NumNb (strict)"("DisabledEnum"=w1693) -> ()  [unwired: 2 in, 2 out]
            n775 = property on="ADD ALL\nPositions" class="Bool (strict)"("DisabledEnum"=w1693) -> ()  [unwired: 2 in, 2 out]
            n776 = property on="RESET POS" class="Bool (strict)"("DisabledEnum"=w1693) -> ()  [unwired: 2 in, 2 out]
            n777 = property on="ADD\nPosition" class="Bool (strict)"("DisabledEnum"=w1693) -> ()  [unwired: 2 in, 2 out]
            n778 = property on="Frames between Patterns" class="NumNb (strict)"("DisabledEnum"=w1692) -> ()  [unwired: 2 in, 2 out]
            n779 = property on="Total Number of Patterns" class="NumNb (strict)"("DisabledEnum"=w1692) -> ()  [unwired: 2 in, 2 out]
            n780 = property on="Nstart" class="NumNb (strict)"("DisabledEnum"=w1692) -> ()  [unwired: 2 in, 2 out]
            n781 = property on="Noff" class="NumNb (strict)"("DisabledEnum"=w1692) -> ()  [unwired: 2 in, 2 out]
            n782 = property on="Non" class="NumNb (strict)"("DisabledEnum"=w1692) -> ()  [unwired: 2 in, 2 out]
          }
        }
      }
      event "useFLUIDICS_TL": Value Change {
        n783 = event-data() -> ("NewVal"=w1696:bool)  [unwired: 1 in, 5 out]
        n784 = case shown="Faux" w1696 {
          frame True {
            w1697 = 0
            n785 = property on="Noff FLUIDICS" class="NumNb (strict)"("DisabledEnum"=w1697) -> ()  [unwired: 2 in, 2 out]
            n786 = property on="Non FLUIDICS" class="NumNb (strict)"("DisabledEnum"=w1697) -> ()  [unwired: 2 in, 2 out]
            n787 = property on="Nstart FLUIDICS" class="NumNb (strict)"("DisabledEnum"=w1697) -> ()  [unwired: 2 in, 2 out]
          }
          frame False {
            w1698 = 2
            n788 = property on="Noff FLUIDICS" class="NumNb (strict)"("DisabledEnum"=w1698) -> ()  [unwired: 2 in, 2 out]
            n789 = property on="Non FLUIDICS" class="NumNb (strict)"("DisabledEnum"=w1698) -> ()  [unwired: 2 in, 2 out]
            n790 = property on="Nstart FLUIDICS" class="NumNb (strict)"("DisabledEnum"=w1698) -> ()  [unwired: 2 in, 2 out]
          }
        }
      }
      event "Exposure Time": Value Change {
        w1699 = 1 items=["Snap", "Sequence"] ("Capture mode")
        # "readout time"
        # "exposure time"
        # "readout speed"
        # "binning"
        # "exposure time"
        n791 = event-data() -> ("NewVal"=w1731:dbl)  [unwired: 1 in, 5 out]
        n792 = call <userlib>:"tm_stopcapture.vi"("error in (no error)"=w1736, "Handle in"=w1737) -> ("error out"=w1735:errorcluster, "Handle out"=w1734:u32)  [unwired: 8 in]
        n793 = call <userlib>:"tm_unpreparecapture.vi"("error in (no error)"=w1735, "Handle in"=w1734) -> ("error out"=w1732:errorcluster, "Handle out"=w1733:u32)  [unwired: 8 in]
        n794 = call <userlib>:"tm_setparameter_a.vi"("error in (no error)"=w1732, "Value in"=w1731, "Parameter"=2049184, "Handle in"=w1733) -> ("error out"=w1729:errorcluster, "Handle out"=w1730:u32)  [unwired: 6 in]
        n795 = call <userlib>:"tm_getparameter_a.vi"("error in (no error)"=w1729, "Parameter"=2049184, "Handle in"=w1730) -> ("error out"=w1722:errorcluster, "Value out"=w1714:dbl, "Handle out"=w1724:u32)  [unwired: 6 in]
        n796 = call <userlib>:"tm_getparameter_a.vi"("error in (no error)"=w1722, "Parameter"=4211872, "Handle in"=w1724) -> ("error out"=w1721:errorcluster, "Value out"=w1711:dbl, "Handle out"=w1723:u32)  [unwired: 6 in]
        n797 = local write "Exposure Time"(w1714) -> ()
        n798 = call <userlib>:"tm_getparameter_a.vi"("error in (no error)"=w1721, "Parameter"=4215968, "Handle in"=w1723) -> ("error out"=w1720:errorcluster, "Value out"=w1712:dbl, "Handle out"=w1719:u32)  [unwired: 6 in]
        n799 = local write "RO Mode"(w1711) -> ()
        n800 = call <userlib>:"tm_getparameter_a.vi"("error in (no error)"=w1720, "Parameter"=4223904, "Handle in"=w1719) -> ("error out"=w1718:errorcluster, "Value out"=w1713:dbl, "Handle out"=w1717:u32)  [unwired: 6 in]
        n801 = local write "Binning"(w1712) -> ()
        n802 = local write "Read Out Time"(w1713) -> ()
        n803 = call <userlib>:"tm_preparecapture.vi"("error in (no error)"=w1718, "Capture mode"=w1699, "Handle in"=w1717) -> ("error out"=w1716:errorcluster, "Buffer Info"=w1709:T2, "Handle out"=w1715:u32)  [unwired: 5 in, 1 out]
        n804 = local write "Buffer Info"(w1709) -> ()
        n805 = call <userlib>:"tm_startcapture_b.vi"("error in (no error)"=w1716, "Handle in"=w1715) -> ("error out"=w1707:errorcluster, "Handle out"=w1708:u32)  [unwired: 8 in]
        n806 = call <userlib>:"tm_firetrigger.vi"("error in (no error)"=w1707, "Handle in"=w1708) -> ("error out"=w1705:errorcluster, "Handle out"=w1706:u32)  [unwired: 8 in]
        n807 = call <userlib>:"tm_waitnextframe.vi"("error in (no error)"=w1705, "Handle in"=w1706) -> ("error out"=w1703:errorcluster, "Handle out"=w1704:u32)  [unwired: 6 in, 2 out]
        n808 = call <userlib>:"tm_getframe_a.vi"("error in (no error)"=w1703, "Buffer Info"=w1709, "Handle in"=w1704) -> ("error out"=w1702:errorcluster, "Data 16"=w1700:u16[][], "Handle out"=w1701:u32)  [unwired: 4 in, 2 out]
        n809 = local write "Intensity Graph"(w1700) -> ()
        n810 = local write "Imtemp"(w1700) -> ()
      }
      event "RO Mode": Value Change {
        w1738 = 1 items=["Snap", "Sequence"] ("Capture mode")
        # "readout speed"
        # "readout time"
        # "exposure time"
        # "readout speed"
        # "binning"
        n811 = event-data() -> ("NewVal"=w1770:u32)  [unwired: 1 in, 5 out]
        n812 = call <userlib>:"tm_stopcapture.vi"("error in (no error)"=w1775, "Handle in"=w1776) -> ("error out"=w1774:errorcluster, "Handle out"=w1773:u32)  [unwired: 8 in]
        n813 = call <userlib>:"tm_unpreparecapture.vi"("error in (no error)"=w1774, "Handle in"=w1773) -> ("error out"=w1771:errorcluster, "Handle out"=w1772:u32)  [unwired: 8 in]
        n814 = call <userlib>:"tm_setparameter_a.vi"("error in (no error)"=w1771, "Value in"=w1770, "Parameter"=4211872, "Handle in"=w1772) -> ("error out"=w1768:errorcluster, "Handle out"=w1769:u32)  [unwired: 6 in]
        n815 = call <userlib>:"tm_getparameter_a.vi"("error in (no error)"=w1768, "Parameter"=2049184, "Handle in"=w1769) -> ("error out"=w1761:errorcluster, "Value out"=w1753:dbl, "Handle out"=w1763:u32)  [unwired: 6 in]
        n816 = call <userlib>:"tm_getparameter_a.vi"("error in (no error)"=w1761, "Parameter"=4211872, "Handle in"=w1763) -> ("error out"=w1760:errorcluster, "Value out"=w1750:dbl, "Handle out"=w1762:u32)  [unwired: 6 in]
        n817 = local write "Exposure Time"(w1753) -> ()
        n818 = call <userlib>:"tm_getparameter_a.vi"("error in (no error)"=w1760, "Parameter"=4215968, "Handle in"=w1762) -> ("error out"=w1759:errorcluster, "Value out"=w1751:dbl, "Handle out"=w1758:u32)  [unwired: 6 in]
        n819 = local write "RO Mode"(w1750) -> ()
        n820 = call <userlib>:"tm_getparameter_a.vi"("error in (no error)"=w1759, "Parameter"=4223904, "Handle in"=w1758) -> ("error out"=w1757:errorcluster, "Value out"=w1752:dbl, "Handle out"=w1756:u32)  [unwired: 6 in]
        n821 = local write "Binning"(w1751) -> ()
        n822 = local write "Read Out Time"(w1752) -> ()
        n823 = call <userlib>:"tm_preparecapture.vi"("error in (no error)"=w1757, "Capture mode"=w1738, "Handle in"=w1756) -> ("error out"=w1755:errorcluster, "Buffer Info"=w1742:T2, "Handle out"=w1754:u32)  [unwired: 5 in, 1 out]
        n824 = local write "Buffer Info"(w1742) -> ()
        n825 = call <userlib>:"tm_startcapture_b.vi"("error in (no error)"=w1755, "Handle in"=w1754) -> ("error out"=w1747:errorcluster, "Handle out"=w1748:u32)  [unwired: 8 in]
        n826 = call <userlib>:"tm_firetrigger.vi"("error in (no error)"=w1747, "Handle in"=w1748) -> ("error out"=w1745:errorcluster, "Handle out"=w1746:u32)  [unwired: 8 in]
        n827 = call <userlib>:"tm_waitnextframe.vi"("error in (no error)"=w1745, "Handle in"=w1746) -> ("error out"=w1744:errorcluster, "Handle out"=w1743:u32)  [unwired: 6 in, 2 out]
        n828 = call <userlib>:"tm_getframe_a.vi"("error in (no error)"=w1744, "Buffer Info"=w1742, "Handle in"=w1743) -> ("error out"=w1740:errorcluster, "Data 16"=w1739:u16[][], "Handle out"=w1741:u32)  [unwired: 4 in, 2 out]
        n829 = local write "Intensity Graph"(w1739) -> ()
        n830 = local write "Imtemp"(w1739) -> ()
      }
      event "Binning": Value Change {
        w1777 = 1 items=["Snap", "Sequence"] ("Capture mode")
        # "binning"
        # "readout time"
        # "exposure time"
        # "readout speed"
        # "binning"
        n831 = event-data() -> ("NewVal"=w1809:u16)  [unwired: 1 in, 5 out]
        n832 = call <userlib>:"tm_stopcapture.vi"("error in (no error)"=w1814, "Handle in"=w1815) -> ("error out"=w1813:errorcluster, "Handle out"=w1812:u32)  [unwired: 8 in]
        n833 = call <userlib>:"tm_unpreparecapture.vi"("error in (no error)"=w1813, "Handle in"=w1812) -> ("error out"=w1810:errorcluster, "Handle out"=w1811:u32)  [unwired: 8 in]
        n834 = call <userlib>:"tm_setparameter_a.vi"("error in (no error)"=w1810, "Value in"=w1809, "Parameter"=4215968, "Handle in"=w1811) -> ("error out"=w1807:errorcluster, "Handle out"=w1808:u32)  [unwired: 6 in]
        n835 = call <userlib>:"tm_getparameter_a.vi"("error in (no error)"=w1807, "Parameter"=2049184, "Handle in"=w1808) -> ("error out"=w1800:errorcluster, "Value out"=w1792:dbl, "Handle out"=w1802:u32)  [unwired: 6 in]
        n836 = call <userlib>:"tm_getparameter_a.vi"("error in (no error)"=w1800, "Parameter"=4211872, "Handle in"=w1802) -> ("error out"=w1799:errorcluster, "Value out"=w1789:dbl, "Handle out"=w1801:u32)  [unwired: 6 in]
        n837 = local write "Exposure Time"(w1792) -> ()
        n838 = call <userlib>:"tm_getparameter_a.vi"("error in (no error)"=w1799, "Parameter"=4215968, "Handle in"=w1801) -> ("error out"=w1798:errorcluster, "Value out"=w1790:dbl, "Handle out"=w1797:u32)  [unwired: 6 in]
        n839 = local write "RO Mode"(w1789) -> ()
        n840 = call <userlib>:"tm_getparameter_a.vi"("error in (no error)"=w1798, "Parameter"=4223904, "Handle in"=w1797) -> ("error out"=w1796:errorcluster, "Value out"=w1791:dbl, "Handle out"=w1795:u32)  [unwired: 6 in]
        n841 = local write "Binning"(w1790) -> ()
        n842 = local write "Read Out Time"(w1791) -> ()
        n843 = call <userlib>:"tm_preparecapture.vi"("error in (no error)"=w1796, "Capture mode"=w1777, "Handle in"=w1795) -> ("error out"=w1794:errorcluster, "Buffer Info"=w1781:T2, "Handle out"=w1793:u32)  [unwired: 5 in, 1 out]
        n844 = local write "Buffer Info"(w1781) -> ()
        n845 = call <userlib>:"tm_startcapture_b.vi"("error in (no error)"=w1794, "Handle in"=w1793) -> ("error out"=w1786:errorcluster, "Handle out"=w1787:u32)  [unwired: 8 in]
        n846 = call <userlib>:"tm_firetrigger.vi"("error in (no error)"=w1786, "Handle in"=w1787) -> ("error out"=w1784:errorcluster, "Handle out"=w1785:u32)  [unwired: 8 in]
        n847 = call <userlib>:"tm_waitnextframe.vi"("error in (no error)"=w1784, "Handle in"=w1785) -> ("error out"=w1782:errorcluster, "Handle out"=w1783:u32)  [unwired: 6 in, 2 out]
        n848 = call <userlib>:"tm_getframe_a.vi"("error in (no error)"=w1782, "Buffer Info"=w1781, "Handle in"=w1783) -> ("error out"=w1778:errorcluster, "Data 16"=w1780:u16[][], "Handle out"=w1779:u32)  [unwired: 4 in, 2 out]
        n849 = local write "Intensity Graph"(w1780) -> ()
        n850 = local write "Imtemp"(w1780) -> ()
      }
      event "Loadpositions": Value Change {
        n851 = event-data() -> ("NewVal"=w1816:bool)  [unwired: 1 in, 5 out]
        n852 = case shown="Vrai" w1816 {
          frame False {
          }
          frame True {
            n853 = stacked-sequence {
              frame #0 {
                n854 = local read "XY positions path"() -> (w1819:path)
                n855 = call "loadXYpositions_svi.vi"("Chemin en entrée"=w1819) -> ("final XY"=w1818:T1, "Number of lines"=w1817:u32)  [unwired: 9 in]
                n856 = local write "stored XY"(w1818) -> ()
                n857 = local write "TL_NPOS"(w1817) -> ()
              }
              frame #1 {
                n858 = local write "Loadpositions"(FALSE) -> ()
              }
            }
          }
        }
      }
      event "Generate\nPositions": Value Change {
        n859 = event-data() -> ("NewVal"=w1821:bool)  [unwired: 1 in, 5 out]
        n860 = case shown="Vrai" w1821 {
          frame False {
          }
          frame True {
            n861 = stacked-sequence {
              frame #0 {
                n862 = local read "Microscope Objective\nMagnification"() -> (w1825:dbl)
                n863 = local read "Number\nof\nPositions"() -> (w1824:u32)
                n864 = local read "Spacing X (µm)"() -> (w1828:dbl)
                n865 = local read "Spacing Y (µm)"() -> (w1827:dbl)
                n866 = local read "Method"() -> (w1826:u8)
                n867 = call "geneXY_svi.vi"("Spacing Y (µm)"=w1827, "Number of Positions"=w1824, "Spacing X (µm)"=w1828, "Method"=w1826, "Microscope Objective\nMagnification"=w1825) -> ("Real Matrix"=w1822:T1, "field_size(µm)"=w1823:dbl)  [unwired: 5 in]
                n868 = local write "stored XY"(w1822) -> ()
                n869 = local write "Field\nHeigth (µm)"(w1823) -> ()
                n870 = local write "Field\nWidth (µm)"(w1823) -> ()
                n871 = stacked-sequence {
                  tunnel: w1823 -> [w1830 w1834]
                  tunnel: w1822 -> [w1829 w1835]
                  frame #0 {
                    n872 = call "vizuXY_svi.vi"("LY (mm)"=w1830, "LX (mm)"=w1830, "stored XY (µm)"=w1829) -> ("Tableau"=w1831:T4)  [unwired: 8 in]
                    n873 = local write "Scanning Motif"(w1831) -> ()
                  }
                  frame #1 {
                    n874 = call "maximini_XYlist_svi.vi"("stored XY"=w1835, "LY"=w1834, "LX"=w1834) -> ("mini (µm)"=w1832:dbl, "maxi (µm)"=w1833:dbl)  [unwired: 7 in]
                    n875 = property on="Scanning Motif" class="GraphXY (strict)"("XScale.Minimum"=w1832, "XScale.Maximum"=w1833, "YScale.Minimum"=w1832, "YScale.Maximum"=w1833) -> ()  [unwired: 2 in, 2 out]
                  }
                }
              }
              frame #1 {
                n876 = local write "Generate\nPositions"(FALSE) -> ()
              }
            }
          }
        }
      }
      event "ADD\nChanel": Value Change {
        n877 = event-data() -> ("NewVal"=w1837:bool)  [unwired: 1 in, 5 out]
        n878 = case shown="Vrai" w1837 {
          frame False {
          }
          frame True {
            n879 = stacked-sequence {
              frame #0 {
                n880 = local read "LED-10"() -> (w1849:bool)
                n881 = local read "LED-11"() -> (w1850:bool)
                n882 = local read "LED-0"() -> (w1857:bool)
                n883 = local read "LED-1"() -> (w1856:bool)
                n884 = local read "LED-2"() -> (w1855:bool)
                n885 = local read "LED-3"() -> (w1854:bool)
                n886 = local read "LED-4"() -> (w1853:bool)
                n887 = local read "LED-5"() -> (w1852:bool)
                n888 = local read "LED-6"() -> (w1851:bool)
                n889 = local read "LED-7"() -> (w1846:bool)
                n890 = local read "LED-8"() -> (w1847:bool)
                n891 = local read "LED-9"() -> (w1848:bool)
                n892 = Build Array(w1857, w1856, w1855, w1854, w1853, w1852, w1851, w1846, w1847, w1848, w1849, w1850) -> (w1844:bool[])
                n893 = local read "Filter selection"() -> (w1841:u8)
                n894 = local read "used Filters"() -> (w1842:u8[])
                n895 = local read "used LEDs"() -> (w1845:bool[][])
                n896 = Build Array (concatenate)(w1845, w1844) -> (w1843:bool[][])
                n897 = Build Array (concatenate)(w1842, w1841) -> (w1840:u8[])
                n898 = local write "used LEDs"(w1843) -> ()
                n899 = Array Size(array=w1840) -> (size(s)=w1839:i32)
                n900 = local write "used Filters"(w1840) -> ()
                n901 = To Unsigned Byte Integer(number=w1839) -> (unsigned 8bit integer=w1838:u8)
                n902 = local write "TL_NCAN"(w1838) -> ()
              }
              frame #1 {
                w1858 = FALSE
                n903 = local write "ADD\nChanel"(w1858) -> ()
                n904 = local write "Filter selection"(1) -> ()
                n905 = local write "LED-10"(w1858) -> ()
                n906 = local write "LED-11"(w1858) -> ()
                n907 = local write "LED-0"(w1858) -> ()
                n908 = local write "LED-1"(w1858) -> ()
                n909 = local write "LED-2"(w1858) -> ()
                n910 = local write "LED-3"(w1858) -> ()
                n911 = local write "LED-4"(w1858) -> ()
                n912 = local write "LED-5"(w1858) -> ()
                n913 = local write "LED-6"(w1858) -> ()
                n914 = local write "LED-7"(w1858) -> ()
                n915 = local write "LED-8"(w1858) -> ()
                n916 = local write "LED-9"(w1858) -> ()
              }
            }
          }
        }
      }
      event "ADD\nPosition": Value Change {
        n917 = event-data() -> ("NewVal"=w1860:bool)  [unwired: 1 in, 5 out]
        n918 = case shown="Vrai" w1860 {
          frame False {
          }
          frame True {
            n919 = local read "TL_NPOS"() -> (w1862:u32)
            n920 = local read "Position to add"() -> (w1863:u32)
            n921 = Less Or Equal?(x=w1863, y=w1862) -> (x <= y?=w1861:bool)
            n922 = case shown="Vrai" w1861 {
              tunnel: w1863 -> [_ w1864]
              frame False {
              }
              frame True {
                n923 = local read "shooted_ positions"() -> (w1871:bool[][])
                n924 = local read "shoot_list"() -> (w1868:T1)
                n925 = Replace Array Subset(array=w1871, new element=TRUE, index (row)=w1864, index (col)=0) -> (w1869:bool[][])
                n926 = Build Array(w1864) -> (w1867:T1)
                n927 = local write "shooted_ positions"(w1869) -> ()
                n928 = local write "ADD\nPosition"(FALSE) -> ()
                n929 = Build Array (concatenate)(w1868, w1867) -> (w1866:T1)
                n930 = local write "shoot_list"(w1866) -> ()
              }
            }
          }
        }
      }
      event "ADD ALL\nPositions": Value Change {
        n931 = event-data() -> ("NewVal"=w1873:bool)  [unwired: 1 in, 5 out]
        n932 = case shown="Vrai" w1873 {
          frame False {
          }
          frame True {
            n933 = local read "TL_NPOS"() -> (w1875:u32)
            n934 = for {
              N: w1875 -> [_]
              i -> [w1876]
              n935 = local read "shooted_ positions"() -> (w1882:bool[][])
              n936 = local read "shoot_list"() -> (w1879:T1)
              n937 = Replace Array Subset(array=w1882, new element=TRUE, index (row)=w1876, index (col)=0) -> (w1880:bool[][])
              n938 = Build Array(w1876) -> (w1878:T1)
              n939 = local write "shooted_ positions"(w1880) -> ()
              n940 = Build Array (concatenate)(w1879, w1878) -> (w1877:T1)
              n941 = local write "shoot_list"(w1877) -> ()
            }
            n942 = local write "ADD ALL\nPositions"(FALSE) -> ()
          }
        }
      }
      event "RESET ALL\nChanels": Value Change {
        n943 = event-data() -> ("NewVal"=w1884:bool)  [unwired: 1 in, 5 out]
        n944 = case shown="Vrai" w1884 {
          frame False {
          }
          frame True {
            w1887 = FALSE
            n945 = Initialize Array(FALSE, 0, 0) -> (w1890:bool[][])
            n946 = Initialize Array(u8 0, 0) -> (w1889:u8[])
            n947 = local write "used Filters"(w1889) -> ()
            n948 = local write "TL_NCAN"(u8 0) -> ()
            n949 = local write "used LEDs"(w1890) -> ()
            n950 = local write "RESET ALL\nChanels"(FALSE) -> ()
            n951 = local write "Filter selection"(1) -> ()
            n952 = local write "LED-0"(w1887) -> ()
            n953 = local write "LED-1"(w1887) -> ()
            n954 = local write "LED-2"(w1887) -> ()
            n955 = local write "LED-3"(w1887) -> ()
            n956 = local write "LED-4"(w1887) -> ()
            n957 = local write "LED-5"(w1887) -> ()
            n958 = local write "LED-6"(w1887) -> ()
            n959 = local write "LED-7"(w1887) -> ()
            n960 = local write "LED-8"(w1887) -> ()
            n961 = local write "LED-9"(w1887) -> ()
            n962 = local write "LED-10"(w1887) -> ()
            n963 = local write "LED-11"(w1887) -> ()
          }
        }
      }
      event "RESET POS": Value Change {
        n964 = event-data() -> ("NewVal"=w1896:bool)  [unwired: 1 in, 5 out]
        n965 = case shown="Vrai" w1896 {
          frame False {
          }
          frame True {
            n966 = Initialize Array(TRUE, 1, 0) -> (w1899:bool[][])
            n967 = Build Array(0) -> (w1898:T1)
            n968 = local write "shooted_ positions"(w1899) -> ()
            n969 = local write "shoot_list"(w1898) -> ()
            n970 = local write "RESET POS"(FALSE) -> ()
          }
        }
      }
      event "Load Config": Value Change {
        n971 = event-data() -> ("NewVal"=w1905:bool)  [unwired: 1 in, 5 out]
        n972 = case shown="Vrai" w1905 {
          tunnel: w1912 -> [w1919 w2031]
          tunnel: w1911 -> [w1918 w2030]
          tunnel: w1910 -> [w1917 w2032]
          tunnel: [w1916 w2029] -> w1909
          tunnel: [w1915 w2032] -> w1908
          tunnel: [w1914 w2031] -> w1907
          tunnel: [w1913 w2030] -> w1906
          tunnel: w1904 -> [_ w2029]
          frame True {
            n973 = stacked-sequence {
              seq-local: [w1923 _ _ _] -> [_ w1948 _ _]
              tunnel: w1919 -> [_ w2001 _ _]
              tunnel: w1918 -> [_ w2000 _ _]
              tunnel: w1917 -> [_ w1970 _ _]
              tunnel: [_ w1969 _ _] -> w1916
              tunnel: [_ w1968 _ _] -> w1915
              tunnel: [_ w1957 _ _] -> w1914
              tunnel: [_ w1956 _ _] -> w1913
              frame #0 {
                n974 = String To Path(string="D:\\CONFIGS_TIME_LAPSE") -> (path=w1920:path)
                n975 = call "Boîte de dialogue de fichier"("start path"=w1920, "prompt"="Please select your favorite config...") -> ("selected path"=w1923:path)  [unwired: 10 in, 3 out]
              }
              frame #1 {
                w1988 = 4211872
                w1987 = 4215968
                w1983 = 1 items=["Snap", "Sequence"] ("Capture mode")
                w1989 = 2049184
                # "readout time"
                # "readout speed"
                # "binning"
                # "exposure time"
                n976 = call "load_config_v4_svi.vi"("Config Directory"=w1948) -> ("BETWEEN_PAT"=w1937:u32, "NPAT"=w1936:u32, "shoot_DURATION"=w1935:dbl, "shoot_at_SCAN"=w1934:u32, "is_single_shoot"=w1933:bool, "useLASER"=w1932:bool, "MIN_SCAN_DUR"=w1929:dbl, "Noff_fluidics"=w1944:u32, "BETEWEEN_SCAN"=w1931:u32, "USED_FILTERS 2"=w1945:u8[], "Nstart_laser"=w1938:u32, "USED_LEDS 2"=w1946:bool[][], "NSCAN"=w1930:u32, "EXPT"=w1924:dbl, "Non_laser"=w1939:u32, "Non_fluidics"=w1943:u32, "XYPOS"=w1947:T1, "Refnum VISA en sortie"=w1927:refnum<visa-resource-name>, "BIN"=w1926:u16, "Nstart_fluidics"=w1942:u32, "ROMODE"=w1925:u32, "useFLUIDICS"=w1941:bool, "STAGE_SPEED"=w1928:dbl, "Noff_laser"=w1940:u32)  [unwired: 3 in]
                n977 = call <userlib>:"tm_stopcapture.vi"("error in (no error)"=w2000, "Handle in"=w2001) -> ("error out"=w1999:errorcluster, "Handle out"=w1998:u32)  [unwired: 8 in]
                n978 = local write "Stage COM PORT"(w1927) -> ()
                n979 = local write "stage speed (mm/s)"(w1928) -> ()
                n980 = local write "stored XY"(w1947) -> ()
                n981 = local write "Total Number of Patterns"(w1936) -> ()
                n982 = local write "Frames between Patterns"(w1937) -> ()
                n983 = local write "Shoot duration"(w1935) -> ()
                n984 = local write "Nstart"(w1938) -> ()
                n985 = local write "Non"(w1939) -> ()
                n986 = local write "useLASER_TL"(w1932) -> ()
                n987 = local write "used Filters"(w1945) -> ()
                n988 = local write "is_single_shoot"(w1933) -> ()
                n989 = local write "Shoot at Scan#"(w1934) -> ()
                n990 = local write "Noff"(w1940) -> ()
                n991 = call <userlib>:"tm_unpreparecapture.vi"("error in (no error)"=w1999, "Handle in"=w1998) -> ("error out"=w1997:errorcluster, "Handle out"=w1996:u32)  [unwired: 8 in]
                n992 = local write "Total Number of Scan"(w1930) -> ()
                n993 = local write "used LEDs"(w1946) -> ()
                n994 = local write "Exposure Time"(w1924) -> ()
                n995 = local write "RO Mode"(w1925) -> ()
                n996 = local write "Binning"(w1926) -> ()
                n997 = local write "Min. Scan duration"(w1929) -> ()
                n998 = local write "Frames between Scan"(w1931) -> ()
                n999 = local write "useFLUIDICS_TL"(w1941) -> ()
                n1000 = local write "Non FLUIDICS"(w1943) -> ()
                n1001 = local write "Nstart FLUIDICS"(w1942) -> ()
                n1002 = local write "Noff FLUIDICS"(w1944) -> ()
                n1003 = call <userlib>:"tm_setparameter_a.vi"("error in (no error)"=w1997, "Value in"=w1924, "Parameter"=w1989, "Handle in"=w1996) -> ("error out"=w1994:errorcluster, "Handle out"=w1995:u32)  [unwired: 6 in]
                n1004 = call <userlib>:"tm_setparameter_a.vi"("error in (no error)"=w1994, "Value in"=w1925, "Parameter"=w1988, "Handle in"=w1995) -> ("error out"=w1992:errorcluster, "Handle out"=w1993:u32)  [unwired: 6 in]
                n1005 = call <userlib>:"tm_setparameter_a.vi"("error in (no error)"=w1992, "Value in"=w1926, "Parameter"=w1987, "Handle in"=w1993) -> ("error out"=w1990:errorcluster, "Handle out"=w1991:u32)  [unwired: 6 in]
                n1006 = flat-sequence {
                  tunnel: w1970 -> [w2013]
                  tunnel: w1927 -> [w2011]
                  tunnel: w1928 -> [w2012]
                  tunnel: [w2011] -> w1969
                  tunnel: [w2010] -> w2002
                  tunnel: [w2016] -> _
                  tunnel: [w2014] -> w1968
                  tunnel: w2002 -> [w2014]
                  frame #0 {
                    n1007 = call "svi_mysetSpeedXY.vi"("entrée d'erreur (pas d'erreur)"=w2013, "speed (mm/s)"=w2012, "Refnum VISA en entrée"=w2011) -> ("sortie d'erreur"=w2010:errorcluster)  [unwired: 8 in]
                  }
                  frame #1 {
                    n1008 = Wait (ms)(milliseconds to wait=1000) -> (millisecond timer value=w2016:u32)
                  }
                }
                n1009 = Array Size(array=w1945) -> (size(s)=w1967:i32)
                n1010 = Matrix Size(0:w1947) -> (1:w1965:i32)  [unwired: 1 out]
                n1011 = To Unsigned Byte Integer(number=w1967) -> (unsigned 8bit integer=w1966:u8)
                n1012 = To Unsigned Long Integer(number=w1965) -> (unsigned 32bit integer=w1964:u32)
                n1013 = call <userlib>:"tm_getparameter_a.vi"("error in (no error)"=w1990, "Parameter"=w1989, "Handle in"=w1991) -> ("error out"=w1979:errorcluster, "Value out"=w1974:dbl, "Handle out"=w1980:u32)  [unwired: 6 in]
                n1014 = call <userlib>:"tm_getparameter_a.vi"("error in (no error)"=w1979, "Parameter"=w1988, "Handle in"=w1980) -> ("error out"=w1978:errorcluster, "Value out"=w1973:dbl, "Handle out"=w1977:u32)  [unwired: 6 in]
                n1015 = local read "Microscope Objective\nMagnification"() -> (w1950:dbl)
                n1016 = local write "TL_NCAN"(w1966) -> ()
                n1017 = local write "TL_NPOS"(w1964) -> ()
                n1018 = local write "Exposure Time"(w1974) -> ()
                n1019 = call <userlib>:"tm_getparameter_a.vi"("error in (no error)"=w1978, "Parameter"=w1987, "Handle in"=w1977) -> ("error out"=w1975:errorcluster, "Value out"=w1972:dbl, "Handle out"=w1976:u32)  [unwired: 6 in]
                n1020 = local write "RO Mode"(w1973) -> ()
                n1021 = local write "Binning"(w1972) -> ()
                n1022 = call <userlib>:"tm_getparameter_a.vi"("error in (no error)"=w1975, "Parameter"=4223904, "Handle in"=w1976) -> ("error out"=w1984:errorcluster, "Value out"=w1971:dbl, "Handle out"=w1985:u32)  [unwired: 6 in]
                n1023 = local write "Read Out Time"(w1971) -> ()
                n1024 = Multiply(x=2048.0, y=6.5) -> (x*y=w1951:dbl)
                n1025 = Divide(x=w1951, y=w1950) -> (x/y=w1949:dbl)
                n1026 = stacked-sequence {
                  tunnel: w1947 -> [w2005 w2006]
                  tunnel: w1949 -> [w2004 w2007]
                  frame #0 {
                    n1027 = call "vizuXY_svi.vi"("LY (mm)"=w2004, "LX (mm)"=w2004, "stored XY (µm)"=w2005) -> ("Tableau"=w2003:T4)  [unwired: 8 in]
                    n1028 = local write "Scanning Motif"(w2003) -> ()
                  }
                  frame #1 {
                    n1029 = call "maximini_XYlist_svi.vi"("stored XY"=w2006, "LY"=w2007, "LX"=w2007) -> ("mini (µm)"=w2008:dbl, "maxi (µm)"=w2009:dbl)  [unwired: 7 in]
                    n1030 = property on="Scanning Motif" class="GraphXY (strict)"("XScale.Maximum"=w2009, "XScale.Minimum"=w2008, "YScale.Maximum"=w2009, "YScale.Minimum"=w2008) -> ()  [unwired: 2 in, 2 out]
                  }
                }
                n1031 = call <userlib>:"tm_preparecapture.vi"("error in (no error)"=w1984, "Capture mode"=w1983, "Handle in"=w1985) -> ("error out"=w1981:errorcluster, "Buffer Info"=w1954:T2, "Handle out"=w1982:u32)  [unwired: 5 in, 1 out]
                n1032 = local write "Buffer Info"(w1954) -> ()
                n1033 = call <userlib>:"tm_startcapture_b.vi"("error in (no error)"=w1981, "Handle in"=w1982) -> ("error out"=w1962:errorcluster, "Handle out"=w1963:u32)  [unwired: 8 in]
                n1034 = call <userlib>:"tm_firetrigger.vi"("error in (no error)"=w1962, "Handle in"=w1963) -> ("error out"=w1960:errorcluster, "Handle out"=w1961:u32)  [unwired: 8 in]
                n1035 = call <userlib>:"tm_waitnextframe.vi"("error in (no error)"=w1960, "Handle in"=w1961) -> ("error out"=w1958:errorcluster, "Handle out"=w1959:u32)  [unwired: 6 in, 2 out]
                n1036 = call <userlib>:"tm_getframe_a.vi"("error in (no error)"=w1958, "Buffer Info"=w1954, "Handle in"=w1959) -> ("error out"=w1956:errorcluster, "Data 16"=w1955:u16[][], "Handle out"=w1957:u32)  [unwired: 4 in, 2 out]
                n1037 = local write "Intensity Graph"(w1955) -> ()
                n1038 = local write "Imtemp"(w1955) -> ()
              }
              frame #2 {
                n1039 = local read "useLASER_TL"() -> (w2018:bool)
                n1040 = case shown="Vrai" w2018 {
                  frame True {
                    n1041 = local read "is_single_shoot"() -> (w2021:bool)
                    n1042 = case shown="Vrai" w2021 {
                      frame True {
                        w2022 = 2
                        w2023 = 0
                        n1043 = property on="RESET POS" class="Bool (strict)"("DisabledEnum"=w2023) -> ()  [unwired: 2 in, 2 out]
                        n1044 = property on="ADD\nPosition" class="Bool (strict)"("DisabledEnum"=w2023) -> ()  [unwired: 2 in, 2 out]
                        n1045 = property on="ADD ALL\nPositions" class="Bool (strict)"("DisabledEnum"=w2023) -> ()  [unwired: 2 in, 2 out]
                        n1046 = property on="Shoot at Scan#" class="NumNb (strict)"("DisabledEnum"=w2023) -> ()  [unwired: 2 in, 2 out]
                        n1047 = property on="Position to add" class="NumNb (strict)"("DisabledEnum"=w2023) -> ()  [unwired: 2 in, 2 out]
                        n1048 = property on="Shoot duration" class="NumNb (strict)"("DisabledEnum"=w2023) -> ()  [unwired: 2 in, 2 out]
                        n1049 = property on="is_single_shoot" class="Bool (strict)"("DisabledEnum"=w2023) -> ()  [unwired: 2 in, 2 out]
                        n1050 = property on="Noff" class="NumNb (strict)"("DisabledEnum"=w2022) -> ()  [unwired: 2 in, 2 out]
                        n1051 = property on="Total Number of Patterns" class="NumNb (strict)"("DisabledEnum"=w2022) -> ()  [unwired: 2 in, 2 out]
                        n1052 = property on="Nstart" class="NumNb (strict)"("DisabledEnum"=w2022) -> ()  [unwired: 2 in, 2 out]
                        n1053 = property on="Frames between Patterns" class="NumNb (strict)"("DisabledEnum"=w2022) -> ()  [unwired: 2 in, 2 out]
                        n1054 = property on="Non" class="NumNb (strict)"("DisabledEnum"=w2022) -> ()  [unwired: 2 in, 2 out]
                      }
                      frame False {
                        w2024 = 0
                        w2025 = 2
                        n1055 = property on="RESET POS" class="Bool (strict)"("DisabledEnum"=w2025) -> ()  [unwired: 2 in, 2 out]
                        n1056 = property on="ADD\nPosition" class="Bool (strict)"("DisabledEnum"=w2025) -> ()  [unwired: 2 in, 2 out]
                        n1057 = property on="ADD ALL\nPositions" class="Bool (strict)"("DisabledEnum"=w2025) -> ()  [unwired: 2 in, 2 out]
                        n1058 = property on="Shoot at Scan#" class="NumNb (strict)"("DisabledEnum"=w2025) -> ()  [unwired: 2 in, 2 out]
                        n1059 = property on="Position to add" class="NumNb (strict)"("DisabledEnum"=w2025) -> ()  [unwired: 2 in, 2 out]
                        n1060 = property on="Shoot duration" class="NumNb (strict)"("DisabledEnum"=w2025) -> ()  [unwired: 2 in, 2 out]
                        n1061 = property on="is_single_shoot" class="Bool (strict)"("DisabledEnum"=w2025) -> ()  [unwired: 2 in, 2 out]
                        n1062 = property on="Noff" class="NumNb (strict)"("DisabledEnum"=w2024) -> ()  [unwired: 2 in, 2 out]
                        n1063 = property on="Total Number of Patterns" class="NumNb (strict)"("DisabledEnum"=w2024) -> ()  [unwired: 2 in, 2 out]
                        n1064 = property on="Nstart" class="NumNb (strict)"("DisabledEnum"=w2024) -> ()  [unwired: 2 in, 2 out]
                        n1065 = property on="Frames between Patterns" class="NumNb (strict)"("DisabledEnum"=w2024) -> ()  [unwired: 2 in, 2 out]
                        n1066 = property on="Non" class="NumNb (strict)"("DisabledEnum"=w2024) -> ()  [unwired: 2 in, 2 out]
                      }
                    }
                  }
                  frame False {
                    w2026 = 2
                    w2027 = 2
                    n1067 = property on="RESET POS" class="Bool (strict)"("DisabledEnum"=w2027) -> ()  [unwired: 2 in, 2 out]
                    n1068 = property on="ADD\nPosition" class="Bool (strict)"("DisabledEnum"=w2027) -> ()  [unwired: 2 in, 2 out]
                    n1069 = property on="ADD ALL\nPositions" class="Bool (strict)"("DisabledEnum"=w2027) -> ()  [unwired: 2 in, 2 out]
                    n1070 = property on="Shoot at Scan#" class="NumNb (strict)"("DisabledEnum"=w2027) -> ()  [unwired: 2 in, 2 out]
                    n1071 = property on="Position to add" class="NumNb (strict)"("DisabledEnum"=w2027) -> ()  [unwired: 2 in, 2 out]
                    n1072 = property on="Shoot duration" class="NumNb (strict)"("DisabledEnum"=w2027) -> ()  [unwired: 2 in, 2 out]
                    n1073 = property on="is_single_shoot" class="Bool (strict)"("DisabledEnum"=w2027) -> ()  [unwired: 2 in, 2 out]
                    n1074 = property on="Noff" class="NumNb (strict)"("DisabledEnum"=w2026) -> ()  [unwired: 2 in, 2 out]
                    n1075 = property on="Total Number of Patterns" class="NumNb (strict)"("DisabledEnum"=w2026) -> ()  [unwired: 2 in, 2 out]
                    n1076 = property on="Nstart" class="NumNb (strict)"("DisabledEnum"=w2026) -> ()  [unwired: 2 in, 2 out]
                    n1077 = property on="Frames between Patterns" class="NumNb (strict)"("DisabledEnum"=w2026) -> ()  [unwired: 2 in, 2 out]
                    n1078 = property on="Non" class="NumNb (strict)"("DisabledEnum"=w2026) -> ()  [unwired: 2 in, 2 out]
                  }
                }
                n1079 = local read "useFLUIDICS_TL"() -> (w2017:bool)
                n1080 = case shown="Vrai" w2017 {
                  frame True {
                    w2019 = 0
                    n1081 = property on="Non FLUIDICS" class="NumNb (strict)"("DisabledEnum"=w2019) -> ()  [unwired: 2 in, 2 out]
                    n1082 = property on="Noff FLUIDICS" class="NumNb (strict)"("DisabledEnum"=w2019) -> ()  [unwired: 2 in, 2 out]
                    n1083 = property on="Nstart FLUIDICS" class="NumNb (strict)"("DisabledEnum"=w2019) -> ()  [unwired: 2 in, 2 out]
                  }
                  frame False {
                    w2020 = 2
                    n1084 = property on="Non FLUIDICS" class="NumNb (strict)"("DisabledEnum"=w2020) -> ()  [unwired: 2 in, 2 out]
                    n1085 = property on="Noff FLUIDICS" class="NumNb (strict)"("DisabledEnum"=w2020) -> ()  [unwired: 2 in, 2 out]
                    n1086 = property on="Nstart FLUIDICS" class="NumNb (strict)"("DisabledEnum"=w2020) -> ()  [unwired: 2 in, 2 out]
                  }
                }
              }
              frame #3 {
                n1087 = local write "Load Config"(FALSE) -> ()
              }
            }
          }
          frame False {
          }
        }
      }
      event "Save Config": Value Change {
        n1088 = event-data() -> ("NewVal"=w2033:bool)  [unwired: 1 in, 5 out]
        n1089 = case shown="Vrai" w2033 {
          frame False {
          }
          frame True {
            n1090 = stacked-sequence {
              frame #0 {
                n1091 = local read "Camera Model"() -> (w2067:string)
                n1092 = local read "Camera Serial"() -> (w2062:string)
                n1093 = local read "Version"() -> (w2066:string)
                n1094 = local read "Total Number of Patterns"() -> (w2038:u32)
                n1095 = local read "Frames between Patterns"() -> (w2037:u32)
                n1096 = local read "Total Number of Scan"() -> (w2045:u32)
                n1097 = local read "Frames between Scan"() -> (w2044:u32)
                n1098 = local read "stage speed (mm/s)"() -> (w2054:sgl)
                n1099 = local read "Min. Scan duration"() -> (w2043:dbl)
                n1100 = local read "Stage COM PORT"() -> (w2053:refnum<visa-resource-name>)
                n1101 = local read "Config Directory"() -> (w2069:path)
                n1102 = local read "Nstart FLUIDICS"() -> (w2047:u32)
                n1103 = local read "config Name"() -> (w2058:string)
                n1104 = local read "Noff FLUIDICS"() -> (w2049:u32)
                n1105 = local read "useFLUIDICS_TL"() -> (w2046:bool)
                n1106 = local read "Non FLUIDICS"() -> (w2048:u32)
                n1107 = local read "Shoot at Scan#"() -> (w2040:i32)
                n1108 = local read "Shoot duration"() -> (w2039:dbl)
                n1109 = local read "is_single_shoot"() -> (w2041:bool)
                n1110 = local read "softversion"() -> (w2059:string)
                n1111 = local read "useLASER_TL"() -> (w2042:bool)
                n1112 = local read "Nstart"() -> (w2036:u32)
                n1113 = local read "used Filters"() -> (w2050:u8[])
                n1114 = local read "used LEDs"() -> (w2051:bool[][])
                n1115 = local read "stored XY"() -> (w2052:T1)
                n1116 = local read "Exposure Time"() -> (w2057:dbl)
                n1117 = local read "Non"() -> (w2035:u32)
                n1118 = local read "Noff"() -> (w2034:u32)
                n1119 = local read "RO Mode"() -> (w2055:u32)
                n1120 = local read "Binning"() -> (w2056:u16)
                n1121 = Concatenate Strings("camera model :", w2067, "\r", "camera version :", w2066, "\r", w2062, "\r") -> (w2060:string)
                n1122 = call "save_config_v4_svi.vi"("Refnum VISA en entrée"=w2053, "Camera infos"=w2060, "Config Directory"=w2069, "USED_LEDS"=w2051, "STAGE_SPEED"=w2054, "Non_fluidics"=w2048, "XYPOS"=w2052, "Nstart_fluidics"=w2047, "ROMODE"=w2055, "NSCAN"=w2045, "BIN"=w2056, "USED_FILTERS"=w2050, "EXPT"=w2057, "BETWEEN_SCAN"=w2044, "config Name"=w2058, "useFLUIDICS"=w2046, "SOFT_VERSION"=w2059, "MIN. SCAN duration"=w2043, "Noff_fluidics"=w2049, "BETWEEN_PAT"=w2037, "NPAT"=w2038, "Noff_laser"=w2034, "Non_laser"=w2035, "Nstart_laser"=w2036, "SHOOT duration"=w2039, "shoot_at_SCAN"=w2040, "isSINGLEshoot"=w2041, "useLASER"=w2042) -> ()
              }
              frame #1 {
                n1123 = local write "Save Config"(FALSE) -> ()
              }
            }
          }
        }
      }
    }
  }
  n1124 = Build Array(0) -> (→"shoot_list":T1)
  n1125 = Initialize Array(TRUE, 1, 0) -> (→"shooted_ positions":bool[][])
  n1126 = local write "Shoot duration"(600.0) -> ()
  n1127 = local write "Shoot at Scan#"(1) -> ()
  n1128 = local write "is_single_shoot"(TRUE) -> ()
  n1129 = property on="Position to add" class="NumNb (strict)"("DisabledEnum"=w16) -> ()  [unwired: 2 in, 2 out]
  n1130 = property on="ADD ALL\nPositions" class="Bool (strict)"("DisabledEnum"=w16) -> ()  [unwired: 2 in, 2 out]
  n1131 = property on="ADD\nPosition" class="Bool (strict)"("DisabledEnum"=w16) -> ()  [unwired: 2 in, 2 out]
  n1132 = property on="is_single_shoot" class="Bool (strict)"("DisabledEnum"=w16) -> ()  [unwired: 2 in, 2 out]
  n1133 = property on="Shoot duration" class="NumNb (strict)"("DisabledEnum"=w16) -> ()  [unwired: 2 in, 2 out]
  n1134 = property on="RESET POS" class="Bool (strict)"("DisabledEnum"=w16) -> ()  [unwired: 2 in, 2 out]
  n1135 = local write "useLASER_TL"(FALSE) -> ()
  n1136 = property on="Shoot at Scan#" class="NumNb (strict)"("DisabledEnum"=w16) -> ()  [unwired: 2 in, 2 out]
  n1137 = property on="Frames between Patterns" class="NumNb (strict)"("DisabledEnum"=w15) -> ()  [unwired: 2 in, 2 out]
  n1138 = property on="Non" class="NumNb (strict)"("DisabledEnum"=w15) -> ()  [unwired: 2 in, 2 out]
  n1139 = property on="Total Number of Patterns" class="NumNb (strict)"("DisabledEnum"=w15) -> ()  [unwired: 2 in, 2 out]
  n1140 = property on="Noff" class="NumNb (strict)"("DisabledEnum"=w15) -> ()  [unwired: 2 in, 2 out]
  n1141 = property on="Nstart" class="NumNb (strict)"("DisabledEnum"=w15) -> ()  [unwired: 2 in, 2 out]
  n1142 = local write "useFLUIDICS_TL"(FALSE) -> ()
  n1143 = property on="Non FLUIDICS" class="NumNb (strict)"("DisabledEnum"=w24) -> ()  [unwired: 2 in, 2 out]
  n1144 = property on="Noff FLUIDICS" class="NumNb (strict)"("DisabledEnum"=w24) -> ()  [unwired: 2 in, 2 out]
  n1145 = property on="Nstart FLUIDICS" class="NumNb (strict)"("DisabledEnum"=w24) -> ()  [unwired: 2 in, 2 out]
  n1146 = call <userlib>:"tm_stopcapture.vi"("error in (no error)"=w153, "Handle in"=w154) -> ("error out"=w148:errorcluster, "Handle out"=w149:u32)  [unwired: 8 out]
  n1147 = call <userlib>:"tm_unpreparecapture.vi"("error in (no error)"=w148, "Handle in"=w149) -> ("error out"=w151:errorcluster, "Handle out"=w150:u32)  [unwired: 8 in]
  n1148 = call "SerialDisconnect.vi"("error in (no error)"=w97, "VISA resource name"=w98) -> ()  [unwired: 1 in, 1 out]
  n1149 = call <userlib>:"tm_closecamera.vi"("error in (no error)"=w151, "Handle in"=w150) -> ("error out"=w156:errorcluster)  [unwired: 9 out]
  n1150 = Close Reference(reference=w114, error in (no error)=w87) -> ()  [unwired: 1 out]
  n1151 = local write "Ready"(w134) -> ()
  n1152 = call <userlib>:"tm_deinitialize.vi"("error in (no error)"=w156) -> ()  [unwired: 11 out]
  "Recorded\nPatterns" <- w58
  "SavedImages" <- w132
  "Next Pattern" <- w59
  "Recorded Scans" <- w58
  "Next Scan" <- w59
  "TL_NCAN" <- u8 0
  "TL_NPOS" <- w56
  "Current Position" <- w56
  "softversion" <- "V4"
